vi "UHR-Fleezers Control (host) - 9.3.vi"() -> ()   [LabVIEW 2009]
uses:
  <vilib>/Utility/miscctls.llb/LVPoint32TypeDef.ctl
  <vilib>/Utility/miscctls.llb/LVMinMaxIncTypeDef.ctl
  <vilib>/userDefined/High Color/nirio_resource_hc.ctl
  <vilib>/Instr/_visa.llb/VISA Configure Serial Port (Instr).vi
  <vilib>/Platform/TimedLoop/XDataNode/XDataNode.xnode
  <vilib>/Platform/TimedLoop/XDataNode/loadlvalarms.vi
  <vilib>/Platform/TimedLoop/XDataNode/timing_clust.ctl
  <vilib>/Platform/TimedLoop/XDataNode/nitl_modes.ctl
  <vilib>/Platform/TimedLoop/XDataNode/wakeup.ctl
  <vilib>/rvi/interface/nirviOpenFPGA/nirviOpenFPGA.xnode
  FPGA Bitfiles/UHR-Fleezers Instr~3C_FPGA Target_UHR-Fleezers Contr~C3.lvbitx
  UHR-Fleezers Control (fpga) - 9.2.vi
  <vilib>/FPGAPlugInAG/PCIe-7852R/nirviIntfOpen_PCIe-7852R.vi
  <vilib>/rvi/interface/nirviMethod/nirviMethod.xnode
  <vilib>/Utility/error.llb/Merge Errors.vi
  <vilib>/LabVIEW Targets/FPGA/Rio/nirio_HostInterface/nirio_Reset.vi
  <vilib>/LabVIEW Targets/FPGA/Rio/nirio_HostInterface/nirio_DMAStopAll.vi
  <vilib>/rvi/interface/common/niFpgaNodeNameForErrorReporting.ctl
  <vilib>/rvi/errors/niLvFpgaWhatHappensToTopLevelVI.ctl
  <vilib>/LabVIEW Targets/FPGA/Rio/nirio_HostInterface/nirio_DisableInterrupts.vi
  <vilib>/Utility/error.llb/Error Cluster From Error Code.vi
  <vilib>/rvi/errors/niLvFpgaAdjustHostInterfaceError.vi
  <vilib>/rvi/interface/nirviReadWriteControl/nirviReadWriteControl.xnode
  <vilib>/LabVIEW Targets/FPGA/Rio/nirio_HostInterface/nirio_WriteBig.vi
  <vilib>/LabVIEW Targets/FPGA/Rio/nirio_HostInterface/nirio_DMAConfigure.vi
  <vilib>/LabVIEW Targets/FPGA/Rio/nirio_HostInterface/nirio_DMAStop.vi
  <vilib>/RVI Host/nirviSupport.llb/nirviErrorClusterFromErrorCode.vi
  <vilib>/LabVIEW Targets/FPGA/Rio/nirio_HostInterface/nirio_EnableInterrupts.vi
  <vilib>/rvi/errors/niLvFpgaReportInternalErrorWithAdditionalInfo.vi
  <vilib>/express/express analysis/Spectral/XNode/ExpressSpectralMeasurementsBlockNode.xnode
  <vilib>/express/express analysis/Spectral/Block/exnSpectralBlock spectral measurements PSD poly.vi
  <vilib>/express/express analysis/Spectral/Block/exnSpectralBlock spectral measurements PSD WFM.vi
  <vilib>/Waveform/WDTOps.llb/WDT Append Waveforms DBL.vi
  <vilib>/LabVIEW Targets/FPGA/Rio/nirio_HostInterface/nirio_ReadBig.vi
  <vilib>/vision/Avi1.llb/AviRefnum.ctl
  <vilib>/rvi/interface/nirviCloseFPGA/nirviCloseFPGA.xnode
  <vilib>/FPGAPlugInAG/PCIe-7852R/nirviIntfClose_PCIe-7852R.vi
  <vilib>/Analysis/NI_AALBase.lvlib
  <vilib>/Platform/TimedLoop/XDataNode/XDNodeRunTimeDep.lvlib
  openfpgaref.8.6.ctl
  NiRioSrv.dll
  <vilib>/vision/NI_Vision_Development_Module.lvlib
panel:
  in  "Force Reset":bool
  in  "Force Yank":bool
  in  "Random Choice":bool=TRUE
  in  "N Array El":u8=3 min=1 step=1
  in  "Yank to Delta Array (MHz)":dbl[](array[numeric])=[16.3, 15.85, 14.85]
  in  "Yank Delay (s)":dbl=3.5
  in  "N pts to average":u16=6
  out "Fl. High":bool
  out "Waiting":bool
  in  "Fl. Delta Thresh. (kHz)":dbl=0.6
  in  "Fl. Triggered...":bool
  in  "Action":string(combo)="Yank"
  out "Duration (s)":dbl
  out "Waveform Graph":dbl[](graph) caption="APD Line Scan"
  in  "Total Volume\nFlushed (uL)":dbl
  in  "Flush Center Channel":bool
  in  "Inject Pump 3 (D)":bool
  in  "Inject Pump 1 (DNA)":bool
  out "Messages":string
  in  "APD Ave N":dbl=10.0
  out "Int. Time (s)":dbl
  in  "Stop All":bool
  out "sigma/mean":dbl
  out "Rate sigma (Hz)":dbl format="%0.2f"
  out "Current Stage  Position":cluster{dbl, dbl, dbl}
  in  "Index":dbl=1.0 caption="Save File Index" min=1.0 step=1.0
  in  "Tab Control 6":T1(tab)=enum."Dual Display (Trap + APD)"
  out "All Signals":waveform(dbl)[](graph)
  in  "Signals to Plot":i32(listbox)
  out "Trap Disp. Freq. (Hz)":dbl caption="Freq. (Hz)" format="%#_6p"
  out "Display Period (s)":dbl caption="Period (s)" format="%#_6p"
  in  "Trap Disp. Downsample":dbl=20000.0 caption="Downsample"
  in  "APD Disp. Scale":dbl=0.1 caption="Scale (Divide,\nfor above plot only)"
  in  "APD Disp. Downsample":dbl=30.0 caption="Integrate" min=1.0 step=1.0
  out "APD Display Freq. (Hz)":dbl caption="Freq. (Hz)"
  out "APD Display Period (s)":dbl caption="Period (s)"
  out "RMS (Ang)":dbl format="%_2g"
  in  "Bead Sep. Int. Time (s)":dbl=5.0 caption="Int. Time (s)"
  in  "Below (kHz)":dbl=0.5
  in  "Above (kHz)":dbl=2.0
  in  "Adjust Scale\nto Mean":bool
  in  "Rescale on Mean":bool
  in  "Offset (nm)":dbl
  out "Mean":dbl caption="Mean (pN)" format="%#_3g"
  out "Force":waveform(dbl)[](graph)
  out "APD 1 Chart":waveform(dbl)(graph)
  in  "Calibration":u16(ring)=2 items=["None", "Position", "Force"]
  out "T1 X":dbl caption="T1 X (pN)" format="%0.2f"
  out "T2 X":dbl caption="T2 X (pN)" format="%0.2f"
  out "Bead Separation":waveform(dbl)(graph)
  in  "Amplitude (nm)":dbl=1.0
  out "Bead Mean (nm)":dbl caption="Mean (nm)" format="%0.2f"
  out "Difference":dbl caption="Difference (pN)" format="%.2g"
  out "APD 1 Graph":dbl[](graph) caption="Most Recent Time Trace"
  out "Trap Delta Graph":dbl[](graph) caption="Most Recent Time Trace"
  out "size(s) APD array":i32
  out "size(s) of 1 acq array":i32
  out "Delta Fl. (Hz)":dbl
  out "APD 1 Graph 2":dbl[](graph) caption="Most Recent Time Trace"
  in  "Flip Green Filter":bool
  in  "Set X Only":bool
  in  "Set Y Only":bool
  out "Detection Laser X":T2(plugin-control)
  out "APD 1":T2(plugin-control)
  out "Detection Laser Y":T2(plugin-control)
  out "Pointer Y (V)":dbl format="%_3g"
  out "Pointer X (V)":dbl format="%_3g"
  in  "Set Confocal Spot (X-Y)":bool
  out "FFT 1":cluster{"f0":dbl, "df":dbl, "magnitude":dbl[]}[](graph)
  out "FFT 2":cluster{"f0":dbl, "df":dbl, "magnitude":dbl[]}[](graph)
  in  "FFT 1 Choice 1":u16(ring) items=["T1 Y", "T1 X", "T1 Sum", "T2 Y", "T2 X", "T2 Sum", "T1 FB X", "T1 FB Sum", "T2 FB X", "T2 FB Sum", "PSD Y", "PSD X", "PSD Y Sum", "none"]
  in  "FFT 2 Choice 1":u16(ring)=13 items=["T1 Y", "T1 X", "T1 Sum", "T2 Y", "T2 X", "T2 Sum", "T1 FB X", "T1 FB Sum", "T2 FB X", "T2 FB Sum", "PSD Y", "PSD X", "PSD Y Sum", "none"]
  in  "FFT 1 Choice 2":u16(ring)=1 items=["T1 Y", "T1 X", "T1 Sum", "T2 Y", "T2 X", "T2 Sum", "T1 FB X", "T1 FB Sum", "T2 FB X", "T2 FB Sum", "PSD Y", "PSD X", "PSD Y Sum", "none"]
  in  "FFT 2 Choice 2":u16(ring)=13 items=["T1 Y", "T1 X", "T1 Sum", "T2 Y", "T2 X", "T2 Sum", "T1 FB X", "T1 FB Sum", "T2 FB X", "T2 FB Sum", "PSD Y", "PSD X", "PSD Y Sum", "none"]
  in  "Compute FFT":bool
  in  "Reset FFT":bool
  in  "# Spectra to Ave.":dbl=100.0
  out "Ave. Time (s)":dbl
  out "1 Channel":waveform(dbl)(graph)
  out "Slow mean":dbl format="%0.2f"
  in  "Slow mean N ave.":dbl=1.0 min=1.0 step=1.0
  out "Mean Intensity":dbl
  out "Sigma":dbl
  out "Sigma/Mean":dbl
  in  "Subtract mean":bool
  in  "High Res. Display":u16(ring) items=["T1 Y", "T1 X", "T1 Sum", "T2 Y", "T2 X", "T2 Sum", "T1 FB X", "T1 FB Sum", "T2 FB X", "T2 FB Sum", "PSD Y", "PSD X", "PSD Y Sum"]
  out "APD 1 Rate (Hz)":dbl format="%#_3p"
  out "Image":u32[][](graph)
  in  "Tab Control":T3(tab)=enum."Trap Control (RF)"
  in  "Lower Ch. Cap.":bool
  in  "With\nOffset":bool
  in  "Read Cal":bool
  out "Tether":bool
  in  "Tether Alarm?":bool=TRUE
  in  "Move to Delta (MHz)":dbl=14.85
  in  "Then...":string(combo)="4"
  in  "Data Acq. Spot":bool
  in  "Confocal Linescan":bool
  in  "Speed (nm/s)":dbl=100.0
  in  "Stop F (pN)":dbl=3.0
  in  "Furthest Withdraw (MHz)":dbl=15.0
  in  "Closest Delta (MHz)":dbl=10.25 step=0.25
  in  "Fish for Tether":bool
  in  "Confocal Image":bool
  in  "Round T1 X":bool caption="Round"
  in  "T1 offset_x (mV)":dbl=-26.302542012392074 format="%#_2g"
  in  "T1 kappa_x (pN/nm)":dbl=0.22546432407642192 min=0.0 step=0.001 format="%#_2g"
  out "Time (s)":dbl
  out "Total Time (s)":dbl
  in  "Start Saving":bool
  in  "Limits Enable":bool=TRUE caption="Enable"
  in  "Limit Max (MHz)":dbl=16.0 caption="Max (MHz)"
  in  "Limit Min (MHz)":dbl=10.0 caption="Min (MHz)"
  in  "Cal sets to save":u32=50 min=1 step=1
  in  "Comment (data description)":string="testing confocal setup"
  out "Calibrating Trap...":bool
  in  "Trap 2 (ON/OFF)":bool
  in  "Trap 1 (ON/OFF)":bool
  in  "Save Calibration":bool
  in  "N sets to save":u32=200 caption="N Sets"
  in  "Save N Sets":bool
  out "Save file name":path
  in  "Save ave N":dbl=500.0 caption="Averaging Factor"
  out "Saving...":bool
  in  "Stop Saving":bool
  out "Progress":u16(slide) scale=0.0..100.0
  out "Manipulating Trap":bool
  out "Buffer Status":dbl(slide) scale=0.0..1.0
  out "Overflow (data lost)":bool
  in  "Reset":bool
  out "Data Rate (Hz)":dbl caption="Trap Data Rate (Hz)" format="%#_3p"
  out "Data Period (s)":dbl caption="Trap Data Period (s)" format="%#_6p"
  out "Save Data Rate (Hz)":dbl caption="Rate (Hz)" format="%#_6p"
  out "Save Data Period (s)":dbl caption="Period (s)" format="%#_6p"
  in  "T1 alpha_x (nm/V)":dbl=630.439304367558 step=10.0 format="%#_3g"
  in  "T2 alpha_x (nm/V)":dbl=704.7738222964198 step=10.0 format="%#_3g"
  in  "T2 kappa_x (pN/nm)":dbl=0.2030110880477556 min=0.0 step=0.001 format="%#_2g"
  in  "T2 offset_x (mV)":dbl=-26.67973517613748 format="%#_2g"
  in  "BD 1 Frequency 1 (MHz)":dbl=70.15 caption="T1 X (MHz)" min=60.0 max=90.0 step=1.0 format="%#_6p"
  in  "BD 1 Frequency 2 (MHz)":dbl=85.0 caption="T2 X (MHz)" min=60.0 max=90.0 step=1.0 format="%#_6p"
  in  "Green Laser ON/Interlacing":bool
  in  "Round T2 X":bool caption="Round"
  in  "AO1":dbl(slide)=5.61 caption="Confocal Y (V)" min=0.0 max=10.0 step=0.01 scale=0.0..10.0 scale format="%_1f"
  in  "AO2":dbl(slide)=3.9 caption="Confocal X (V)" min=0.0 max=10.0 step=0.01 scale=0.0..10.0 scale format="%_1f"
  in  "Upper Cap.":bool
  in  "Lower Cap.":bool
  in  "Trap Raster Scan":bool
  out "Raster Scanning...":bool
  in  "Trap Delta (MHz)":dbl=14.85
  in  "Dump Beads":bool
  out "Stage Moving":bool
  in  "Wait Before Save (s)":u32=1
  out "Attempts":dbl
  in  "Attempt Limit":dbl=30.0 caption="Limit"
  in  "Array":dbl[][](array[numeric])
  in  "Move to Position 5":bool
  in  "Position 5 Label":string="Lower channel capillary"
  in  "z nudge increment (um)":dbl=0.5
  in  "+z":bool
  in  "Saved Stage Positions":T4={"Position 1"={1.04712, -0.65049, 0.0}, "Position 2"={0.0, 0.0, 0.0}, "Position 3"={2.99364, -0.33706, 0.0}, "Position 4"={2.1058, 0.57485, 0.0}, "Position 5"={3.01039, 3.32514, 0.03555}} {"Position 5"."?" min=-0.1 max=0.1 step=0.1; "Position 1"."?" min=-0.1 max=0.1 step=0.1; "Position 2"."?" min=-0.1 max=0.1 step=0.1; "Position 3"."?" min=-0.1 max=0.1 step=0.1; "Position 4"."?" min=-0.1 max=0.1 step=0.1}
  in  "Position 1 Label":string="Upper capillary"
  in  "Set Position 1":bool
  in  "Set Position 2":bool
  in  "Set Position 3":bool
  in  "Set Position 4":bool
  in  "Move to Position 3":bool
  in  "Move to Position 4":bool
  in  "Move to Position 2":bool
  in  "Move to Position 1":bool
  in  "Position 2 Label":string="Lower capillary"
  in  "Position 3 Label":string="Measurement spot"
  in  "Position 4 Label":string="Dump beads"
  in  "-z":bool
  in  "Set Position 5":bool
  in  "Top Ch Inject Rate (ul/h)":dbl=10.0
  in  "Pump write delay (ms)":dbl=300.0
  in  "All Pump Parameters":T5={"Pump 1"={"Diameter (mm)"=4.61, "Units"=3.0, "Volume"=0.0, "Rate"=0.0}, "Pump 2"={"Diameter (mm)"=4.61, "Units"=3.0, "Volume"=0.0, "Rate"=0.0}, "Pump 3"={"Diameter (mm)"=4.61, "Units"=3.0, "Volume"=0.0, "Rate"=0.0}}
  in  "Top Ch Inject Volume (uL)":dbl=100.0
  in  "Pump pause delay (ms)":u32
  in  "Bottom Ch Inject Volume (uL)":dbl=100.0
  in  "Bottom Ch Inject Rate (ul/h)":dbl=10.0
  in  "Flush Center Ch Volume (uL)":dbl=15.0
  in  "Flush Center Ch Rate (ul/m)":dbl=100.0
  in  "Tab Control 2":T6(tab)=enum."AOD Raster Scan"
  out "Total Counts (ticks)":u32
  in  "Trap ON/OFF X or Y Amp?":bool=TRUE
  in  "Oscillate Set 1":bool
  in  "Trap 1 ON":bool
  in  "Number Interlace Sets":u8=3 min=1 max=3
  in  "DIO count 3 (ticks)":u32=200
  in  "DIO count 2 (ticks)":u32=200
  in  "DIO count 1 (ticks)":u32=200
  in  "BD 2 Amplitude 3 (%)":dbl min=0.0 max=50.0 step=1.0
  in  "BD 2 Amplitude 2 (%)":dbl min=0.0 max=50.0 step=1.0
  in  "BD 2 Amplitude 1 (%)":dbl min=0.0 max=50.0 step=1.0
  in  "BD 1 Amplitude 3 (%)":dbl min=0.0 max=50.0 step=1.0
  in  "BD 1 Amplitude 2 (%)":dbl=35.0 min=0.0 max=50.0 step=1.0
  in  "BD 1 Amplitude 1 (%)":dbl=10.0 min=0.0 max=50.0 step=1.0
  in  "BD 2 Frequency 3 (MHz)":dbl=26.0 min=0.0 max=40.0 step=1.0 format="%#_6p"
  in  "BD 1 Frequency 3 (MHz)":dbl=70.0 min=60.0 max=90.0 step=1.0 format="%#_6p"
  in  "BD 2 Frequency 2 (MHz)":dbl=26.0 min=0.0 max=40.0 step=1.0 format="%#_6p"
  in  "BD 2 Frequency 1 (MHz)":dbl=26.0 min=0.0 max=40.0 step=1.0 format="%#_6p"
  in  "Not-Interlacing Set":enum32{"Set 1", "Set 2", "Set 3"}(radio)
  in  "Interlace":bool=TRUE
  in  "Trap 2 ON":bool
  in  "Trap 3 ON":bool
  in  "Scan axis 2":bool=TRUE
  in  "Osc. freq. (Hz)":dbl=0.25
  in  "Osc. amp. (MHz)":dbl=2.0
  out "Coords":T7
  in  "Manipulation Scaling":cluster{"Horizontal":dbl, "Vertical":dbl}={"Horizontal"=0.075, "Vertical"=0.01}
  in  "Freq or Amp switch first":bool=TRUE
  in  "Swap F1 and F2":bool
  in  "Freq switch delay":u16
  in  "Amp switch delay":u16=5
  in  "MCL Step Increment (V_int)":dbl=3.0
  out "Time to Finish All (min)":dbl format="%#_2p"
  in  "Scan Speed (nm/s)":dbl=100.0
  in  "Scan Range (nm)":dbl=200.0
  in  "Step Size (nm)":dbl=1.0
  in  "MCL/AOM Scale Tweak":dbl=1.0
  in  "MCL Step Position Ratio":dbl=0.5
  in  "Move MCL Also?":bool=TRUE
  out "Final sep (nm)":dbl
  out "Initial sep (nm)":dbl
  out "Save index":dbl
  out "Final delta (MHz)":dbl
  out "Initial delta (MHz)":dbl
  out "Final freq. (MHz)":dbl
  out "Initial freq. (MHz)":dbl
  in  "Saved AOD Raster Scan Parameter Sets":T8(array[cluster])=[{"Scan Range AOD (nm) 2"=500.0, "Step Size AOD (nm) 2"=1.0, "Scan Speed AOD (nm/s) 2"=200.0, "Number of scans (AOD) 2"=1, "Label"=""}, {"Scan Range AOD (nm) 2"=1000.0, "Step Size AOD (nm) 2"=1.0, "Scan Speed AOD (nm/s) 2"=200.0, "Number of scans (AOD) 2"=5, "Label"="wide offset scan"}, {"Scan Range AOD (nm) 2"=20.0, "Step Size AOD (nm) 2"=0.68, "Scan Speed AOD (nm/s) 2"=0.68, "Number of scans (AOD) 2"=1, "Label"="2 bp steps"}]
  in  "Load parameters":bool
  out "Scan Range (MHz)":dbl=10.0
  in  "Restart DMA? (AOD)":bool=TRUE caption="Restart DMA?"
  out "Incr. int (AOD)":i64
  out "Time/Scan (s) (AOD)":dbl format="%#_2p"
  out "Data points/scans":dbl
  out "Data points/scan (f/b)":dbl
  in  "Save scans":bool=TRUE
  out "AOD Scan I":u64 caption="Scan I"
  in  "Continuous AOD Scanning":bool caption="Continuous Scanning"
  in  "Abort AOD Scan":bool caption="Abort Scan"
  in  "Scan BD":bool=TRUE
  out "Cycles/step (AOD)":u64=400 format="%.0p"
  in  "Number of F/B Scans (AOD)":u16=3 min=1
  out "Scan steps (AOD)":u64=1000
  out "Scan Increment (MHz)":dbl=0.2
  out "AOD Scanning":bool caption="Scanning"
  in  "Start AOD Scan":bool caption="Start Scan"
  out "N sets should be saved":dbl
  out "Progress 2":u16(slide) caption="Progress" scale=0.0..100.0
  in  "Abort save 2":bool caption="Abort save"
  in  "Trap 1 Bead Size (nm)":dbl=860.0
  in  "Trap 2 Bead Size (nm)":dbl=790.0
  out "MCL Count":dbl
  in  "All FB On/Off":bool=TRUE
  in  "AI2 to Setpoint":cluster{"Set 1":bool, "Set 2":bool}
  out "AI2 (V)":cluster{"Set 1":dbl, "Set 2":dbl}
  in  "Reset Feedback":cluster{"Set 1":bool, "Set 2":bool}
  in  "PID Gains":T9={"Set 1"={"proportional gain (Kc)"=0, "integral gain (Kc*Ts/Ti)"=5, "derivative gain (Kc*Td/Ts)"=0}, "Set 2"={"proportional gain (Kc)"=0, "integral gain (Kc*Ts/Ti)"=5, "derivative gain (Kc*Td/Ts)"=0}}
  in  "Setpoints (V)":cluster{"Set 1":dbl, "Set 2":dbl}={"Set 1"=9.0, "Set 2"=9.0}
  in  "Feedback On/Off":cluster{"Set 1":bool, "Set 2":bool}={"Set 1"=TRUE, "Set 2"=TRUE}
  in  "Tab Control 3":enum32{"Timing", "MCL Scan", "Analog Out"}(tab)=enum."MCL Scan"
  out "APD Gate Late Counter":u32
  in  "- phase (APD Gate)":bool
  in  "+ phase (APD Gate)":bool
  out "APD Gate Relative Phase":i16
  in  "Phase Adj. (APD Gate)":i16=20
  in  "Initial Phase Adjustment (APD Gate)":i16=50
  in  "Save APD Data\nwith Trap Data":bool=TRUE
  out "APD FIFO Elements Remaining":u32
  in  "- phase (APD Acq)":bool
  in  "+ phase (APD Acq)":bool
  out "APD Acq Late Counter":u32
  out "APD Acq Relative Phase":i16
  in  "Phase Adj. (APD Acq)":i16=20
  in  "Initial Phase Adjustment (APD Acq)":i16
  in  "Invert APD Gate":bool caption="Invert Gate"
  in  "APD Gate OFF Count":u32=450 caption="Gate OFF Count"
  in  "APD Gate ON Count":u32=150 caption="Gate ON Count"
  in  "APD Gate":enum32{"ON", "OFF", "Interlace"}(radio)=enum."Interlace"
  in  "APD Integration Time (s)":dbl=0.01 caption="Integration Time (s)"
  out "APD Acq Rate (Hz)":dbl=20000000.0 caption="Rate (Hz)"
  out "APD Samples/FIFO Acq.":dbl
  out "APD Elements/DMA read":u32
  out "APD Int. Count":u32 format="%.0p"
  in  "Tab Control 5":enum32{"PSD X", "PSD Y", "Other Data Channel"}(tab)
  out "Data map":dbl[][](graph)
  in  "Channel":i32=4
  in  "Abort MCL Scan":bool
  out "MCL Scan I":u64
  out "MCL Scanning":bool
  in  "Start MCL Scan":bool
  out "wait to reset values":bool
  in  "Tab Control 4":enum32{"Scan Settings", "MCL FPGA Loop Timing"}(tab)
  out "Total Time (s)":dbl
  in  "Scan lines (y)":u64=20
  in  "Fast Scan Dir":bool=TRUE
  in  "2D or 1D Scan":bool=TRUE
  out "Initial X":dbl
  out "Initial Y":dbl
  out "Time/f+b scan (s) (MCL)":dbl caption="Time/scan (s)"
  in  "Number of scans (MCL)":u64=1 caption="Scans"
  in  "Scan steps (MCL)":u64=40 caption="Scan steps (x)"
  in  "N APD Samp/step":dbl=3.0
  in  "Scan Range (V)\n(of steps)":dbl=3.5
  in  "Restart DMA? (MCL)":bool=TRUE caption="Restart DMA?"
  in  "Continuous MCL Scanning":bool caption="Cont. Scanning"
  in  "Center Scan":bool=TRUE
  in  "Save Data (MCL)":bool=TRUE caption="Save Data"
  out "Actual Incr. int (MCL)":i16 caption="Incr. int"
  out "Desired incr (int)":dbl
  out "Desired Scan Incr (V)":dbl
  out "N sets should be saved (MCL)":dbl caption="N sets should be saved"
  out "Data points/scans (MCL)":dbl caption="Data points/scans"
  out "Data points/scan (f+b)":dbl caption="points/scan (f+b)"
  out "Cycles/step (MCL)":u64 caption="Cycles/step" format="%.0p"
  out "Actual MCL Inc (V)":dbl
  in  "Phase adjust (MCL)":i16 caption="Phase adjust"
  out "Relative Phase (MCL)":i16 caption="Relative Phase"
  in  "Initial Phase Adj. (MCL)":i16 caption="Initial Phase Adj."
  in  "Update Count (MCL)":u32=600
  in  "+ phase (MCL)":bool
  in  "- phase (MCL)":bool
  out "MCL Late Counter":u32
  in  "APD 1 AO Mult.":i16=1 min=1
  in  "APD 2 AO Mult.":i16=1 min=1
  in  "APD 1 AO offset":i16
  in  "APD 2 AO offset":i16
  in  "Tab Control 7":enum32{"Green FB Signals", "Slow MCL Scan"}(tab)
  out "Green FB Plot":dbl(graph)
  out "MCL Scan 2":cluster{"Begin (V)":dbl, dbl, dbl[]}(graph)
  out "MCL Scan":cluster{"Begin (V)":dbl, dbl, dbl[]}(graph)
  in  "Green laser mode":enum32{"Laser ON", "Laser OFF", "Interlace"}(radio)=enum."Interlace"
  in  "GI Frequency, ON count":u32=150 min=1 step=1
  in  "Invert GI":bool
  out "GI Late Counter":u32
  in  "Phase adj. (GI)":i16=5
  out "GI relative phase":i16
  in  "+ phase (GI)":bool
  in  "Initial Phase Adjustment (GI)":i16=15
  in  "GI Frequency, OFF count":u32=450 min=1 step=1
  in  "- phase (GI)":bool
  out "Green FB Signals (V)":cluster{"Y":dbl, "X":dbl, "Sum":dbl}
  out "Relative phase (Green FB)":i16
  in  "+ phase (Green FB)":bool
  in  "- phase (Green FB)":bool
  in  "Green FB Count":u32=600
  in  "Phase adj. (Green FB)":i16=10
  in  "Initial Phase Adjustment (Green FB)":i16=50
  in  "Green FB On/Off":bool=TRUE
  in  "Current When FB OFF (%)":dbl=87.0 min=0.0 max=100.0 step=1.0
  in  "Green int current ON count adj":u32=150
  in  "Green FB Gains":T10={"proportional gain (Kc)"=10, "integral gain (Kc*Ts/Ti)"=5, "derivative gain (Kc*Td/Ts)"=0}
  in  "Green FB Setpoint (mV)":dbl=100.0
  in  "- phase (GI) 2":bool
  in  "Initial Phase Adjustment (GI) 2":i16=-100
  in  "+ phase (GI) 2":bool
  out "GI relative phase 2":i16
  in  "Phase adj. (GI) 2":i16=20
  out "GI Late Counter 2":u32
  in  "# Samples/trap":dbl=20000.0 format="%#_6p"
  out "Elements/DMA read":u32 format="%.0p"
  out "Ave. Rate (Hz)":dbl format="%#_6p"
  out "FIFO El. Rem.":u32 format="%.0p"
  in  "Phase adj. (AI1)":i16=15
  out "Relative phase (AI1)":i16
  in  "+ phase (AI1)":bool
  in  "- phase (AI1)":bool
  out "Late Counter (AI1)":u32
  in  "Initial Phase Adjustment (AI1)":i16=220
  out "AI rate (Hz)":dbl=50000.0 format="%#_6p"
  in  "AI Count (ticks)":u32=200
  out "# Samples/channel":u32=20000 format="%.0p"
  in  "FIFO Depth":u32=600000 format="%.0p"
  in  "Detector Type":string(combo)="IR-QPD + PSD + FB-QPD X position"
  in  "N Acq Sets (Traps + Fl.)":i16=3
  in  "Sets to FIFO (Traps)":T11={"Set 1"=TRUE, "Set 2"=TRUE, "Set 3"=FALSE}
  in  "FPGA Ave.":dbl=1.0 min=1.0 step=1.0
  out "Ave. Period (s)":dbl format="%#_6p"
  out "DMA Update Period (s)":dbl
  out "FPGA Averaging":bool
  out "Trap Sets":i16
  out "Counts/DMA":dbl format="%#_6p"
  in  "Video Capture Rate (Hz)":dbl=30.0
  in  "Video Index":dbl=1.0 min=1.0 step=1.0
  in  "New Video File":bool
  in  "Capture Video":bool
  in  "Reset Averaging":bool
  in  "Averaging":bool
  in  "Capture and Save Image":bool
  in  "Image Index":dbl=1.0 min=1.0
  out "Path Out":path
  in  "Center Point":cluster{"X":i32, "Y":i32}={"X"=335, "Y"=271}
  in  "Zoom Factor":sgl=7.0
  out "Window Size":cluster{"Width":i32, "Height":i32}
  out "Window Position":cluster{"X Position":i32, "Y Position":i32}={"X Position"=40, "Y Position"=40}
  in  "Initial Window Size":cluster{"Width":i32, "Height":i32}={"Width"=884, "Height"=619}
  in  "Initial Window Position":cluster{"X Position":i32, "Y Position":i32}={"X Position"=796, "Y Position"=4}
  in  "Intensity Upper":u8=88
  in  "Intensity Lower":u8=66
  out "error out":errorcluster
  out "error out 2":errorcluster
  in  "Lost Tether Alarm Threshold (pN)":dbl=0.5
  in  "AOM X Cal (nm/MHz)":dbl=123.0
  in  "MCL X Cal (nm/V)":dbl=1070.0
  out "X RF Amplitude Limits (%)":T12={"Minimum"=0.0, "Maximum"=50.0, "Increment"=1.0}
  out "X RF Frequency Limits (MHz)":T12={"Minimum"=60.0, "Maximum"=90.0, "Increment"=1.0}
  out "Y RF Frequency Limits (MHz)":T12={"Minimum"=60.0, "Maximum"=90.0, "Increment"=1.0}
  out "Y RF Amplitude Limits (%)":T12={"Minimum"=0.0, "Maximum"=50.0, "Increment"=1.0}
  in  "Manip. X?":bool=TRUE
  in  "Manip. Y?":bool
  in  "Force Manip Abort":bool
  out "Read cal error":errorcluster
  in  "DAQ Delay (ms)":u32=1000
  in  "Start Scan":bool
  in  "Scan axis":bool=TRUE
  in  "Osc. amp. (V)":dbl=5.0
  in  "Osc. center (V)":dbl=5.0
  in  "Osc. freq. (Hz) 2":dbl=1.0
  in  "MCL Mode":u16(ring) items=["Manual Positioning", "Sinusoidal Wave", "Linear Scan"]
  in  "Begin (V)":dbl
  in  "End (V)":dbl=10.0
  in  "N Points":dbl=20.0
  in  "Delay to Interlace (s)":dbl
  in  "Delayed Interlace Start":bool
  in  "Read Lateness and Rel Phase":bool
  out "Vec Mean of T1 T2":dbl[](array[numeric])
  in  "Cal read wait (s)":u32=5
  out "Time tether formed":timestamp
  in  "Sample Chamber Stage Serial Port":refnum<visa-resource-name>="ChamberStageCOM4"
  in  "Syringe Pump Serial Port":refnum<visa-resource-name>="ChemyxPumpCOM3"
  # "Trap Display:"
  # "APD Display:"
  # "DAQ"
  # "Move Stage and Take Action"
  # "Trap Manipulation"
  # "Data Saving"
  # "Bead Calibration"
  # "Trap Position Difference Limits"
  # "DNA Beads"
  # "ADig Beads"
  # "Center channel"
  # "Units: \n1 = ml/m\n2 = ml/h\n3 = ul/m\n4 = ul/h"
  # "Rate param is ul/h\nVolume param is ul"
  # "X"
  # "Y"
  # "Oscillate Set 1 freq. (debugging)"
  # "BD 1"
  # "BD 2"
  # "AOD Raster Scan"
  # "Approx. trap separations"
  # "X"
  # "Y"
  # "Gate"
  # "X"
  # "2D"
  # "Y"
  # "1D"
  # "Green Laser Interlacing"
  # "Green FB Measurement"
  # "Digital Gate"
  # "Current Analog Control"
  # "Total AI Rates (NOT rates/trap)"
  # "(Samples/trap x Trap Sets)"
  # "(Samples/channel x\n8 if averaging (8 channels)\n4 if no averaging)"
  # "Trap 1"
  # "Trap 2"
  # "Flour./Trap 3"
  # "External Video Window"
  # "MCL Position Debugging"
  # "Temporary Control Storage\n(these used to be somewhere else, still want to keep them)"
  # "Y"
  # "X"
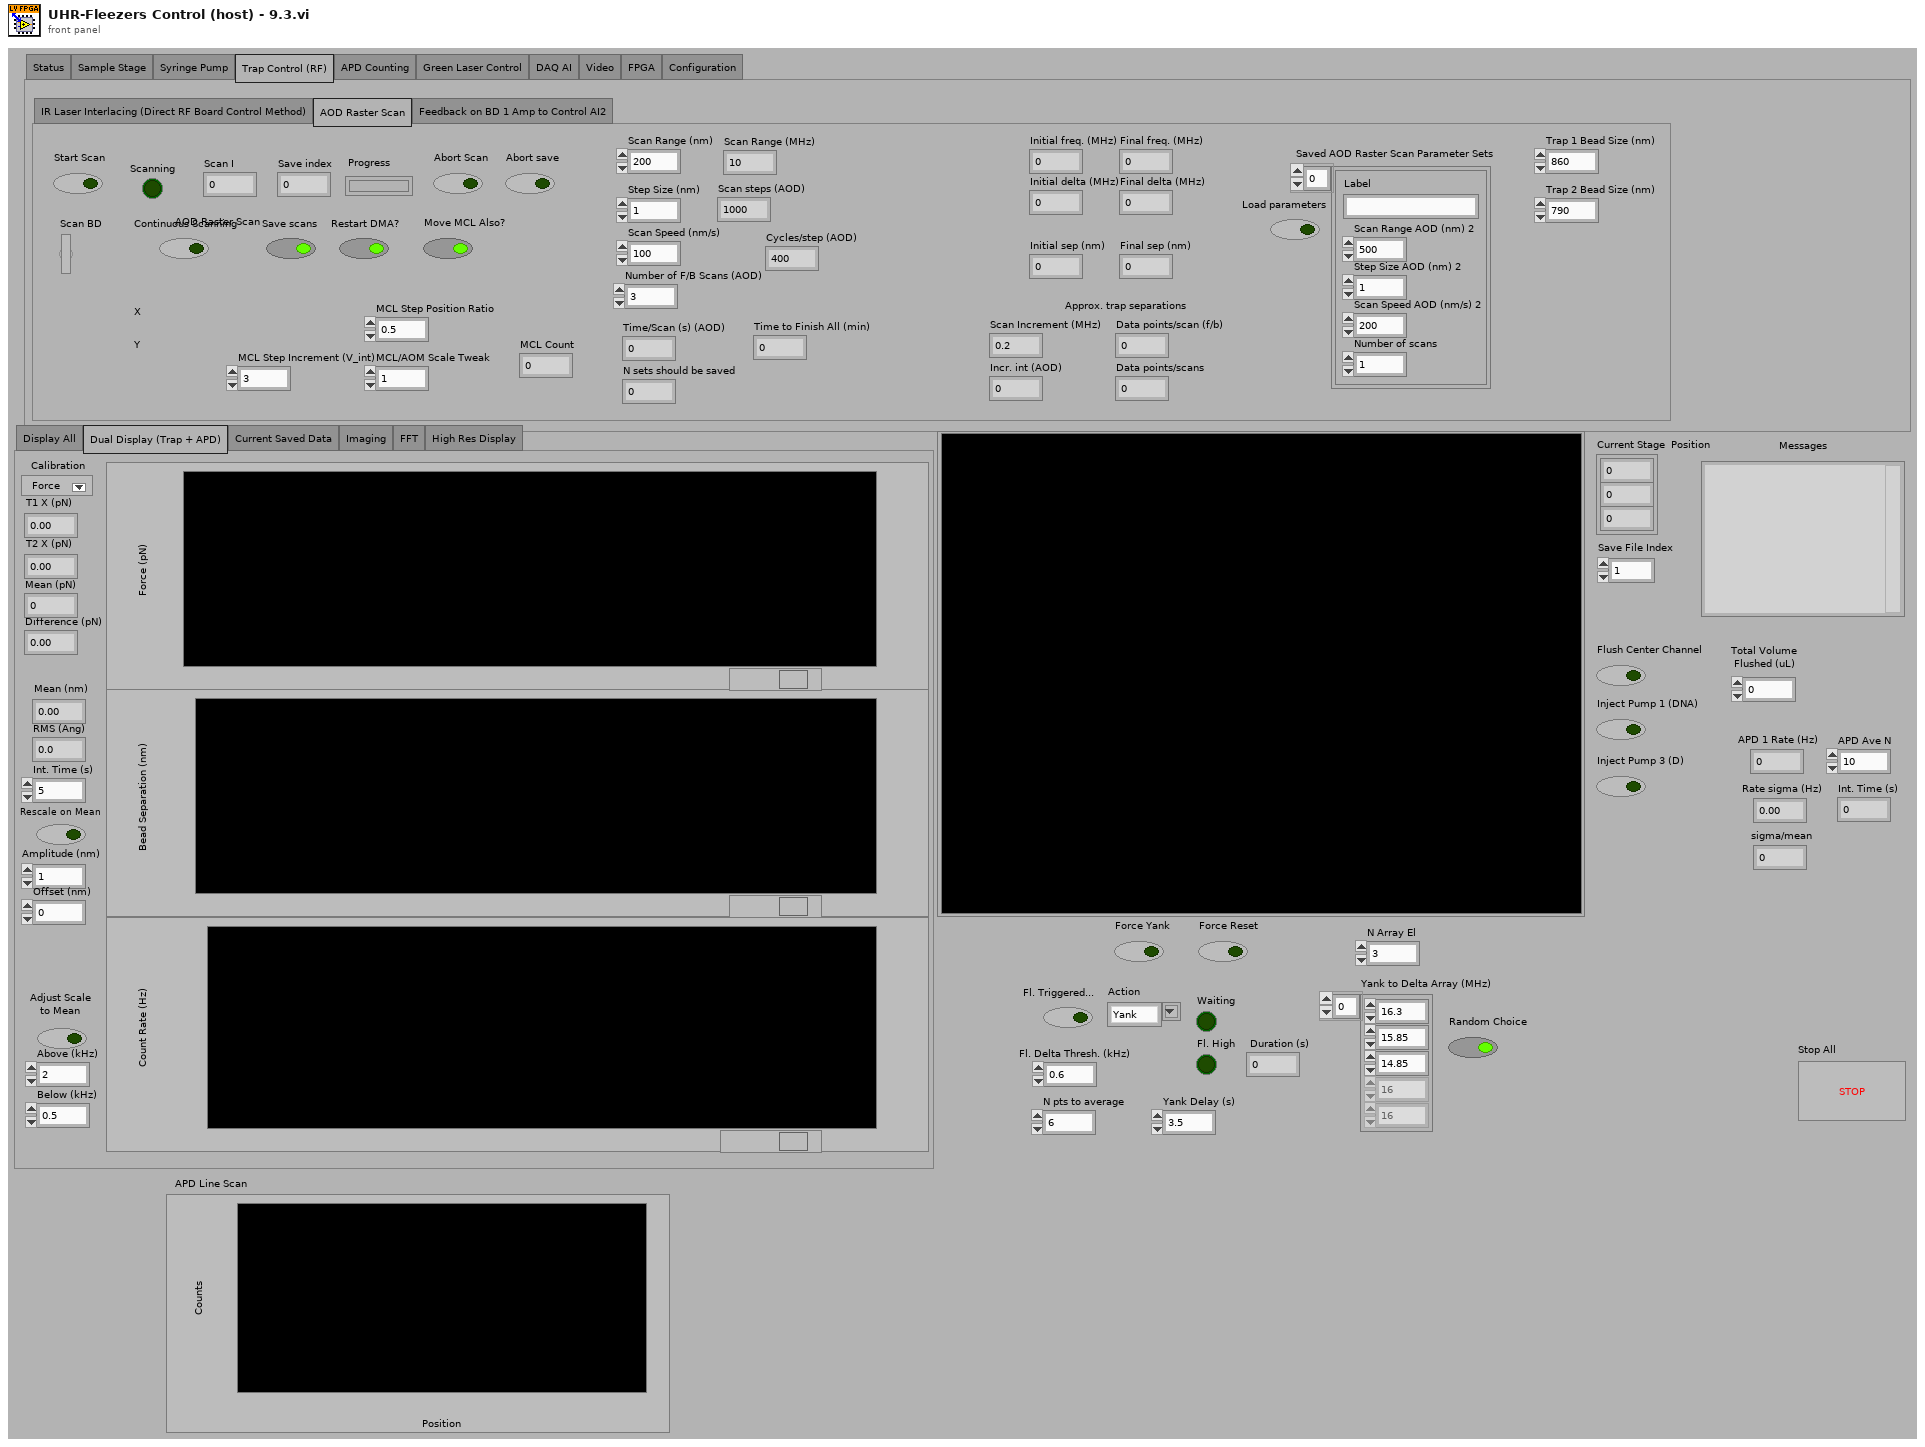
[diagram p1: front panel]
types:
  T1 = enum32{"Display All", "Dual Display (Trap + APD)", "Current Saved Data", "Imaging", "FFT", "High Res Display"}
  T2 = typedef "IMAQ Image.ctl" = refnum<image>
  T3 = enum32{"Status", "Sample Stage", "Syringe Pump", "Trap Control (RF)", "APD Counting", "Green Laser Control", "DAQ AI", "Video", "FPGA", "Configuration"}
  T4 = cluster{"Position 1":cluster{dbl, dbl, dbl}, "Position 2":cluster{dbl, dbl, dbl}, "Position 3":cluster{dbl, dbl, dbl}, "Position 4":cluster{dbl, dbl, dbl}, "Position 5":cluster{dbl, dbl, dbl}}
  T5 = cluster{"Pump 1":cluster{"Diameter (mm)":dbl, "Units":dbl, "Volume":dbl, "Rate":dbl}, "Pump 2":cluster{"Diameter (mm)":dbl, "Units":dbl, "Volume":dbl, "Rate":dbl}, "Pump 3":cluster{"Diameter (mm)":dbl, "Units":dbl, "Volume":dbl, "Rate":dbl}}
  T6 = enum32{"IR Laser Interlacing (Direct RF Board Control Method)", "AOD Raster Scan", "Feedback on BD 1 Amp to Control AI2"}
  T7 = typedef "LVPoint32TypeDef.ctl" = cluster{"Horizontal":i32, "Vertical":i32}
  T8 = cluster{"Scan Range AOD (nm) 2":dbl, "Step Size AOD (nm) 2":dbl, "Scan Speed AOD (nm/s) 2":dbl, "Number of scans (AOD) 2":u16, "Label":string}[]
  T9 = cluster{"Set 1":cluster{"proportional gain (Kc)":i16, "integral gain (Kc*Ts/Ti)":i16, "derivative gain (Kc*Td/Ts)":i16}, "Set 2":cluster{"proportional gain (Kc)":i16, "integral gain (Kc*Ts/Ti)":i16, "derivative gain (Kc*Td/Ts)":i16}}
  T10 = cluster{"proportional gain (Kc)":i16, "integral gain (Kc*Ts/Ti)":i16, "derivative gain (Kc*Td/Ts)":i16}
  T11 = cluster{"Set 1":bool, "Set 2":bool, "Set 3":bool}
  T12 = typedef "LVMinMaxIncTypeDef.ctl" = cluster{"Minimum":dbl, "Maximum":dbl, "Increment":dbl}
  T13 = typedef "Image Type" = u32
  T14 = typedef "nirio_resource_hc.ctl" = tag
  T15 = typedef "openfpgaref.8.6.ctl" = refnum<k20>
  T16 = typedef "niFpgaNodeNameForErrorReporting.ctl" = enum16{"Open FPGA VI Reference", "Read/Write Control", "Invoke Method: Abort", "Invoke Method: Acknowledge IRQ", "Invoke Method: Download", "Invoke Method: FIFO.Configure", "Invoke Method: FIFO.Read", "Invoke Method: FIFO.Start", "Invoke Method: FIFO.Stop", "Invoke Method: FIFO.Write", "Invoke Method: Reset", "Invoke Method: Run", "Invoke Method: Wait on IRQ", "Close FPGA VI Reference"}
  T17 = typedef "niLvFpgaWhatHappensToTopLevelVI.ctl" = enum16{"top level VI scripted behind XNode", "top level VI inlined behind XNode"}
  T18 = typedef "XDNodeRunTimeDep.lvlib/timing_clust.ctl" = cluster{"Expected End [f-1]":u64, "Actual End [f-1]":u64, "Finished Late? [f-1]":bool, "Expected End [i-1]":u64, "Actual End [i-1]":u64, "Finished Late? [i-1]":bool, "Expected Start [i]":u64, "Actual Start [i]":u64, "Expected Start [f]":u64, "Actual Start [f]":u64, "Source Name":string, "Structure Name":string, "Period":i64, "Deadline":i64, "Offset":i64, "Start":i64, "Priority":i32, "Timeout":i32, "Mode":T19, "Wakeup Reason":T20, "Error":errorcluster, "Source Type":string, "Secondary Source Type":string, "Global End Time":u64, "Global Start Time":u64, "Frame Duration":u64, "Iteration Duration":u64, "Assigned CPU":i32, "I/O Scan Engine Mode":u32}
  T19 = typedef "XDNodeRunTimeDep.lvlib/nitl_modes.ctl" = enum32{"No Change", "Process missed periods, maintain original phase", "Discard missed periods, maintain original phase", "Process missed periods, ignore original phase", "Discard missed periods, ignore original phase"}
  T20 = typedef "XDNodeRunTimeDep.lvlib/wakeup.ctl" = enum32{"Normal", "Aborted", "Asynchronous wakeup", "Timing source error", "Timed loop error", "Timeout"}
  T21 = enum16{"big-endian, network order", "native, host order", "little-endian"}
  T22 = enum16{"open", "replace", "create", "open or create", "replace or create", "replace or create with confirmation"}
  T23 = cluster{"Scan Range AOD (nm) 2":dbl, "Step Size AOD (nm) 2":dbl, "Scan Speed AOD (nm/s) 2":dbl, "Number of scans (AOD) 2":u16, "Label":string}
  T24 = cluster{"[0]":dbl, "[1]":dbl, "[2]":dbl, "[3]":dbl, "[4]":dbl, "[5]":dbl}
  T25 = cluster{"Diameter (mm)":dbl, "Units":dbl, "Volume":dbl, "Rate":dbl}
  T26 = cluster{"Left":i32, "Top":i32, "Width":u32, "Height":u32}
  T27 = cluster{cluster{"Left":i32, "Top":i32, "Width":u32, "Height":u32}}[]
  T28 = enum32{"setting", "request", "request control", "info", "statistics", "system settings", "I/O sub system", "HRT control", "camera descriptions", "device specific data", "event sub system settings", "event sub system results", "image memory manager"}
  T29 = typedef "AviRefnum.ctl" = refnum<k1>
  T30 = typedef "imagedata.ctl" = cluster{"image type":i32, "image depth":i32, "image":u8[], "mask":u8[], "colors":u32[], "Rectangle":cluster{"left":i16, "top":i16, "right":i16, "bottom":i16}}
  T31 = enum32{"Normal Display", "Dual Display (APD)", "FFT", "High Res Display"}
  T32 = cluster{"Origin Pixel":cluster{"X":sgl, "Y":sgl}, "Angle Relative to Horizontal (deg)":sgl, "Axis Reference":u32}
  T33 = typedef "Simple Grid Descriptor" = cluster{"X Step":sgl, "Y Step":sgl, "Unit":T34}
  T34 = typedef "Image Unit" = enum32{"Undefined", "Angström", "Micrometer", "Millimeter", "Centimeter", "Meter", "Kilometer", "Microinch", "Inch", "Feet", "Nautical miles", "Standard miles", "Steps"}
  T35 = cluster{"averaging mode":u16, "weighting mode":u16, "number of averages":u32}
  T36 = cluster{"dB On (F)":bool, "unwrap phase (F)":bool, "convert to degree (F)":bool}
  T37 = cluster{"Green FB Ch 0":i16, "Green FB Ch 1":i16, "Green FB Ch 2":i16}
  T38 = cluster{string, string, string, string, string, string, string, string}
  T39 = cluster{string, string, string, string, string, string, string, string, string, string, string, string}
  T40 = cluster{string, string, string, string, string, string, string, string, string, string, string, string, string}
  T41 = cluster{string, string, string, string, string, string, string, string, string, string, string, string, string, string}
  T42 = cluster{"f0":dbl, "df":dbl, "magnitude":dbl[]}[][]
  T43 = cluster{"Green FB Ch 0":dbl, "Green FB Ch 1":dbl, "Green FB Ch 2":dbl}
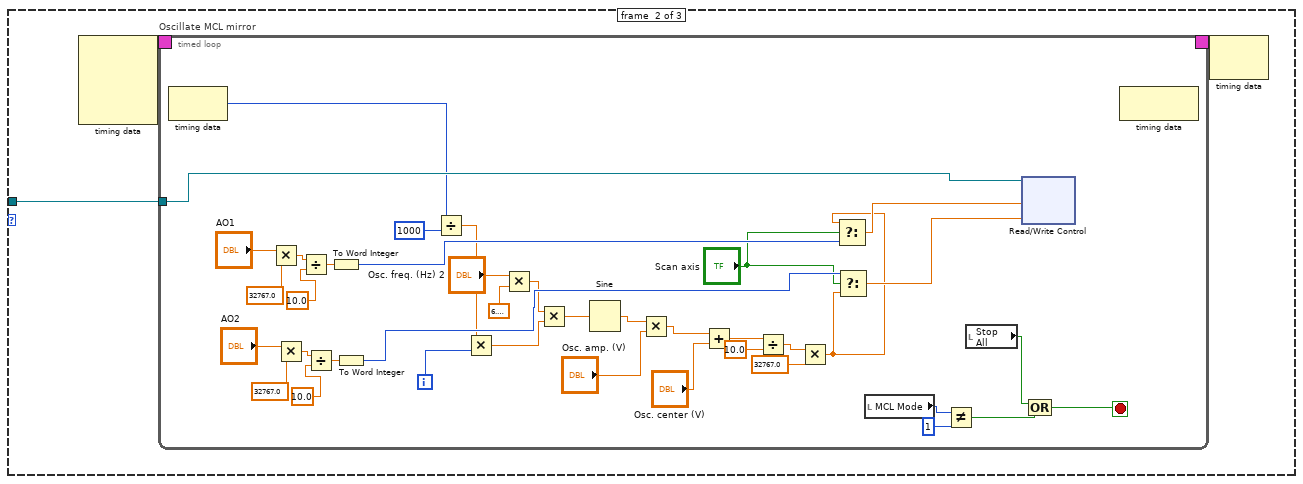
[diagram p2: hidden frame]
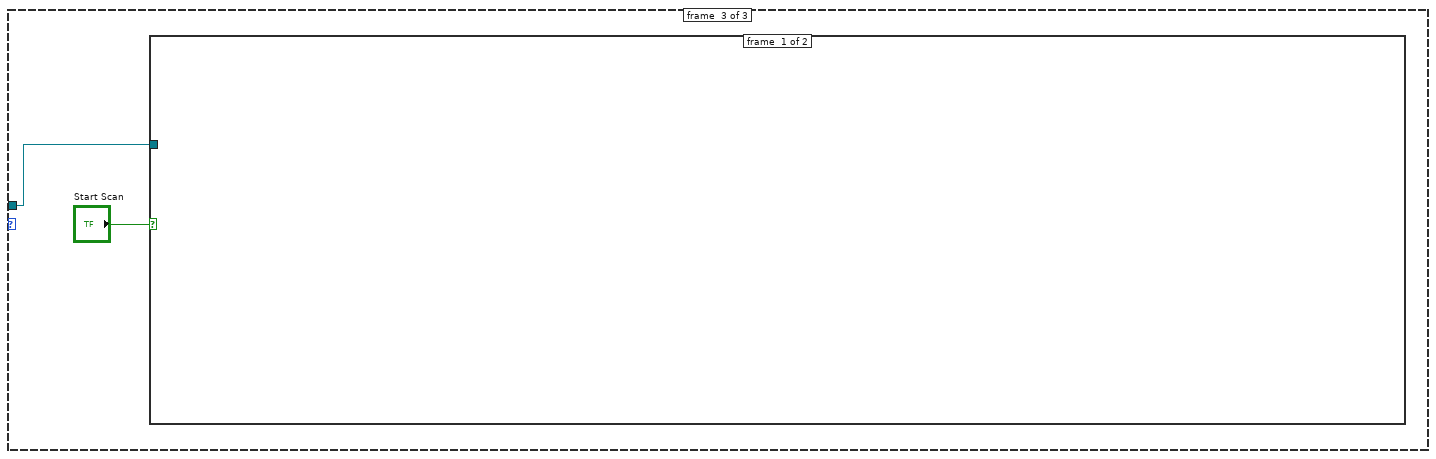
[diagram p3: hidden frame]
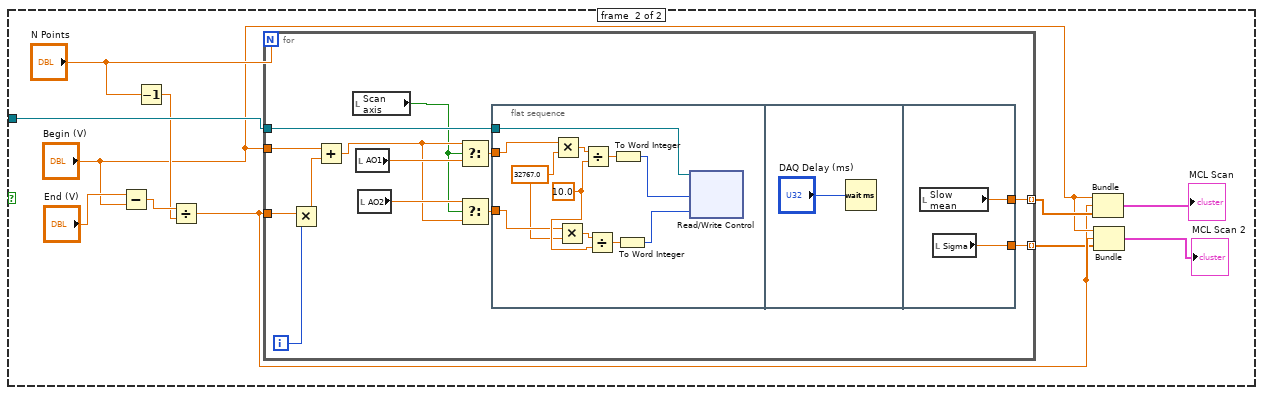
[diagram p4: hidden frame]
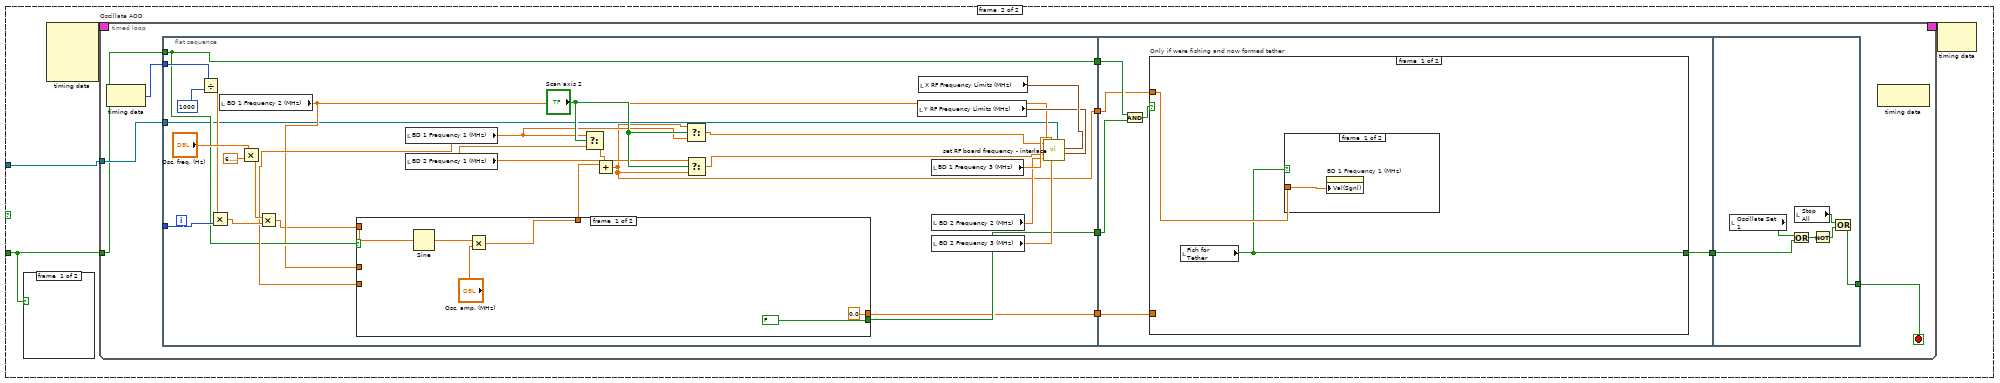
[diagram p6: hidden frame]
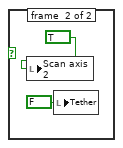
[diagram p7: hidden frame]
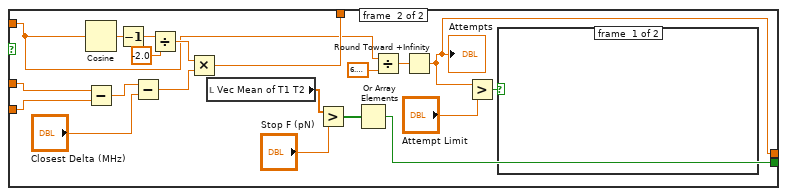
[diagram p8: hidden frame]
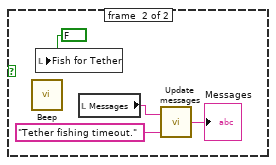
[diagram p9: hidden frame]
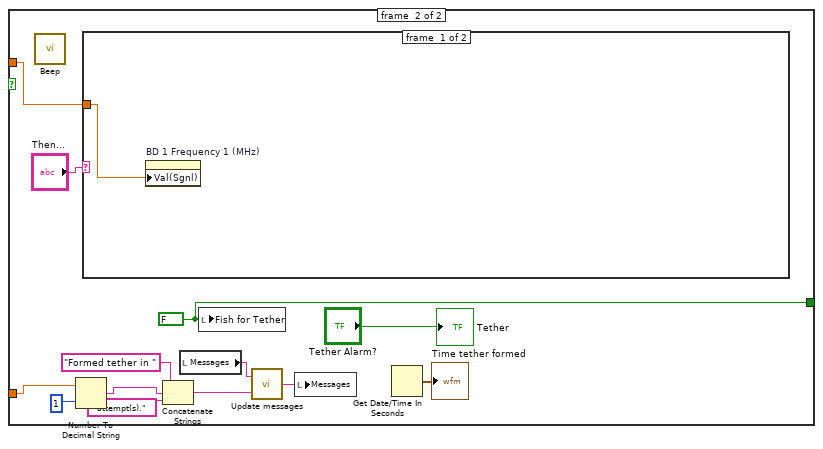
[diagram p11: hidden frame]
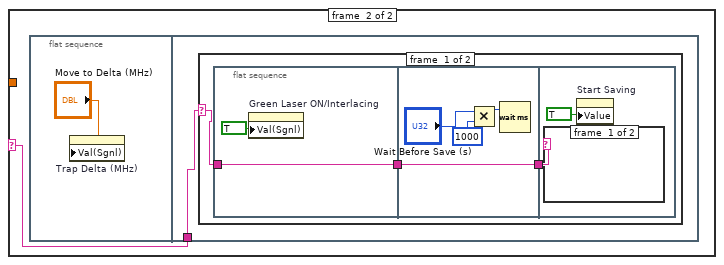
[diagram p12: hidden frame]
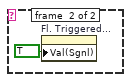
[diagram p13: hidden frame]
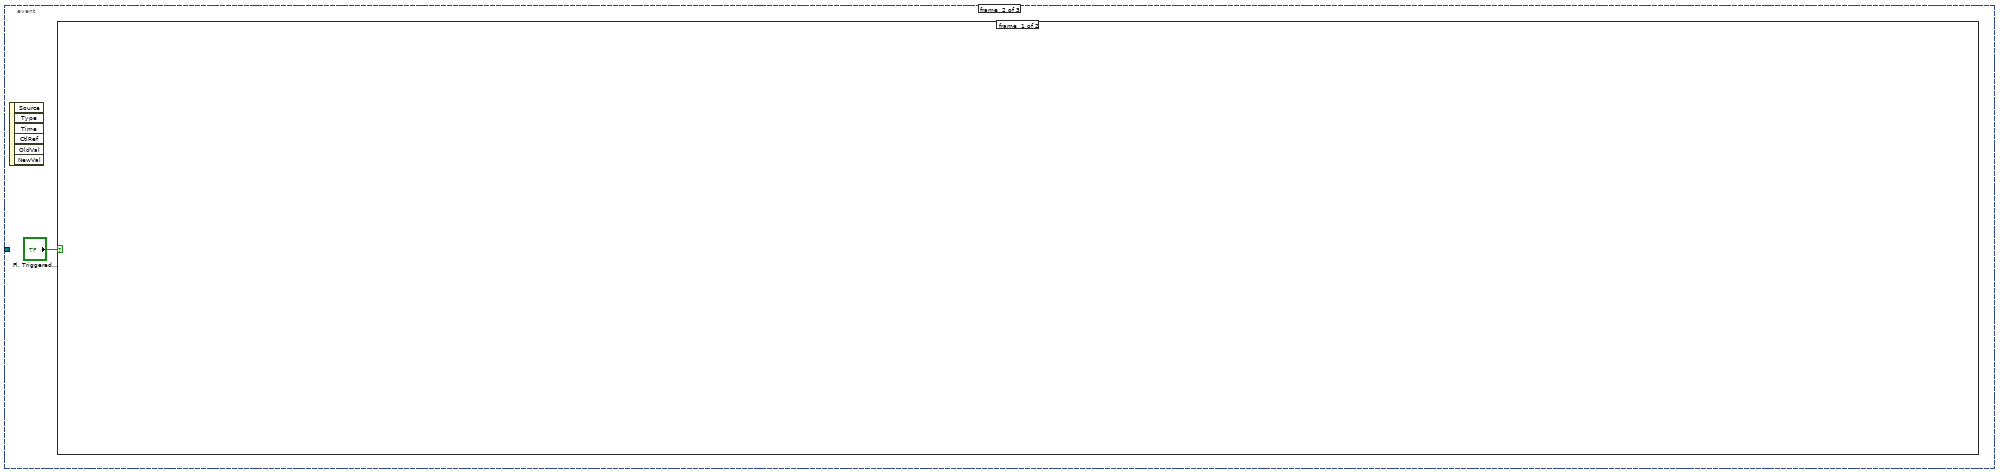
[diagram p15: hidden frame]
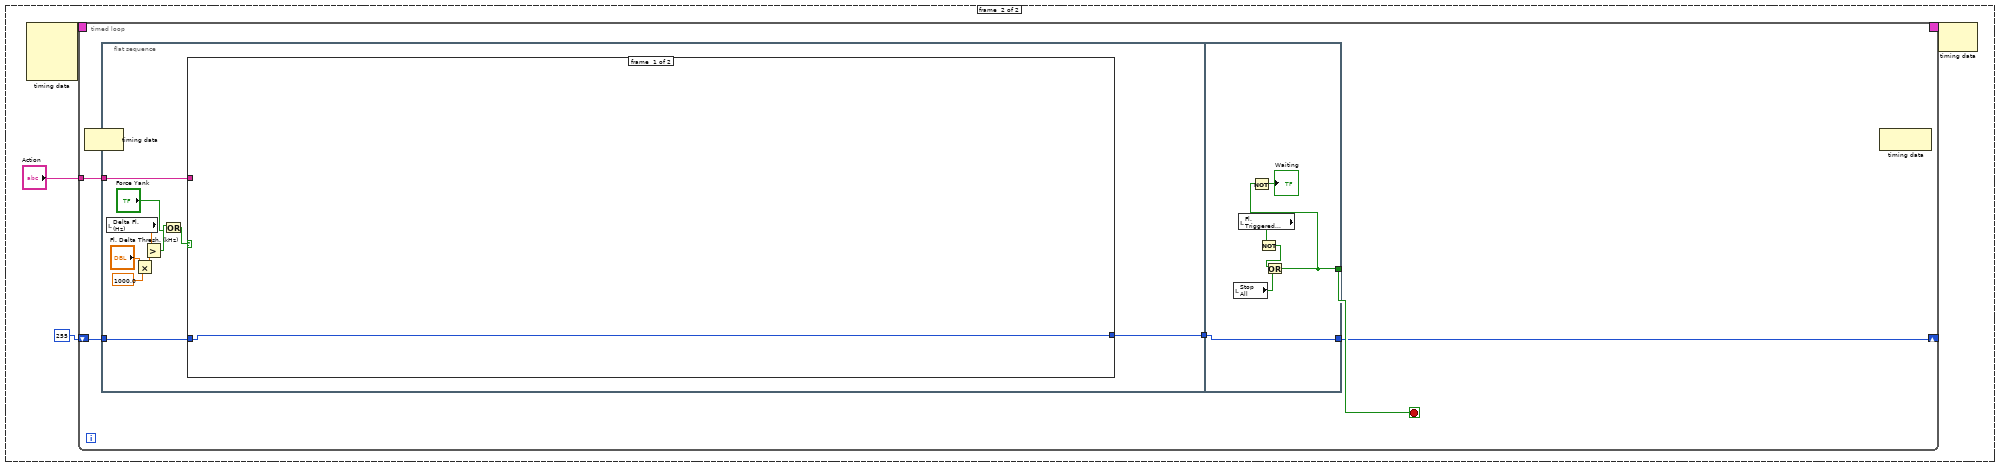
[diagram p16: hidden frame]
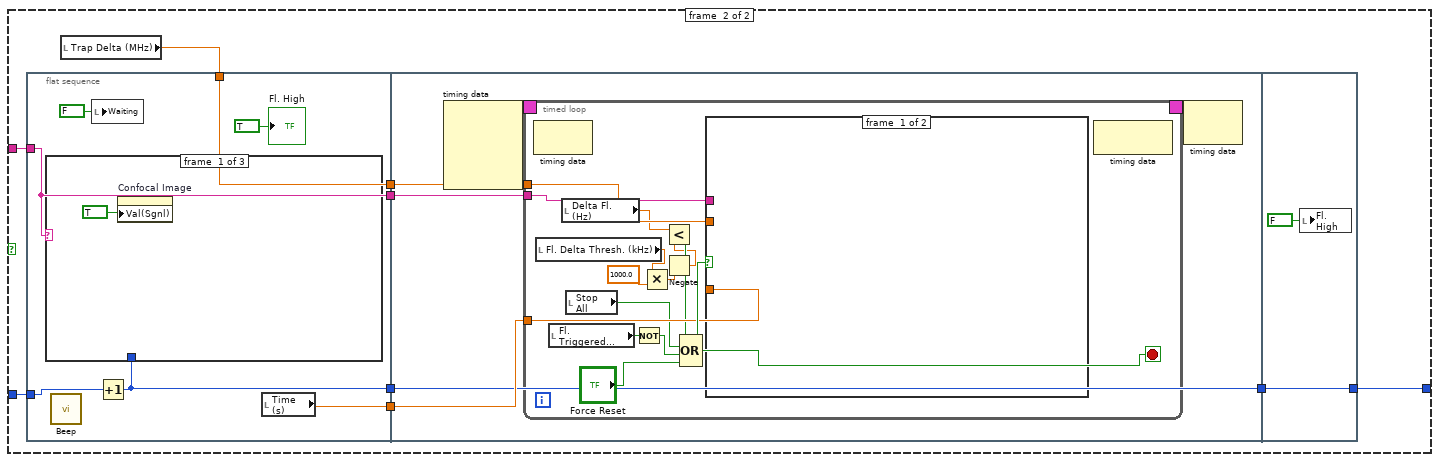
[diagram p17: hidden frame]
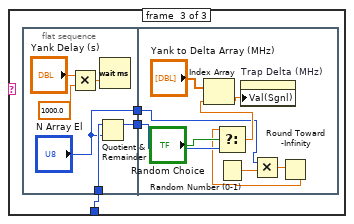
[diagram p19: hidden frame]
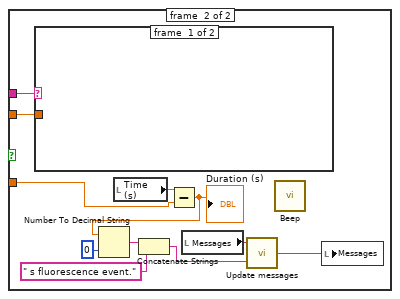
[diagram p20: hidden frame]
diagram:
  w3 = T13 2 items=["Grayscale (U8)", "Grayscale (I16)", "Grayscale (SGL)", "Complex (CSG)", "RGB (U32)", "HSL (U32)", "RGB (U64)", "Grayscale (U16)"] ("Image Type")
  w57 = T12 {"Minimum"=-0.1, "Maximum"=0.1, "Increment"=0.1}  # Z Limits
  w70 = cluster{"output high":i16, "output low":i16} {"output high"=3000, "output low"=0} ("FB output range 1")
  w76 = TRUE ("AI to FIFO")
  w161 = 10.0 ("y")
  w160 = 32767.0 ("y")
  w176 = 6.0  # clock mult.
  w177 = 49152000.0  # TCXO frequ.
  n1 = Build Array("DIO count 1 (ticks)", "DIO count 2 (ticks)", "DIO count 3 (ticks)") -> (w52:u32[])
  n2 = Multiply(x="APD Integration Time (s)", y=40000000.0) -> (x*y=w84:dbl)
  n3 = Reciprocal(x="APD Integration Time (s)") -> (1/x=w81:dbl)
  n4 = local write "APD Acq Rate (Hz)"(w81) -> ()
  n5 = local read "AO1"() -> (w155:dbl)
  n6 = local read "AO2"() -> (w154:dbl)
  n7 = To Unsigned Long Integer(number=w84) -> (unsigned 32bit integer=w83:u32)
  "APD Int. Count" <- w83
  n8 = local read "Scan Increment (MHz)"() -> (w172:dbl)
  n9 = local read "Continuous MCL Scanning"() -> (w142:bool)
  n10 = local read "Fast Scan Dir"() -> (w141:bool)
  n11 = Multiply(x=w155, y=w160) -> (x*y=w157:dbl)
  n12 = local read "Number of scans (MCL)"() -> (w143:u64)
  n13 = Multiply(x=w154, y=w160) -> (x*y=w159:dbl)
  n14 = Divide(x=w157, y=w161) -> (x/y=w156:dbl)
  n15 = Divide(x=w159, y=w161) -> (x/y=w158:dbl)
  n16 = To Word Integer(number=w156) -> (16bit integer=w153:i16)
  n17 = To Word Integer(number=w158) -> (16bit integer=w152:i16)
  n18 = Not(x=w141) -> (.not. x?=w136:bool)
  n19 = local read "Cycles/step (MCL)"() -> (w144:u64)
  n20 = Multiply(x=w172, y=1000.0) -> (x*y=w179:dbl)
  n21 = local read "Scan steps (MCL)"() -> (w145:u64)
  n22 = local read "Desired Scan Incr (V)"() -> (w147:dbl)
  n23 = Scale By Power Of 2(n=48, x=w179) -> (x*2^n=w180:dbl)
  n24 = Multiply(x=w177, y=w176) -> (x*y=w175:dbl)
  n25 = Divide(x=w180, y=w175) -> (x/y=w174:dbl)
  n26 = local read "Setpoints (V)"() -> (w200:cluster{"Set 1":dbl, "Set 2":dbl})
  n27 = property on="AI Count (ticks)" class="DigNum (strict)"("Val(Sgnl)"="AI Count (ticks)") -> ()  [unwired: 2 in, 2 out]
  n28 = local read "Number Interlace Sets"() -> (w45:u8)
  n29 = Split 1D Array(array=w52, index=w45) -> (first subarray=w54:u32[])  [unwired: 1 out]
  n30 = Add Array Elements(numeric array=w54) -> (sum=w53:u32)
  n31 = local read "# Samples/channel"() -> (w164:u32)
  n32 = To Quad Integer(1:w174) -> (0:w171:i64)
  n33 = local read "Sets to FIFO (Traps)"() -> (w207:T11)
  n34 = local read "Number of F/B Scans (AOD)"() -> (w165:u16)
  n35 = local read "Not-Interlacing Set"() -> (w44:enum32{"Set 1", "Set 2", "Set 3"})
  n36 = To Unsigned Byte Integer(number=w44) -> (unsigned 8bit integer=w50:u8)
  n37 = Index Array(array=w52, index=w50) -> (element=w51:u32)
  n38 = Divide(x=40000000.0, y="AI Count (ticks)") -> (x/y=w132:dbl)
  n39 = Multiply(x=w147, y=32767.0) -> (x*y=w149:dbl)
  n40 = local read "Feedback On/Off"() -> (w203:cluster{"Set 1":bool, "Set 2":bool})
  n41 = local read "PID Gains"() -> (w195:T9)
  n42 = local read "Scan steps (AOD)"() -> (w170:u64)
  n43 = local read "All FB On/Off"() -> (w204:bool)
  n44 = local read "Cycles/step (AOD)"() -> (w169:u64)
  n45 = local write "AI rate (Hz)"(w132) -> ()
  n46 = Divide(x=w149, y=10.0) -> (x/y=w148:dbl)
  n47 = Multiply(x=w170, y=w169) -> (x*y=w168:u64)
  n48 = Multiply(x=3276.7, y=w200) -> (x*y=w199:cluster{"Set 1":dbl, "Set 2":dbl})
  n49 = To Word Integer(number=w148) -> (16bit integer=w146:i16)
  n50 = Multiply(x=w168, y=u64 2) -> (x*y=w166:u64)
  n51 = Divide(x=w132, y="FPGA Ave.") -> (x/y=w133:dbl)
  n52 = To Word Integer(number=w199) -> (16bit integer=w198:cluster{"Set 1":i16, "Set 2":i16})
  n53 = xnode "Open FPGA VI Reference"("resource name"=T14 "750kHzDAQ") -> ("FPGA VI Reference Out"=w187:T15, "error out"=w186:errorcluster)  [unwired: 1 in]
  n54 = Unbundle By Name(w195) -> ("Set 1"=w194:T10, "Set 2"=w193:T10)
  n55 = Multiply(x=w166, y=w165) -> (x*y=w163:u64)
  n56 = Divide(x=w163, y=w164) -> (x/y=w162:dbl)
  n57 = local write "Ave. Rate (Hz)"(w133) -> ()
  n58 = Unbundle By Name(w198) -> ("Set 1"=w197:i16, "Set 2"=w196:i16)
  n59 = local read "2D or 1D Scan"() -> (w73:bool)
  n60 = local write "Data points/scans"(w163) -> ()
  n61 = And(x=w203, y=w204) -> (x .and. y?=w202:cluster{"Set 1":bool, "Set 2":bool})
  n62 = local read "Scan BD"() -> (w181:bool)
  n63 = Reciprocal(x=w133) -> (1/x=w134:dbl)
  n64 = local write "Data points/scan (f/b)"(w166) -> ()
  n65 = local read "N Acq Sets (Traps + Fl.)"() -> (w125:i16)
  n66 = local write "N sets should be saved"(w162) -> ()
  n67 = Unbundle By Name(w202) -> ("Set 1"=w206:bool, "Set 2"=w205:bool)
  n68 = xnode "Invoke Method"("FPGA VI Reference In"=w187, "error in"=w186) -> ("FPGA VI Reference Out"=w69:T15, "error out"=w99:errorcluster)
  n69 = local read "Interlace"() -> (w46:bool)
  n70 = Select(t=w53, s=w46, f=w51) -> (s? t:f=w43:u32)
  n71 = local write "Update Count (MCL)"(w43) -> ()
  n72 = local write "Total Counts (ticks)"(w43) -> ()
  n73 = local write "Ave. Period (s)"(w134) -> ()
  n74 = property on="2D or 1D Scan" class="Bool (strict)"("Val(Sgnl)"=w73) -> ()  [unwired: 2 in, 2 out]
  n75 = xnode "Read/Write Control"("FPGA VI Reference In"=w68, "error in"=w99, "ai count"="AI Count (ticks)", "AI Averages"="FPGA Ave.", "DMA buffer timeout"=0, "AI to FIFO"=FALSE, "Interlace ON/OFF"=w46, "Number Interlace Cycles"=w45, "AI1 Sets to FIFO"=w207, "FB On/Off Set 1"=w206, "FB On/Off Set 2"=w205, "Interlace Off Parameters"=w44, "FB Setpoint Set 1"=w197, "FB Setpoint Set 2"=w196, "FB Gains Set 1"=w194, "FB Gains Set 2"=w193, "FB output range 1"=w70, "FB output range 2"=w70, "Cycles per step"=w169, "Scan BD"=w181, "Number of scans"=w165, "Scan steps"=w170, "Scan freq.  increment"=w171, "AO1"=w153, "AO2"=w152, "Scan freq.  increment (MCL)"=w146, "Scan steps (MCL)"=w145, "Cycles per step (MCL)"=w144, "Number of scans (MCL)"=w143, "MCL count"=w43, "Cont. Scan (MCL)"=w142, "MCL Scan Axis"=w136, "1D or 2D Scan?"=w73, "N of AI1 Int Acq Sets"=w125, "Freq or Amp switch first"="Freq or Amp switch first", "Freq switch delay"="Freq switch delay", "Amp switch delay"="Amp switch delay", "Swap F1 and F2"="Swap F1 and F2", "APD Acq Rate Count"=w83, "APD to FIFO"=FALSE, "APD Gate Operating Mode"="APD Gate", "APD Gate ON Count"="APD Gate ON Count", "APD Gate OFF Count"="APD Gate OFF Count", "Invert APD Gate"="Invert APD Gate", "DIO count 1 (ticks)"="DIO count 1 (ticks)", "DIO count 2 (ticks)"="DIO count 2 (ticks)", "DIO count 3 (ticks)"="DIO count 3 (ticks)", "APD 1 AO scale factor"="APD 1 AO Mult.", "APD 2 AO scale factor"="APD 2 AO Mult.", "APD 1 AO offset"="APD 1 AO offset", "APD 2 AO offset"="APD 2 AO offset") -> ("FPGA VI Reference Out"=w38:T15, "error out"=w40:errorcluster)
  n76 = local read "Green Laser ON/Interlacing"() -> (w41:bool)
  n77 = local read "GI Frequency, OFF count"() -> (w34:u32)
  n78 = local read "GI Frequency, ON count"() -> (w33:u32)
  n79 = Multiply(x="Current When FB OFF (%)", y=655.35) -> (x*y=w24:dbl)
  n80 = local read "Green laser mode"() -> (w42:enum32{"Laser ON", "Laser OFF", "Interlace"})
  n81 = local read "Green FB Count"() -> (w32:u32)
  n82 = To Unsigned Word Integer(number=w24) -> (unsigned 16bit integer=w22:u16)
  n83 = local read "Invert GI"() -> (w36:bool)
  n84 = Multiply(x="Green FB Setpoint (mV)", y=3.2767) -> (x*y=w21:dbl)
  n85 = case shown="False" w41 {
    tunnel: w42 -> [_ w234]
    tunnel: [enum32{"Laser ON", "Laser OFF", "Interlace"}."Laser OFF" ("Green laser mode") w234] -> w35
    frame #0 {
    }
    frame #1 {
    }
  }
  n86 = To Word Integer(number=w21) -> (16bit integer=w19:i16)
  n87 = xnode "Read/Write Control"("FPGA VI Reference In"=w38, "error in"=w40, "Green interlace ON count 2"=w33, "Green interlace OFF count 2"=w34, "Invert GI 2"=w36, "Operating Mode 2"=w35, "Green FB Gains"="Green FB Gains", "Green FB Setpoint"=w19, "Green FB On/Off"="Green FB On/Off", "Current Out"=w22, "Green int current ON count adj"="Green int current ON count adj", "Green FB Count"=w32, "Operating Mode"=w35, "Green interlace OFF count"=w34, "Green interlace ON count"=w33, "Invert GI"=w36) -> ("FPGA VI Reference Out"=w37:T15, "error out"=w39:errorcluster)
  n88 = flat-sequence {
    tunnel: w69 -> [w239]
    tunnel: [w239] -> w68
    tunnel: [w238] -> w67
    tunnel: [w237] -> w66
    tunnel: [w235] -> w64
    tunnel: [w236] -> w65
    frame #0 {
      w236 = T12 {"Minimum"=0.0, "Maximum"=40.0, "Increment"=1.0} ("Min Max Inc")
      w235 = T12 {"Minimum"=0.0, "Maximum"=50.0, "Increment"=1.0} ("Data Entry Limits")
      w238 = T12 {"Minimum"=60.0, "Maximum"=90.0, "Increment"=1.0} ("Min Max Inc")
      w237 = T12 {"Minimum"=0.0, "Maximum"=50.0, "Increment"=1.0} ("Data Entry Limits")
      n89 = property on="BD 2 Frequency 1 (MHz)" class="DigNum (strict)"("Data Range"=w236) -> ()  [unwired: 2 in, 2 out]
      n90 = property on="BD 2 Frequency 3 (MHz)" class="DigNum (strict)"("Data Range"=w236) -> ()  [unwired: 2 in, 2 out]
      n91 = property on="BD 2 Frequency 2 (MHz)" class="DigNum (strict)"("Data Range"=w236) -> ()  [unwired: 2 in, 2 out]
      n92 = property on="BD 1 Frequency 1 (MHz)" class="DigNum (strict)"("Data Range"=w238) -> ()  [unwired: 2 in, 2 out]
      n93 = property on="BD 1 Frequency 2 (MHz)" class="DigNum (strict)"("Data Range"=w238) -> ()  [unwired: 2 in, 2 out]
      n94 = property on="BD 1 Frequency 3 (MHz)" class="DigNum (strict)"("Data Range"=w238) -> ()  [unwired: 2 in, 2 out]
      n95 = property on="BD 2 Amplitude 1 (%)" class="DigNum (strict)"("Data Range"=w235) -> ()  [unwired: 2 in, 2 out]
      n96 = property on="BD 2 Amplitude 2 (%)" class="DigNum (strict)"("Data Range"=w235) -> ()  [unwired: 2 in, 2 out]
      n97 = property on="BD 2 Amplitude 3 (%)" class="DigNum (strict)"("Data Range"=w235) -> ()  [unwired: 2 in, 2 out]
      n98 = property on="BD 1 Amplitude 3 (%)" class="DigNum (strict)"("Data Range"=w237) -> ()  [unwired: 2 in, 2 out]
      n99 = property on="BD 1 Amplitude 2 (%)" class="DigNum (strict)"("Data Range"=w237) -> ()  [unwired: 2 in, 2 out]
      n100 = property on="BD 1 Amplitude 1 (%)" class="DigNum (strict)"("Data Range"=w237) -> ()  [unwired: 2 in, 2 out]
      "X RF Frequency Limits (MHz)" <- w238
      "X RF Amplitude Limits (%)" <- w237
      "Y RF Amplitude Limits (%)" <- w235
      "Y RF Frequency Limits (MHz)" <- w236
    }
  }
  n101 = xnode "Invoke Method"("FPGA VI Reference In"=w37, "error in"=w39, "Depth"="FIFO Depth") -> ("FPGA VI Reference Out"=w192:T15, "error out"=w191:errorcluster)
  n102 = xnode "Invoke Method"("FPGA VI Reference In"=w192, "error in"=w191) -> ("FPGA VI Reference Out"=w98:T15, "error out"=w97:errorcluster)
  n103 = xnode "Invoke Method"("FPGA VI Reference In"=w98, "error in"=w97) -> ("FPGA VI Reference Out"=w96:T15, "error out"=w95:errorcluster)  [unwired: 1 out]
  n104 = flat-sequence "Initial FPGA Loop Relative Phase Adjustment" {
    tunnel: "Initial Phase Adjustment (AI1)" -> [w249]
    tunnel: "Initial Phase Adjustment (GI)" -> [w248]
    tunnel: w96 -> [w247]
    tunnel: w95 -> [w246]
    tunnel: "Initial Phase Adj. (MCL)" -> [w245]
    tunnel: [w250] -> w107
    tunnel: [w244] -> w103
    tunnel: "Initial Phase Adjustment (APD Acq)" -> [w243]
    tunnel: "Initial Phase Adjustment (APD Gate)" -> [w242]
    tunnel: "Initial Phase Adjustment (Green FB)" -> [w241]
    tunnel: "Initial Phase Adjustment (GI) 2" -> [w240]
    tunnel: w107 -> [w402]
    tunnel: [w403] -> w104
    tunnel: w103 -> [w403]
    tunnel: [w402] -> w102
    tunnel: w104 -> [w406]
    tunnel: w102 -> [w405]
    tunnel: [w408] -> w101
    tunnel: [w407] -> w100
    tunnel: [w567] -> w105
    tunnel: [w568] -> w106
    tunnel: w101 -> [w568]
    tunnel: w100 -> [w567]
    frame #0 {
      n105 = xnode "Read/Write Control"("FPGA VI Reference In"=w247, "error in"=w246, "Phase count adjustment"=w249, "Phase count adjustment (GI)"=w248, "Phase count adjustment (MCL)"=w245, "Phase Count Adjustment (APD Acq)"=w243, "Phase count adjustment (APD Gate)"=w242, "Phase count adjustment (Green FB)"=w241, "Phase count adjustment (GI) 2"=w240) -> ("FPGA VI Reference Out"=w244:T15, "error out"=w250:errorcluster)
    }
    frame #1 {
      n106 = Wait (ms)(milliseconds to wait=u32 1000) -> ()  [unwired: 1 out]
    }
    frame #2 {
      w404 = TRUE
      n107 = xnode "Read/Write Control"("FPGA VI Reference In"=w406, "error in"=w405, "+ phase"=w404, "+ phase (GI)"=w404, "+ phase (MCL)"=w404, "+ phase (APD Acq)"=w404, "+ phase (APD Gate)"=w404, "+ phase (Green FB)"=w404, "+ phase (GI) 2"=w404) -> ("FPGA VI Reference Out"=w407:T15, "error out"=w408:errorcluster)
    }
    frame #3 {
      n108 = Wait (ms)(milliseconds to wait=u32 1000) -> ()  [unwired: 1 out]
    }
  }
  n109 = local read "Phase adj. (Green FB)"() -> (w55:i16)
  n110 = local read "Phase adj. (GI) 2"() -> (w25:i16)
  n111 = local read "Phase adjust (MCL)"() -> (w137:i16)
  n112 = local read "Phase adj. (AI1)"() -> (w139:i16)
  n113 = local read "Phase adj. (GI)"() -> (w138:i16)
  n114 = xnode "Read/Write Control"("FPGA VI Reference In"=w105, "error in"=w106, "Phase count adjustment"=w139, "Phase count adjustment (GI)"=w138, "Phase count adjustment (MCL)"=w137, "Phase Count Adjustment (APD Acq)"="Phase Adj. (APD Acq)", "Phase count adjustment (APD Gate)"="Phase Adj. (APD Gate)", "Phase count adjustment (Green FB)"=w55, "Phase count adjustment (GI) 2"=w25) -> ("FPGA VI Reference Out"=w8:T15, "error out"=w114:errorcluster)
  n115 = call "Initialize RF boards - interlace 3.vi"("error in"=w114, "FPGA VI Reference In"=w8) -> ("error out"=w112:errorcluster, "FPGA VI Reference Out"=w113:T15)
  n116 = call "set RF board frequency - interlace.vi"("Board 2 Frequency Limits"=w65, "Board 1 Frequency Limits"=w67, "error in"=w112, "FPGA VI Reference In"=w113, "Board 2 Frequency 3 (MHz)"="BD 2 Frequency 3 (MHz)", "Board 1 Frequency 3 (MHz)"="BD 1 Frequency 3 (MHz)", "Board 2 Frequency 2 (MHz)"="BD 2 Frequency 2 (MHz)", "Board 2 Frequency 1 (MHz)"="BD 2 Frequency 1 (MHz)", "Board 1 Frequency 2 (MHz)"="BD 1 Frequency 2 (MHz)", "Board 1 Frequency 1  (MHz)"="BD 1 Frequency 1 (MHz)") -> ("error out"=w223:errorcluster, "FPGA VI Reference Out"=w224:T15)
  n117 = call "set RF board amplitude - interlace.vi"("Board 2 Amplitude Limits"=w64, "Board 1 Amplitude Limits"=w66, "error in"=w223, "FPGA VI Reference In"=w224, "Board 2 Amplitude 3 (%)"="BD 2 Amplitude 3 (%)", "Board 1 Amplitude 3 (%)"="BD 1 Amplitude 3 (%)", "Board 2 Amplitude 2 (%)"="BD 2 Amplitude 2 (%)", "Board 2 Amplitude 1 (%)"="BD 2 Amplitude 1 (%)", "Board 1 Amplitude 2 (%)"="BD 1 Amplitude 2 (%)", "Board 1 Amplitude 1 (%)"="BD 1 Amplitude 1 (%)") -> ("error out"=w211:errorcluster, "FPGA VI Reference Out"=w212:T15)
  n118 = flat-sequence {
    tunnel: w212 -> [w577]
    tunnel: w211 -> [w576]
    tunnel: [w575] -> w216
    tunnel: [w574] -> w215
    tunnel: [w618] -> w214
    tunnel: w216 -> [w618]
    tunnel: [w617] -> w213
    tunnel: w215 -> [w617]
    tunnel: w214 -> [w626]
    tunnel: w213 -> [w625]
    tunnel: [w624] -> w78
    tunnel: [w623] -> w77
    frame #0 {
      n119 = local read "Trap 1 (ON/OFF)"() -> (w569:bool)
      n120 = xnode "Read/Write Control"("FPGA VI Reference In"=w577, "error in"=w576, "Direct RF Box  Communication"=FALSE) -> ("FPGA VI Reference Out"=w575:T15, "error out"=w574:errorcluster)
      n121 = local write "Saving..."(FALSE ("Saving Data")) -> ()
      n122 = local write "Stop All"(FALSE ("Stop All")) -> ()
      n123 = local write "Index"(1.0 ("Index")) -> ()
      n124 = property on="Trap 1 ON" class="Bool (strict)"("Value"=w569) -> ()  [unwired: 2 in, 2 out]
      "Manipulating Trap" <- FALSE ("Manipulating Trap")
    }
    frame #1 {
      n125 = local read "Trap 2 (ON/OFF)"() -> (w616:bool)
      n126 = Wait (ms)(milliseconds to wait=u32 10) -> ()  [unwired: 1 out]
      n127 = property on="Trap 2 ON" class="Bool (strict)"("Val(Sgnl)"=w616) -> ()  [unwired: 2 in, 2 out]
    }
    frame #2 {
      n128 = xnode "Read/Write Control"("FPGA VI Reference In"=w626, "error in"=w625, "FPGA Controls  RF Box"=TRUE ("Direct RF Box  Communication")) -> ("FPGA VI Reference Out"=w624:T15, "error out"=w623:errorcluster)
      n129 = call "Update messages.vi"("Message to add"="UHR-Fleezers ready.", "Old message string"="") -> ("New message string"=w622:string)
      n130 = local write "Messages"(w622) -> ()
    }
  }
  n131 = Subtract(x="BD 1 Frequency 1 (MHz)", y="BD 1 Frequency 2 (MHz)") -> (x-y=w124:dbl)
  n132 = Subtract(x="BD 2 Frequency 1 (MHz)", y="BD 2 Frequency 2 (MHz)") -> (x-y=w123:dbl)
  n133 = Square(x=w123) -> (x^2=w121:dbl)
  n134 = Square(x=w124) -> (x^2=w122:dbl)
  n135 = Add(x=w122, y=w121) -> (x+y=w120:dbl)
  n136 = Square Root(x=w120) -> (sqrt(x)=w119:dbl)
  n137 = local write "Trap Delta (MHz)"(w119) -> ()
  n138 = xnode "Read/Write Control"("FPGA VI Reference In"=w78, "error in"=w77, "AI to FIFO"=w76, "APD to FIFO"=w76) -> ("FPGA VI Reference Out"=w75:T15, "error out"=w74:errorcluster)
  n139 = property on="pos 1 z" class="DigNum (strict)"("Data Range"=w57) -> ()  [unwired: 2 in, 2 out]
  n140 = property on="pos 2 z" class="DigNum (strict)"("Data Range"=w57) -> ()  [unwired: 2 in, 2 out]
  n141 = property on="pos 3 z" class="DigNum (strict)"("Data Range"=w57) -> ()  [unwired: 2 in, 2 out]
  n142 = property class="DigNum (strict)"("Data Range"=w57) -> ()  [unwired: 2 in, 2 out]
  n143 = call "IMAQ Create"("Image Name"="Det. Y Image", "Image Type"=w3) -> ("New Image"=w1:T2)  [unwired: 3 in, 1 out]
  n144 = call-poly "VISA Configure Serial Port"("VISA resource name"="Sample Chamber Stage Serial Port") -> ("VISA resource name out"=w61:refnum<visa-resource-name>, "error out"=w60:errorcluster)  [unwired: 5 in, 8 out]
  n145 = call "IMAQ Create"("Image Name"="Det. X Image", "Image Type"=w3) -> ("New Image"=w2:T2)  [unwired: 3 in, 1 out]
  n146 = call "IMAQ Create"("Image Name"="APD1 Image", "Image Type"=w3) -> ("New Image"=w6:T2)  [unwired: 3 in, 1 out]
  n147 = disable-structure shown="Disabled" {
    disable-tunnel: [w666 _] -> w184
    disable-tunnel: w78 -> [w665 _]
    frame #0 {
      n148 = node-c288() -> (w668:T18)  [unwired: 4 out]
      n149 = timed-loop "Rough control of MCL mirror stage (debugging)" {
        tunnel: w665 -> [w671]
        tunnel: [w670] -> w666
        timing: w668 -> [_]
        timing-out: [_] -> w667
        stop <- w670 stop-if-true
        n150 = node-c288() -> ()  [unwired: 2 out]
        n151 = case shown="1" "MCL Mode" {
          tunnel: w671 -> [_ w674 w776]
          frame #0 {
          }
          frame #1 {
            n152 = node-c288() -> (w676:T18)  [unwired: 4 out]
            n153 = timed-loop "Oscillate MCL mirror" {
              timing: w676 -> [_]
              timing-out: [_] -> w675
              tunnel: w674 -> [w715]
              i -> [w714]
              stop <- w677 stop-if-true
              n154 = node-c288() -> (w713:i64)  [unwired: 1 out]
              n155 = Multiply(x="AO1", y=32767.0) -> (x*y=w709:dbl)
              n156 = Multiply(x="AO2", y=32767.0) -> (x*y=w704:dbl)
              n157 = Divide(x=w709, y=10.0) -> (x/y=w710:dbl)
              n158 = Divide(x=w704, y=10.0) -> (x/y=w705:dbl)
              n159 = To Word Integer(number=w710) -> (16bit integer=w702:i16)
              n160 = To Word Integer(number=w705) -> (16bit integer=w701:i16)
              n161 = Divide(x=w713, y=i64 1000) -> (x/y=w684:dbl)
              n162 = Multiply(x=w684, y=w714) -> (x*y=w695:dbl)
              n163 = Multiply(x="Osc. freq. (Hz) 2", y=6.283185307179586) -> (x*y=w696:dbl)
              n164 = Multiply(x=w696, y=w695) -> (x*y=w694:dbl)
              n165 = Sine(x=w694) -> (sin(x)=w693:dbl)
              n166 = Multiply(x=w693, y="Osc. amp. (V)") -> (x*y=w691:dbl)
              n167 = Add(x=w691, y="Osc. center (V)") -> (x+y=w689:dbl)
              n168 = Divide(x=w689, y=10.0) -> (x/y=w687:dbl)
              n169 = Multiply(x=w687, y=32767.0) -> (x*y=w682:dbl)
              n170 = Select(t=w682, s="Scan axis", f=w702) -> (s? t:f=w700:dbl)
              n171 = Select(t=w701, s="Scan axis", f=w682) -> (s? t:f=w699:dbl)
              n172 = local read "MCL Mode"() -> (w681:u16)
              n173 = Not Equal?(x=w681, y=u16 1) -> (x != y?=w678:bool)
              n174 = local read "Stop All"() -> (w679:bool)
              n175 = xnode "Read/Write Control"("FPGA VI Reference In"=w715, "AO1"=w700, "AO2"=w699) -> ()  [unwired: 1 in, 2 out]
              n176 = Compound Arithmetic op=OR(w679, w678) -> (w677:bool)
              n177 = node-c288() -> ()  [unwired: 2 out]
            }
            n178 = node-c288(w675) -> ()  [unwired: 1 out]
          }
          frame #2 {
            n179 = case shown="True" "Start Scan" {
              tunnel: w776 -> [_ w788]
              frame #0 {
              }
              frame #1 {
                n180 = Subtract(x="End (V)", y="Begin (V)") -> (x-y=w784:dbl)
                n181 = Decrement(x="N Points") -> (x-1=w783:dbl)
                n182 = Divide(x=w784, y=w783) -> (x/y=w781:dbl)
                n183 = for {
                  N: "N Points" -> [_]
                  tunnel: "Begin (V)" -> [w801]
                  tunnel: w788 -> [w793]
                  tunnel: [w792] -> w787 mode=indexing
                  tunnel: w781 -> [w791]
                  tunnel: [w789] -> w780 mode=indexing
                  i -> [w800]
                  n184 = Multiply(x=w791, y=w800) -> (x*y=w799:dbl)
                  n185 = Add(x=w801, y=w799) -> (x+y=w796:dbl)
                  n186 = local read "Scan axis"() -> (w790:bool)
                  n187 = local read "AO1"() -> (w798:dbl)
                  n188 = local read "AO2"() -> (w797:dbl)
                  n189 = Select(t=w796, s=w790, f=w798) -> (s? t:f=w795:dbl)
                  n190 = Select(t=w797, s=w790, f=w796) -> (s? t:f=w794:dbl)
                  n191 = flat-sequence {
                    tunnel: w795 -> [w805]
                    tunnel: w794 -> [w804]
                    tunnel: w793 -> [w802]
                    tunnel: [w870] -> w792
                    tunnel: [w869] -> w789
                    frame #0 {
                      w808 = 10.0 ("y")
                      w803 = 32767.0 ("y")
                      n192 = Multiply(x=w805, y=w803) -> (x*y=w811:dbl)
                      n193 = Multiply(x=w804, y=w803) -> (x*y=w809:dbl)
                      n194 = Divide(x=w811, y=w808) -> (x/y=w812:dbl)
                      n195 = Divide(x=w809, y=w808) -> (x/y=w810:dbl)
                      n196 = To Word Integer(number=w812) -> (16bit integer=w806:i16)
                      n197 = To Word Integer(number=w810) -> (16bit integer=w807:i16)
                      n198 = xnode "Read/Write Control"("FPGA VI Reference In"=w802, "AO1"=w806, "AO2"=w807) -> ()  [unwired: 1 in, 2 out]
                    }
                    frame #1 {
                      n199 = Wait (ms)(milliseconds to wait="DAQ Delay (ms)") -> ()  [unwired: 1 out]
                    }
                    frame #2 {
                      n200 = local read "Slow mean"() -> (w870:dbl)
                      n201 = local read "Sigma"() -> (w869:dbl)
                    }
                  }
                }
                n202 = Bundle("Begin (V)"="Begin (V)", w781, w787) -> (→"MCL Scan":cluster{"Begin (V)":dbl, dbl, dbl[]})  [unwired: 1 out]
                n203 = Bundle("Begin (V)"="Begin (V)", w781, w780) -> (→"MCL Scan 2":cluster{"Begin (V)":dbl, dbl, dbl[]})  [unwired: 1 out]
              }
            }
          }
        }
        n204 = local read "Stop All"() -> (w670:bool)
        n205 = node-c288() -> ()  [unwired: 2 out]
      }
      n206 = node-c288(w667) -> ()  [unwired: 1 out]
    }
    frame #1 {
    }
  }
  n207 = node-c288() -> (w13:T18)  [unwired: 4 out]
  n208 = node-c288() -> (w17:T18)  [unwired: 4 out]
  n209 = node-c288() -> (w11:T18)  [unwired: 4 out]
  n210 = node-c288() -> (w15:T18)  [unwired: 4 out]
  n211 = timed-loop "Control parameters (event loop)" {
    tunnel: w78 -> [w876]
    shift-right: [w875] -> _
    shift-left: errorcluster {"status"=FALSE, "code"=0, "source"=""} ("error out") -> [w874]
    tunnel: [w873] -> w182
    timing: w13 -> [_]
    timing-out: [_] -> w12
    stop <- w873 stop-if-true
    n212 = node-c288() -> ()  [unwired: 2 out]
    n213 = event shown="[44] \"Inject Pump 3 (D)\": Value Change" {
      selector: _ -> [_ _ _ _ _ _ _ _ _ _ _ _ _ _ _ _ _ _ _ _ _ _ _ _ _ _ _ _ _ _ _ _ _ _ _ _ _ _ _ _ _ _ _ _ _ _ _]
      dyn-events: _ -> [_ _ _ _ _ _ _ _ _ _ _ _ _ _ _ _ _ _ _ _ _ _ _ _ _ _ _ _ _ _ _ _ _ _ _ _ _ _ _ _ _ _ _ _ _ _ _]
      timeout: _ -> [_ _ _ _ _ _ _ _ _ _ _ _ _ _ _ _ _ _ _ _ _ _ _ _ _ _ _ _ _ _ _ _ _ _ _ _ _ _ _ _ _ _ _ _ _ _ _]
      tunnel: w876 -> [w917 _ _ w1044 _ w1139 _ _ _ _ w1205 _ _ _ _ _ _ _ w1325 w1463 w1525 w1568 w1718 w1793 w1904 w1997 w2081 w2165 w2249 w2333 w2426 w2621 w2821 w2914 w3047 _ w3217 w3258 w3305 w3382 w3423 _ w3468 _ _ _ w3616]
      tunnel: [w916 _ _ w1034 _ w1138 _ _ w1170 _ w1184 _ _ _ _ _ _ _ w1324 w1459 w1522 w1565 w1717 w1791 w1903 w1991 w2075 w2159 w2243 w2327 w2424 w2620 w2819 w2912 w3045 _ w3215 w3256 w3295 w3380 w3421 _ w3466 _ _ _ w3614] -> w875
      tunnel: w874 -> [w915 _ _ w1043 _ w1137 _ _ w1170 _ w1204 _ _ _ _ _ _ _ w1323 w1458 w1521 w1564 w1716 w1792 w1902 w1996 w2080 w2164 w2248 w2332 w2425 w2619 w2820 w2913 w3046 _ w3216 w3257 w3304 w3381 w3422 _ w3467 _ _ _ w3615]
      tunnel: [_ _ _ _ _ _ _ _ w1169 _ _ _ _ _ _ _ _ _ _ _ _ _ _ _ _ _ _ _ _ _ _ _ _ _ _ _ _ _ _ _ _ _ _ _ _ _ _] -> w873
      tunnel: [_ _ _ _ _ _ "Round T1 X" _ _ _ _ _ _ _ _ _ "Load parameters" _ _ _ _ _ _ _ _ _ _ _ _ _ _ _ _ _ _ _ _ _ _ _ _ _ _ _ _ _ _] -> _
      tunnel: [_ _ "Adjust Scale\nto Mean" _ _ _ _ _ _ _ _ "Set Position 1" "Set Position 2" "Set Position 3" "Set Position 4" "Set Position 5" _ _ _ _ _ _ _ _ _ _ _ _ _ _ _ _ _ _ _ _ _ _ _ _ _ _ _ _ _ _ _] -> _
      tunnel: [_ _ _ _ _ _ _ "Round T2 X" _ "Delayed Interlace Start" _ _ _ _ _ _ _ _ _ _ _ _ _ _ _ _ _ _ _ _ _ _ _ _ _ _ _ _ _ _ _ _ _ _ _ _ _] -> _
      tunnel: [_ "Rescale on Mean" _ _ _ _ _ _ _ _ _ _ _ _ _ _ _ _ _ _ _ _ _ _ _ _ _ _ _ _ _ _ _ _ _ _ _ _ _ _ _ _ _ _ _ _ _] -> _
      tunnel: [_ _ _ _ _ _ _ _ _ _ _ _ _ _ _ _ _ _ _ _ _ _ _ _ _ _ _ _ _ _ _ _ _ _ _ _ _ _ _ _ _ _ _ _ _ _ "Flip Green Filter"] -> _
      event #0 {
        # "So that if 'Save ave N' is updated, the AOD scanning code updates too."
        n214 = event-data() -> ()  [unwired: 6 out]
        n215 = local read "AI Count (ticks)"() -> (w887:u32)
        n216 = local read "FPGA Ave."() -> (w891:dbl)
        n217 = Boolean To (0,1)(Boolean="Sets to FIFO (Traps)") -> (0, 1=w905:cluster{"Set 1":i16, "Set 2":i16, "Set 3":i16})
        n218 = xnode "Read/Write Control"("FPGA VI Reference In"=w917, "error in"=w915, "ai count"=w887, "AI1 Sets to FIFO"="Sets to FIFO (Traps)", "AI Averages"=w891, "N of AI1 Int Acq Sets"="N Acq Sets (Traps + Fl.)") -> ("error out"=w916:errorcluster)  [unwired: 1 out]
        n219 = Cluster To Array(cluster=w905) -> (array=w904:i16[])
        n220 = local read "Scan steps (AOD)"() -> (w906:u64)
        n221 = Multiply(x=w887, y="N Acq Sets (Traps + Fl.)") -> (x*y=w885:u32)
        n222 = Divide(x=40000000.0, y=w887) -> (x/y=w913:dbl)
        "AI rate (Hz)" <- w913
        n223 = Add Array Elements(numeric array=w904) -> (sum=w889:i16)
        "Trap Sets" <- w889
        n224 = Divide(x=w913, y=w891) -> (x/y=w914:dbl)
        "Ave. Rate (Hz)" <- w914
        n225 = Reciprocal(x=w914) -> (1/x=→"Ave. Period (s)":dbl)
        n226 = property on="Scan steps (AOD)" class="DigNum (strict)"("Val(Sgnl)"=w906) -> ()  [unwired: 2 in, 2 out]
        n227 = Divide(x=w914, y="N Acq Sets (Traps + Fl.)") -> (x/y=w910:dbl)
        "Data Rate (Hz)" <- w910
        n228 = Reciprocal(x=w910) -> (1/x=→"Data Period (s)":dbl)
        n229 = local read "Save ave N"() -> (w909:dbl)
        n230 = Divide(x=w910, y=w909) -> (x/y=w908:dbl)
        "Save Data Rate (Hz)" <- w908
        n231 = Reciprocal(x=w908) -> (1/x=→"Save Data Period (s)":dbl)
        n232 = Multiply(x=w885, y="# Samples/trap") -> (x*y=w881:dbl)
        "Counts/DMA" <- w881
        n233 = Multiply(x=w889, y="# Samples/trap") -> (x*y=w888:dbl)
        "# Samples/channel" <- w888
        n234 = Greater?(x=w891, y=1.0) -> (0:w894:bool)
        "FPGA Averaging" <- w894
        n235 = local read "APD Int. Count"() -> (w883:u32)
        n236 = Divide(x=w888, y=u32 2) -> (x/y=w897:dbl)
        n237 = Select(t=w888, s=w894, f=w897) -> (s? t:f=w902:dbl)
        n238 = Divide(x=w881, y=w883) -> (x/y=w882:dbl)
        "APD Samples/FIFO Acq." <- w882
        n239 = Divide(x=w881, y=40000000.0) -> (x/y=w879:dbl)
        "DMA Update Period (s)" <- w879
        n240 = Multiply(x=w902, y=u32 8) -> (x*y=→"Elements/DMA read":dbl)
        n241 = Multiply(x=2.0, y=w882) -> (x*y=→"APD Elements/DMA read":dbl)
        n242 = local read "N sets to save"() -> (w899:u32)
        n243 = Multiply(x=w879, y=w899) -> (x*y=→"Total Time (s)":dbl)
      }
      event #1 {
        n244 = event-data() -> ()  [unwired: 7 out]
        n245 = local read "Bead Mean (nm)"() -> (w1022:dbl)
        n246 = Add(x="Amplitude (nm)", y=w1022) -> (x+y=w1020:dbl)
        n247 = Subtract(x=w1022, y="Amplitude (nm)") -> (x-y=w1019:dbl)
        n248 = property on="Bead Separation" class="WFChart (strict)"("YScale.Minimum"=w1019) -> ()  [unwired: 2 in, 2 out]
        n249 = property on="Bead Separation" class="WFChart (strict)"("YScale.Maximum"=w1020) -> ()  [unwired: 2 in, 2 out]
      }
      event #2 {
        n250 = event-data() -> ()  [unwired: 7 out]
        n251 = local read "APD 1 Rate (Hz)"() -> (w1031:dbl)
        n252 = Multiply(x=1000.0, y="Above (kHz)") -> (x*y=w1029:dbl)
        n253 = Multiply(x=1000.0, y="Below (kHz)") -> (x*y=w1027:dbl)
        n254 = Add(x=w1029, y=w1031) -> (x+y=w1024:dbl)
        n255 = Subtract(x=w1031, y=w1027) -> (x-y=w1025:dbl)
        n256 = property on="APD 1 Chart" class="WFChart (strict)"("YScale.Minimum"=w1025) -> ()  [unwired: 2 in, 2 out]
        n257 = property on="APD 1 Chart" class="WFChart (strict)"("YScale.Maximum"=w1024) -> ()  [unwired: 2 in, 2 out]
      }
      event #3 {
        n258 = event-data() -> ()  [unwired: 7 out]
        n259 = Negate(x="Phase adj. (AI1)") -> (-x=w1041:i16)
        n260 = Select(t=w1041, s="- phase (AI1)", f="Phase adj. (AI1)") -> (s? t:f=w1040:i16)
        n261 = xnode "Read/Write Control"("FPGA VI Reference In"=w1044, "error in"=w1043, "Phase count adjustment"=w1040) -> ("FPGA VI Reference Out"=w1039:T15, "error out"=w1038:errorcluster)
        n262 = Or(x="- phase (AI1)", y="+ phase (AI1)") -> (x .or. y?=w1035:bool)
        n263 = xnode "Read/Write Control"("FPGA VI Reference In"=w1039, "error in"=w1038, "+ phase"=w1035) -> ("error out"=w1034:errorcluster)  [unwired: 1 out]
      }
      event #4 {
        w1120 = u32 9868950 ("Color Box")
        n264 = event-data() -> ("Row"=w1122:i32)  [unwired: 9 out]
        n265 = property on="All Signals" class="WFChart (strict)"("Active Plot"=w1122) -> (error out=w1133:errorcluster)  [unwired: 2 in, 1 out]
        n266 = property on="All Signals" class="WFChart (strict)" props=["Plot", "Visible?", "Plot", "Plot Color"](error in=w1133) -> (error out=w1132:errorcluster, "Plot.Visible?"=w1131:bool)  [unwired: 1 in, 2 out]
        n267 = Select(t=FALSE ("Plot.Visible"), s=w1131, f=TRUE ("Plot.Visible")) -> (s? t:f=w1126:bool)
        n268 = property on="All Signals" class="WFChart (strict)"(error in=w1132, "Plot.Visible?"=w1126) -> (error out=w1128:errorcluster)  [unwired: 1 in, 1 out]
        n269 = property on="All Signals" class="WFChart (strict)"(error in=w1128) -> (error out=w1123:errorcluster, "Plot.Plot Color"=w1127:u32)  [unwired: 1 in, 1 out]
        n270 = property on="Signals to Plot" class="LstBox (strict)"(error in=w1123, "Active Row"=w1122) -> (error out=w1121:errorcluster)  [unwired: 1 in, 1 out]
        n271 = Select(t=w1127, s=w1126, f=u32 0) -> (s? t:f=w1124:u32)
        n272 = property on="Signals to Plot" class="LstBox (strict)"(error in=w1121, "CellFontColor"=w1124, "SelColor"=w1120, "CellBG"=w1120, "CellFontSize"=u32 20 ("Active Row:Cell Font:Size"), "CellFontBold"=TRUE ("Active Row:Cell Font:Bold")) -> ()  [unwired: 1 in, 2 out]
      }
      event #5 {
        n273 = event-data() -> ("CtlRef"=w1136:refnum<vi>)  [unwired: 6 out]
        n274 = control-ref of="Trap Delta (MHz)"() -> (w1135:refnum<vi>)
        n275 = Equal?(x=w1135, y=w1136) -> (x = y?=w1134:bool)
        n276 = case shown="False" "Oscillate Set 1" {
          tunnel: w1139 -> [w1159 _]
          tunnel: [w1158 w1162] -> w1138
          tunnel: w1137 -> [w1157 w1162]
          tunnel: w1134 -> [w1142 _]
          frame #0 {
            n277 = local read "BD 1 Frequency 2 (MHz)"() -> (w1146:dbl)
            n278 = local read "BD 1 Frequency 1 (MHz)"() -> (w1144:dbl)
            n279 = Subtract(x=w1146, y="Trap Delta (MHz)") -> (x-y=w1143:dbl)
            n280 = Select(t=w1143, s=w1142, f=w1144) -> (s? t:f=w1141:dbl)
            n281 = local read "Y RF Frequency Limits (MHz)"() -> (w1147:T12)
            n282 = local read "X RF Frequency Limits (MHz)"() -> (w1148:T12)
            n283 = local read "BD 1 Frequency 3 (MHz)"() -> (w1160:dbl)
            n284 = local write "BD 1 Frequency 1 (MHz)"(w1141) -> ()
            n285 = local read "BD 2 Frequency 1 (MHz)"() -> (w1151:dbl)
            n286 = local read "BD 2 Frequency 2 (MHz)"() -> (w1150:dbl)
            n287 = local read "BD 2 Frequency 3 (MHz)"() -> (w1161:dbl)
            n288 = call "set RF board frequency - interlace.vi"("Board 2 Frequency Limits"=w1147, "Board 1 Frequency Limits"=w1148, "error in"=w1157, "FPGA VI Reference In"=w1159, "Board 2 Frequency 3 (MHz)"=w1161, "Board 1 Frequency 3 (MHz)"=w1160, "Board 2 Frequency 2 (MHz)"=w1150, "Board 2 Frequency 1 (MHz)"=w1151, "Board 1 Frequency 2 (MHz)"=w1146, "Board 1 Frequency 1  (MHz)"=w1141) -> ("error out"=w1158:errorcluster)  [unwired: 1 out]
            n289 = Subtract(x=w1151, y=w1150) -> (x-y=w1155:dbl)
            n290 = Subtract(x=w1141, y=w1146) -> (x-y=w1156:dbl)
            n291 = Square(x=w1155) -> (x^2=w1153:dbl)
            n292 = Square(x=w1156) -> (x^2=w1154:dbl)
            n293 = Add(x=w1154, y=w1153) -> (x+y=w1152:dbl)
            n294 = Square Root(x=w1152) -> (sqrt(x)=w1149:dbl)
            n295 = local write "Trap Delta (MHz)"(w1149) -> ()
            n296 = property on="Initial delta (MHz)" class="DigNum (strict)"("Val(Sgnl)"=w1149) -> ()  [unwired: 2 in, 2 out]
          }
          frame #1 {
          }
        }
      }
      event #6 {
        n297 = event-data() -> ()  [unwired: 7 out]
        n298 = local read "BD 1 Frequency 1 (MHz)"() -> (w1165:dbl)
        n299 = Round To Nearest(number=w1165) -> (nearest integer value=w1164:dbl)
        n300 = property on="BD 1 Frequency 1 (MHz)" class="DigNum (strict)"("Val(Sgnl)"=w1164) -> ()  [unwired: 2 in, 2 out]
      }
      event #7 {
        n301 = event-data() -> ()  [unwired: 7 out]
        n302 = local read "BD 1 Frequency 2 (MHz)"() -> (w1167:dbl)
        n303 = Round To Nearest(number=w1167) -> (nearest integer value=w1166:dbl)
        n304 = property on="BD 1 Frequency 2 (MHz)" class="DigNum (strict)"("Val(Sgnl)"=w1166) -> ()  [unwired: 2 in, 2 out]
      }
      event #8 {
        n305 = event-data() -> ()  [unwired: 7 out]
        n306 = local read "Stop All"() -> (w1169:bool)
      }
      event #9 {
        n307 = event-data() -> ()  [unwired: 7 out]
        n308 = flat-sequence {
          frame #0 {
            n309 = Multiply(x="Delay to Interlace (s)", y=1000.0) -> (x*y=w1172:dbl)
            n310 = Wait (ms)(milliseconds to wait=w1172) -> ()  [unwired: 1 out]
          }
          frame #1 {
            n311 = property on="Green laser mode" class="RadioBtnsControl (strict)"("Val(Sgnl)"=enum32{"Laser ON", "Laser OFF", "Interlace"}."Interlace" ("Value (Signaling)")) -> ()  [unwired: 2 in, 2 out]
          }
        }
      }
      event #10 {
        w1196 = i16 1 ("f")
        n312 = event-data() -> ()  [unwired: 7 out]
        n313 = local write "Trap 1 (ON/OFF)"("Trap 1 ON") -> ()
        n314 = local write "Trap 2 (ON/OFF)"("Trap 2 ON") -> ()
        n315 = Boolean To (0,1)(Boolean="Trap 3 ON") -> (0, 1=w1197:i16)
        n316 = Boolean To (0,1)(Boolean="Trap 1 ON") -> (0, 1=w1198:i16)
        n317 = Boolean To (0,1)(Boolean="Trap 2 ON") -> (0, 1=w1199:i16)
        n318 = Select(t=w1199, s="Trap ON/OFF X or Y Amp?", f=w1196) -> (s? t:f=w1194:i16)
        n319 = Select(t=w1198, s="Trap ON/OFF X or Y Amp?", f=w1196) -> (s? t:f=w1195:i16)
        n320 = Select(t=w1197, s="Trap ON/OFF X or Y Amp?", f=w1196) -> (s? t:f=w1193:i16)
        n321 = Select(t=w1196, s="Trap ON/OFF X or Y Amp?", f=w1199) -> (s? t:f=w1191:i16)
        n322 = Select(t=w1196, s="Trap ON/OFF X or Y Amp?", f=w1198) -> (s? t:f=w1192:i16)
        n323 = Select(t=w1196, s="Trap ON/OFF X or Y Amp?", f=w1197) -> (s? t:f=w1190:i16)
        n324 = And(x="All FB On/Off", y="Feedback On/Off") -> (x .and. y?=w1188:cluster{"Set 1":bool, "Set 2":bool})
        n325 = local read "BD 1 Amplitude 1 (%)"() -> (w1208:dbl)
        n326 = local read "BD 1 Amplitude 2 (%)"() -> (w1207:dbl)
        n327 = local read "BD 1 Amplitude 3 (%)"() -> (w1206:dbl)
        n328 = Unbundle By Name(w1188) -> ("Set 1"=w1183:bool, "Set 2"=w1180:bool)
        n329 = local read "Y RF Amplitude Limits (%)"() -> (w1176:T12)
        n330 = local read "X RF Amplitude Limits (%)"() -> (w1177:T12)
        n331 = local read "BD 2 Amplitude 1 (%)"() -> (w1209:dbl)
        n332 = local read "BD 2 Amplitude 2 (%)"() -> (w1210:dbl)
        n333 = local read "BD 2 Amplitude 3 (%)"() -> (w1211:dbl)
        n334 = And(x="Trap 2 ON", y=w1180) -> (x .and. y?=w1178:bool)
        n335 = And(x="Trap 1 ON", y=w1183) -> (x .and. y?=w1181:bool)
        n336 = Multiply(x=w1195, y=w1208) -> (x*y=w1203:dbl)
        n337 = Multiply(x=w1207, y=w1194) -> (x*y=w1201:dbl)
        n338 = Multiply(x=w1206, y=w1193) -> (x*y=w1202:dbl)
        n339 = Multiply(x=w1209, y=w1192) -> (x*y=w1212:dbl)
        n340 = Multiply(x=w1210, y=w1191) -> (x*y=w1213:dbl)
        n341 = Multiply(x=w1211, y=w1190) -> (x*y=w1214:dbl)
        n342 = call "set RF board amplitude - interlace.vi"("Board 2 Amplitude Limits"=w1176, "Board 1 Amplitude Limits"=w1177, "error in"=w1204, "FPGA VI Reference In"=w1205, "Board 2 Amplitude 3 (%)"=w1214, "Board 1 Amplitude 3 (%)"=w1202, "Board 2 Amplitude 2 (%)"=w1213, "Board 2 Amplitude 1 (%)"=w1212, "Board 1 Amplitude 2 (%)"=w1201, "Board 1 Amplitude 1 (%)"=w1203) -> ("error out"=w1185:errorcluster, "FPGA VI Reference Out"=w1186:T15)
        n343 = xnode "Read/Write Control"("FPGA VI Reference In"=w1186, "error in"=w1185, "FB On/Off Set 1"=w1181, "FB On/Off Set 2"=w1178) -> ("error out"=w1184:errorcluster)  [unwired: 1 out]
      }
      event #11 {
        n344 = event-data() -> ()  [unwired: 7 out]
        n345 = local read "Current Stage  Position"() -> (w1275:cluster{dbl, dbl, dbl})
        n346 = local read "Saved Stage Positions"() -> (w1274:T4)
        n347 = Bundle By Name(cluster=w1274, "Position 1"=w1275) -> (w1273:T4)
        n348 = local write "Saved Stage Positions"(w1273) -> ()
      }
      event #12 {
        n349 = event-data() -> ()  [unwired: 7 out]
        n350 = local read "Current Stage  Position"() -> (w1279:cluster{dbl, dbl, dbl})
        n351 = local read "Saved Stage Positions"() -> (w1278:T4)
        n352 = Bundle By Name(cluster=w1278, "Position 2"=w1279) -> (w1277:T4)
        n353 = local write "Saved Stage Positions"(w1277) -> ()
      }
      event #13 {
        n354 = event-data() -> ()  [unwired: 7 out]
        n355 = local read "Saved Stage Positions"() -> (w1283:T4)
        n356 = local read "Current Stage  Position"() -> (w1282:cluster{dbl, dbl, dbl})
        n357 = Bundle By Name(cluster=w1283, "Position 3"=w1282) -> (w1281:T4)
        n358 = local write "Saved Stage Positions"(w1281) -> ()
      }
      event #14 {
        n359 = event-data() -> ()  [unwired: 7 out]
        n360 = local read "Current Stage  Position"() -> (w1286:cluster{dbl, dbl, dbl})
        n361 = local read "Saved Stage Positions"() -> (w1287:T4)
        n362 = Bundle By Name(cluster=w1287, "Position 4"=w1286) -> (w1285:T4)
        n363 = local write "Saved Stage Positions"(w1285) -> ()
      }
      event #15 {
        n364 = event-data() -> ()  [unwired: 7 out]
        n365 = local read "Current Stage  Position"() -> (w1290:cluster{dbl, dbl, dbl})
        n366 = local read "Saved Stage Positions"() -> (w1291:T4)
        n367 = Bundle By Name(cluster=w1291, "Position 5"=w1290) -> (w1289:T4)
        n368 = local write "Saved Stage Positions"(w1289) -> ()
      }
      event #16 {
        n369 = event-data() -> ()  [unwired: 7 out]
        n370 = property on="Saved AOD Raster Scan Parameter Sets" class="Arr (strict)"() -> ("Index Values"=w1301:u32[])  [unwired: 2 in, 2 out]
        n371 = Index Array(array=w1301, index=0) -> (element=w1298:u32)
        n372 = Index Array(array="Saved AOD Raster Scan Parameter Sets", index=w1298) -> (element=w1297:T23)
        n373 = Unbundle By Name(w1297) -> ("Scan Range AOD (nm) 2"=w1296:dbl, "Step Size AOD (nm) 2"=w1295:dbl, "Scan Speed AOD (nm/s) 2"=w1294:dbl, "Number of scans (AOD) 2"=w1293:u16)
        n374 = flat-sequence {
          tunnel: w1296 -> [w1305]
          tunnel: w1295 -> [w1304]
          tunnel: w1294 -> [w1303]
          tunnel: w1293 -> [w1306]
          frame #0 {
            n375 = local write "Scan Speed (nm/s)"(w1303) -> ()
            n376 = local write "Scan Range (nm)"(w1305) -> ()
            n377 = local write "Step Size (nm)"(w1304) -> ()
          }
          frame #1 {
            n378 = property on="Number of F/B Scans (AOD)" class="DigNum (strict)"("Val(Sgnl)"=w1306) -> ()  [unwired: 2 in, 2 out]
          }
        }
      }
      event #17 {
        n379 = event-data() -> ()  [unwired: 7 out]
        n380 = property on="Trap 2 ON" class="Bool (strict)"("Val(Sgnl)"="Trap 2 (ON/OFF)") -> ()  [unwired: 2 in, 2 out]
        n381 = property on="Trap 1 ON" class="Bool (strict)"("Val(Sgnl)"="Trap 1 (ON/OFF)") -> ()  [unwired: 2 in, 2 out]
      }
      event #18 {
        n382 = event-data() -> ()  [unwired: 7 out]
        n383 = local read "DIO count 3 (ticks)"() -> (w1319:u32)
        n384 = local read "DIO count 1 (ticks)"() -> (w1321:u32)
        n385 = local read "DIO count 2 (ticks)"() -> (w1320:u32)
        n386 = To Unsigned Byte Integer(number="Not-Interlacing Set") -> (unsigned 8bit integer=w1310:u8)
        n387 = Add(x=w1310, y=u8 1) -> (x+y=w1314:u8)
        n388 = xnode "Read/Write Control"("FPGA VI Reference In"=w1325, "error in"=w1323, "DIO count 1 (ticks)"=w1321, "DIO count 2 (ticks)"=w1320, "DIO count 3 (ticks)"=w1319, "Interlace ON/OFF"="Interlace", "Number Interlace Cycles"="Number Interlace Sets", "Interlace Off Parameters"=w1314) -> ("error out"=w1324:errorcluster)  [unwired: 1 out]
        n389 = Build Array(w1321, w1320, w1319) -> (w1312:u32[])
        n390 = Split 1D Array(array=w1312, index="Number Interlace Sets") -> (first subarray=w1322:u32[])  [unwired: 1 out]
        n391 = Index Array(array=w1312, index=w1310) -> (element=w1311:u32)
        n392 = Add Array Elements(numeric array=w1322) -> (sum=w1316:u32)
        n393 = Select(t=w1316, s="Interlace", f=w1311) -> (s? t:f=→"Total Counts (ticks)":u32)
      }
      event #19 {
        n394 = event-data() -> ()  [unwired: 7 out]
        n395 = Unbundle By Name("Reset Feedback") -> ("Set 1"=w1461:bool, "Set 2"=w1460:bool)
        n396 = xnode "Read/Write Control"("FPGA VI Reference In"=w1463, "error in"=w1458, "FB Reset Set 1"=w1461, "FB Reset Set 2"=w1460) -> ("error out"=w1459:errorcluster)  [unwired: 1 out]
      }
      event #20 {
        n397 = event-data() -> ()  [unwired: 7 out]
        n398 = Unbundle By Name("PID Gains") -> ("Set 1"=w1524:T10, "Set 2"=w1523:T10)
        n399 = xnode "Read/Write Control"("FPGA VI Reference In"=w1525, "error in"=w1521, "FB Gains Set 1"=w1524, "FB Gains Set 2"=w1523) -> ("error out"=w1522:errorcluster)  [unwired: 1 out]
      }
      event #21 {
        n400 = event-data() -> ()  [unwired: 7 out]
        n401 = xnode "Read/Write Control"("FPGA VI Reference In"=w1568, "error in"=w1564) -> ("FPGA VI Reference Out"=w1567:T15, "error out"=w1566:errorcluster, "AI2 Y Sum Set 1"=w1575:i16, "AI2 Y Sum Set 2"=w1574:i16)
        n402 = Cluster To Array(cluster="AI2 to Setpoint") -> (array=w1578:bool[])
        n403 = local read "AI2 (V)"() -> (w1576:cluster{"Set 1":dbl, "Set 2":dbl})
        n404 = Or Array Elements(Boolean array=w1578) -> (logical OR=w1579:bool)
        n405 = Bundle By Name(cluster=w1576, "Set 1"=w1575, "Set 2"=w1574) -> (w1573:cluster{"Set 1":dbl, "Set 2":dbl})
        n406 = Divide(x=w1573, y=3276.7) -> (x/y=w1572:cluster{"Set 1":dbl, "Set 2":dbl})
        "AI2 (V)" <- w1572
        n407 = case shown="True" w1579 {
          tunnel: [w1641 w1658] -> w1571
          tunnel: "AI2 to Setpoint" -> [_ w1654]
          tunnel: "Setpoints (V)" -> [w1642 w1657]
          tunnel: w1572 -> [_ w1651]
          frame #0 {
            n408 = Multiply(x=3276.7, y=w1642) -> (x*y=w1643:cluster{"Set 1":dbl, "Set 2":dbl})
            n409 = To Word Integer(number=w1643) -> (16bit integer=w1641:cluster{"Set 1":i16, "Set 2":i16})
          }
          frame #1 {
            n410 = Unbundle By Name(w1651) -> ("Set 1"=w1650:dbl, "Set 2"=w1649:dbl)
            n411 = Unbundle By Name(w1657) -> ("Set 1"=w1656:dbl, "Set 2"=w1655:dbl)
            n412 = Unbundle By Name(w1654) -> ("Set 1"=w1653:bool, "Set 2"=w1652:bool)
            n413 = Select(t=w1650, s=w1653, f=w1656) -> (s? t:f=w1648:dbl)
            n414 = Select(t=w1649, s=w1652, f=w1655) -> (s? t:f=w1647:dbl)
            n415 = Bundle By Name(cluster=w1657, "Set 1"=w1648, "Set 2"=w1647) -> (w1645:cluster{"Set 1":dbl, "Set 2":dbl})
            n416 = Multiply(x=3276.7, y=w1645) -> (x*y=w1646:cluster{"Set 1":dbl, "Set 2":dbl})
            n417 = local write "Setpoints (V)"(w1645) -> ()
            n418 = To Word Integer(number=w1646) -> (16bit integer=w1658:cluster{"Set 1":i16, "Set 2":i16})
          }
        }
        n419 = Unbundle By Name(w1571) -> ("Set 1"=w1570:i16, "Set 2"=w1569:i16)
        n420 = xnode "Read/Write Control"("FPGA VI Reference In"=w1567, "error in"=w1566, "FB Setpoint Set 1"=w1570, "FB Setpoint Set 2"=w1569) -> ("error out"=w1565:errorcluster)  [unwired: 1 out]
      }
      event #22 {
        n421 = event-data() -> ()  [unwired: 7 out]
        n422 = xnode "Read/Write Control"("FPGA VI Reference In"=w1718, "error in"=w1716, "Invert GI"="Invert GI", "Invert GI 2"="Invert GI") -> ("error out"=w1717:errorcluster)  [unwired: 1 out]
      }
      event #23 {
        n423 = event-data() -> ()  [unwired: 7 out]
        n424 = local read "Green FB Setpoint (mV)"() -> (w1782:dbl)
        n425 = local read "Current When FB OFF (%)"() -> (w1785:dbl)
        n426 = Multiply(x=w1782, y=3.2767) -> (x*y=w1781:dbl)
        n427 = Multiply(x=w1785, y=655.35) -> (x*y=w1786:dbl)
        n428 = To Unsigned Word Integer(number=w1786) -> (unsigned 16bit integer=w1784:u16)
        n429 = local read "Green int current ON count adj"() -> (w1789:u32)
        n430 = local read "Green FB Gains"() -> (w1788:T10)
        n431 = local read "Green Laser ON/Interlacing"() -> (w1779:bool)
        n432 = local read "Green laser mode"() -> (w1778:enum32{"Laser ON", "Laser OFF", "Interlace"})
        n433 = local read "Green FB On/Off"() -> (w1790:bool)
        n434 = Equal?(x=w1778, y=enum32{"Laser ON", "Laser OFF", "Interlace"}."Interlace") -> (x = y?=w1776:bool)
        n435 = Compound Arithmetic op=AND(w1776, w1790, w1779) -> (w1780:bool)
        n436 = xnode "Read/Write Control"("FPGA VI Reference In"=w1793, "error in"=w1792, "Green FB Setpoint"=w1781, "Green FB On/Off"=w1780, "Current Out"=w1784, "Green int current ON count adj"=w1789, "Green FB Gains"=w1788) -> ("error out"=w1791:errorcluster)  [unwired: 1 out]
      }
      event #24 {
        n437 = event-data() -> ()  [unwired: 7 out]
        n438 = case shown="True" "Green Laser ON/Interlacing" {
          tunnel: "Green laser mode" -> [_ w1911]
          tunnel: [enum32{"Laser ON", "Laser OFF", "Interlace"}."Laser OFF" ("Green laser mode") w1911] -> w1899
          tunnel: [FALSE w1907] -> w1898
          frame #0 {
          }
          frame #1 {
            n439 = local read "Green FB On/Off"() -> (w1908:bool)
            n440 = Equal?(x=w1911, y=enum32{"Laser ON", "Laser OFF", "Interlace"}."Interlace") -> (x = y?=w1909:bool)
            n441 = And(x=w1909, y=w1908) -> (x .and. y?=w1907:bool)
          }
        }
        n442 = xnode "Read/Write Control"("FPGA VI Reference In"=w1904, "error in"=w1902, "Operating Mode"=w1899, "Operating Mode 2"=w1899, "Green FB On/Off"=w1898) -> ("error out"=w1903:errorcluster)  [unwired: 1 out]
      }
      event #25 {
        n443 = event-data() -> ()  [unwired: 7 out]
        n444 = local read "Phase Adj. (APD Gate)"() -> (w1987:i16)
        n445 = Negate(x=w1987) -> (-x=w1995:i16)
        n446 = Select(t=w1995, s="- phase (APD Gate)", f=w1987) -> (s? t:f=w1994:i16)
        n447 = Or(x="- phase (APD Gate)", y="+ phase (APD Gate)") -> (x .or. y?=w1990:bool)
        n448 = xnode "Read/Write Control"("FPGA VI Reference In"=w1997, "error in"=w1996, "Phase count adjustment (APD Gate)"=w1994) -> ("FPGA VI Reference Out"=w1992:T15, "error out"=w1993:errorcluster)
        n449 = xnode "Read/Write Control"("FPGA VI Reference In"=w1992, "error in"=w1993, "+ phase (APD Gate)"=w1990) -> ("error out"=w1991:errorcluster)  [unwired: 1 out]
      }
      event #26 {
        n450 = event-data() -> ()  [unwired: 7 out]
        n451 = local read "Phase Adj. (APD Acq)"() -> (w2073:i16)
        n452 = Negate(x=w2073) -> (-x=w2079:i16)
        n453 = Select(t=w2079, s="+ phase (APD Acq)", f=w2073) -> (s? t:f=w2078:i16)
        n454 = Or(x="+ phase (APD Acq)", y="- phase (APD Acq)") -> (x .or. y?=w2074:bool)
        n455 = xnode "Read/Write Control"("FPGA VI Reference In"=w2081, "error in"=w2080, "Phase Count Adjustment (APD Acq)"=w2078) -> ("FPGA VI Reference Out"=w2076:T15, "error out"=w2077:errorcluster)
        n456 = xnode "Read/Write Control"("FPGA VI Reference In"=w2076, "error in"=w2077, "+ phase (APD Acq)"=w2074) -> ("error out"=w2075:errorcluster)  [unwired: 1 out]
      }
      event #27 {
        n457 = event-data() -> ()  [unwired: 7 out]
        n458 = Negate(x="Phase adj. (GI)") -> (-x=w2163:i16)
        n459 = Select(t=w2163, s="+ phase (GI)", f="Phase adj. (GI)") -> (s? t:f=w2162:i16)
        n460 = Or(x="+ phase (GI)", y="- phase (GI)") -> (x .or. y?=w2158:bool)
        n461 = xnode "Read/Write Control"("FPGA VI Reference In"=w2165, "error in"=w2164, "Phase count adjustment (GI)"=w2162) -> ("FPGA VI Reference Out"=w2160:T15, "error out"=w2161:errorcluster)
        n462 = xnode "Read/Write Control"("FPGA VI Reference In"=w2160, "error in"=w2161, "+ phase (GI)"=w2158) -> ("error out"=w2159:errorcluster)  [unwired: 1 out]
      }
      event #28 {
        n463 = event-data() -> ()  [unwired: 7 out]
        n464 = Negate(x="Phase adj. (GI) 2") -> (-x=w2247:i16)
        n465 = Select(t=w2247, s="+ phase (GI) 2", f="Phase adj. (GI) 2") -> (s? t:f=w2246:i16)
        n466 = Or(x="+ phase (GI) 2", y="- phase (GI) 2") -> (x .or. y?=w2242:bool)
        n467 = xnode "Read/Write Control"("FPGA VI Reference In"=w2249, "error in"=w2248, "Phase count adjustment (GI) 2"=w2246) -> ("FPGA VI Reference Out"=w2244:T15, "error out"=w2245:errorcluster)
        n468 = xnode "Read/Write Control"("FPGA VI Reference In"=w2244, "error in"=w2245, "+ phase (GI) 2"=w2242) -> ("error out"=w2243:errorcluster)  [unwired: 1 out]
      }
      event #29 {
        n469 = event-data() -> ()  [unwired: 7 out]
        n470 = Negate(x="Phase adj. (Green FB)") -> (-x=w2331:i16)
        n471 = Select(t=w2331, s="+ phase (Green FB)", f="Phase adj. (Green FB)") -> (s? t:f=w2330:i16)
        n472 = Or(x="+ phase (Green FB)", y="- phase (Green FB)") -> (x .or. y?=w2326:bool)
        n473 = xnode "Read/Write Control"("FPGA VI Reference In"=w2333, "error in"=w2332, "Phase count adjustment (Green FB)"=w2330) -> ("FPGA VI Reference Out"=w2328:T15, "error out"=w2329:errorcluster)
        n474 = xnode "Read/Write Control"("FPGA VI Reference In"=w2328, "error in"=w2329, "+ phase (Green FB)"=w2326) -> ("error out"=w2327:errorcluster)  [unwired: 1 out]
      }
      event #30 {
        n475 = event-data() -> ()  [unwired: 7 out]
        n476 = local read "APD Integration Time (s)"() -> (w2407:dbl)
        n477 = local read "APD Gate ON Count"() -> (w2422:u32)
        n478 = local read "APD Gate OFF Count"() -> (w2421:u32)
        n479 = local read "Invert APD Gate"() -> (w2423:bool)
        n480 = local read "APD Gate"() -> (w2420:enum32{"ON", "OFF", "Interlace"})
        n481 = Multiply(x=w2407, y=40000000.0) -> (x*y=w2418:dbl)
        n482 = Reciprocal(x=w2407) -> (1/x=→"APD Acq Rate (Hz)":dbl)
        n483 = To Unsigned Long Integer(number=w2418) -> (unsigned 32bit integer=w2417:u32)
        n484 = local read "DMA Update Period (s)"() -> (w2408:dbl)
        n485 = Divide(x=w2408, y=w2407) -> (x/y=w2411:dbl)
        n486 = local read "APD 1 AO offset"() -> (w2413:i16)
        n487 = local read "APD 1 AO Mult."() -> (w2415:i16)
        n488 = local read "APD 2 AO Mult."() -> (w2414:i16)
        n489 = local read "APD 2 AO offset"() -> (w2412:i16)
        n490 = Multiply(x=2.0, y=w2411) -> (x*y=w2410:dbl)
        n491 = local write "APD Samples/FIFO Acq."(w2411) -> ()
        n492 = local write "APD Elements/DMA read"(w2410) -> ()
        n493 = xnode "Read/Write Control"("FPGA VI Reference In"=w2426, "error in"=w2425, "Invert APD Gate"=w2423, "APD Gate ON Count"=w2422, "APD Gate OFF Count"=w2421, "APD Acq Rate Count"=w2417, "APD Gate Operating Mode"=w2420, "APD 1 AO scale factor"=w2415, "APD 2 AO scale factor"=w2414, "APD 1 AO offset"=w2413, "APD 2 AO offset"=w2412) -> ("error out"=w2424:errorcluster)  [unwired: 1 out]
      }
      event #31 {
        n494 = event-data() -> ()  [unwired: 7 out]
        n495 = xnode "Read/Write Control"("FPGA VI Reference In"=w2621, "error in"=w2619, "Green interlace ON count"="GI Frequency, ON count", "Green interlace OFF count"="GI Frequency, OFF count", "Green interlace ON count 2"="GI Frequency, ON count", "Green interlace OFF count 2"="GI Frequency, OFF count", "Green FB Count"="Green FB Count") -> ("error out"=w2620:errorcluster)  [unwired: 1 out]
      }
      event #32 {
        w2789 = 123.0  # AOM cal (nm/MHz)
        n496 = event-data() -> ()  [unwired: 7 out]
        n497 = local read "BD 1 Frequency 1 (MHz)"() -> (w2772:dbl)
        n498 = local read "AOM X Cal (nm/MHz)"() -> (w2764:dbl)
        n499 = local read "X RF Frequency Limits (MHz)"() -> (w2776:T12)
        n500 = local read "Y RF Frequency Limits (MHz)"() -> (w2773:T12)
        n501 = local read "BD 2 Frequency 1 (MHz)"() -> (w2778:dbl)
        n502 = Negate(x="Scan Range (nm)") -> (-x=w2741:dbl)
        n503 = Divide(x=w2741, y=w2764) -> (x/y=w2745:dbl)
        n504 = Select(t=w2776, s="Scan BD", f=w2773) -> (s? t:f=w2775:T12)
        n505 = Select(t=w2772, s="Scan BD", f=w2778) -> (s? t:f=w2777:dbl)
        n506 = Unbundle By Name(w2775) -> ("Maximum"=w2784:dbl, "Minimum"=w2783:dbl)
        n507 = Add(x=w2745, y=w2777) -> (x+y=w2781:dbl)
        n508 = Divide(x=w2741, y="Step Size (nm)") -> (x/y=w2761:dbl)
        n509 = Divide(x="Step Size (nm)", y=w2764) -> (x/y=w2770:dbl)
        n510 = Absolute Value(x=w2761) -> (abs(x)=w2744:dbl)
        n511 = Sign(1:w2741) -> (0:w2742:dbl)
        n512 = In Range and Coerce(upper limit=w2784, x=w2781, lower limit=w2783) -> (coerced(x)=w2780:dbl, In Range?=w2782:bool)
        n513 = To Unsigned Quad Integer(1:w2744) -> (0:w2760:u64)
        "Scan steps (AOD)" <- w2760
        n514 = call "IR AOM freq to word.vi"("Frequency In (MHz)"=w2770) -> ("Frequency Word Out (double)"=w2767:dbl)
        n515 = Multiply(x=w2742, y=w2767) -> (x*y=w2743:dbl)
        n516 = Subtract(x=w2781, y=w2780) -> (x-y=w2779:dbl)
        n517 = To Quad Integer(1:w2743) -> (0:w2766:i64)
        "Incr. int (AOD)" <- w2766
        n518 = Subtract(x=w2745, y=w2779) -> (x-y=w2765:dbl)
        "Scan Range (MHz)" <- w2765
        n519 = Select(t=w2745, s=w2782, f=w2765) -> (s? t:f=w2785:dbl)
        n520 = Multiply(x=w2765, y=w2764) -> (x*y=w2763:dbl)
        n521 = Decrement(x=w2760) -> (x-1=w2813:u64)
        n522 = Negate(x=w2763) -> (-x=w2759:dbl)
        n523 = local write "Scan Range (nm)"(w2759) -> ()
        n524 = Divide(x=w2785, y=w2813) -> (x/y=w2769:dbl)
        "Scan Increment (MHz)" <- w2769
        n525 = call "IR AOM freq to word.vi"("Frequency In (MHz)"=w2769) -> ("Frequency Word Out (double)"=w2768:dbl)
        n526 = Divide(x="Step Size (nm)", y="Scan Speed (nm/s)") -> (x/y=w2756:dbl)
        n527 = To Quad Integer(1:w2768) -> ()  [unwired: 1 out]
        n528 = local read "Number Interlace Sets"() -> (w2739:u8)
        n529 = local read "AI Count (ticks)"() -> (w2740:u32)
        n530 = local read "Total Counts (ticks)"() -> (w2738:u32)
        n531 = local read "# Samples/trap"() -> (w2771:dbl)
        n532 = Multiply(x=w2740, y=w2739) -> (x*y=w2737:u32)
        n533 = Divide(x=w2738, y=w2737) -> (x/y=w2736:dbl)
        n534 = Select(t=w2772, s="Scan BD", f=w2778) -> (s? t:f=w2810:dbl)
        "Initial freq. (MHz)" <- w2810
        n535 = Add(x=w2785, y=w2810) -> (x+y=→"Final freq. (MHz)":dbl)
        n536 = Divide(x=w2738, y=40000000.0) -> (x/y=w2755:dbl)
        n537 = Divide(x=w2756, y=w2755) -> (x/y=w2754:dbl)
        n538 = To Unsigned Quad Integer(1:w2754) -> (0:w2753:u64)
        "Cycles/step (AOD)" <- w2753
        n539 = xnode "Read/Write Control"("FPGA VI Reference In"=w2821, "error in"=w2820, "Scan steps"=w2760, "Number of scans"="Number of F/B Scans (AOD)", "Cycles per step"=w2753, "Scan freq.  increment"=w2766, "Scan BD"="Scan BD") -> ("error out"=w2819:errorcluster)  [unwired: 1 out]
        n540 = Multiply(x=w2760, y=w2753) -> (x*y=w2814:u64)
        n541 = Multiply(x=w2814, y=u64 2) -> (x*y=w2735:u64)
        n542 = Multiply(x=w2736, y=w2735) -> (x*y=w2734:dbl)
        "Data points/scan (f/b)" <- w2734
        n543 = Multiply(x=w2734, y="Number of F/B Scans (AOD)") -> (x*y=w2817:dbl)
        "Data points/scans" <- w2817
        n544 = Divide(x=w2817, y=w2771) -> (x/y=→"N sets should be saved":dbl)
        n545 = Multiply(x=w2814, y=w2755) -> (x*y=w2752:dbl)
        "Time/Scan (s) (AOD)" <- w2752
        n546 = Select(t=w2785, s="Scan BD", f=0.0) -> (s? t:f=w2811:dbl)
        n547 = Select(t=0.0, s="Scan BD", f=w2785) -> (s? t:f=w2807:dbl)
        n548 = local read "BD 2 Frequency 2 (MHz)"() -> (w2803:dbl)
        n549 = local read "BD 1 Frequency 2 (MHz)"() -> (w2806:dbl)
        n550 = Add(x=w2807, y=w2778) -> (x+y=w2804:dbl)
        n551 = Add(x=w2772, y=w2811) -> (x+y=w2805:dbl)
        n552 = Multiply(x=w2752, y=2.0) -> (x*y=w2751:dbl)
        n553 = Multiply(x=w2751, y="Number of F/B Scans (AOD)") -> (x*y=w2748:dbl)
        n554 = Divide(x=w2748, y=60.0) -> (x/y=→"Time to Finish All (min)":dbl)
        n555 = Add(x="Trap 2 Bead Size (nm)", y="Trap 1 Bead Size (nm)") -> (x+y=w2793:dbl)
        n556 = Divide(x=w2793, y=2.0) -> (x/y=w2787:dbl)
        n557 = Subtract(x=w2804, y=w2803) -> (x-y=w2801:dbl)
        n558 = Subtract(x=w2805, y=w2806) -> (x-y=w2802:dbl)
        n559 = local read "Initial delta (MHz)"() -> (w2790:dbl)
        n560 = Square(x=w2801) -> (x^2=w2800:dbl)
        n561 = Square(x=w2802) -> (x^2=w2799:dbl)
        n562 = Add(x=w2799, y=w2800) -> (x+y=w2798:dbl)
        n563 = Square Root(x=w2798) -> (sqrt(x)=w2797:dbl)
        "Final delta (MHz)" <- w2797
        n564 = Multiply(x=w2789, y=w2797) -> (x*y=w2796:dbl)
        n565 = Multiply(x=w2790, y=w2789) -> (x*y=w2788:dbl)
        n566 = Subtract(x=w2788, y=w2787) -> (x-y=→"Initial sep (nm)":dbl)
        n567 = Subtract(x=w2796, y=w2787) -> (x-y=→"Final sep (nm)":dbl)
      }
      event #33 {
        n568 = event-data() -> ()  [unwired: 7 out]
        n569 = local read "Freq or Amp switch first"() -> (w2908:bool)
        n570 = local read "Amp switch delay"() -> (w2909:u16)
        n571 = local read "Freq switch delay"() -> (w2911:u16)
        n572 = local read "Swap F1 and F2"() -> (w2910:bool)
        n573 = xnode "Read/Write Control"("FPGA VI Reference In"=w2914, "error in"=w2913, "Freq switch delay"=w2911, "Swap F1 and F2"=w2910, "Amp switch delay"=w2909, "Freq or Amp switch first"=w2908) -> ("error out"=w2912:errorcluster)  [unwired: 1 out]
      }
      event #34 {
        w3011 = 32767.0 ("y")
        n574 = event-data() -> ()  [unwired: 7 out]
        n575 = Select(t="Scan lines (y)", s="2D or 1D Scan", f="Number of scans (MCL)") -> (s? t:f=w3016:u64)
        n576 = Decrement(x="Scan steps (MCL)") -> (x-1=w3032:u64)
        n577 = Divide(x="Scan Range (V)\n(of steps)", y=w3032) -> (x/y=w3031:dbl)
        "Desired Scan Incr (V)" <- w3031
        n578 = local read "APD Integration Time (s)"() -> (w3024:dbl)
        n579 = Multiply(x=w3031, y=w3011) -> (x*y=w3040:dbl)
        n580 = Divide(x=w3040, y=10.0) -> (x/y=w3030:dbl)
        "Desired incr (int)" <- w3030
        n581 = local read "Update Count (MCL)"() -> (w3036:u32)
        n582 = Round Toward -Infinity(1:w3030) -> (0:w3039:dbl)
        n583 = To Word Integer(number=w3039) -> (16bit integer=w3014:i16)
        "Actual Incr. int (MCL)" <- w3014
        n584 = Multiply(x=w3024, y=40000000.0) -> (x*y=w3037:dbl)
        n585 = Divide(x=w3037, y=w3036) -> (x/y=w3035:dbl)
        n586 = Multiply(x=i16 10, y=w3014) -> (x*y=w3012:i16)
        n587 = Multiply(x="N APD Samp/step", y=w3035) -> (x*y=w3034:dbl)
        "Cycles/step (MCL)" <- w3034
        n588 = Divide(x=w3012, y=w3011) -> (x/y=→"Actual MCL Inc (V)":dbl)
        n589 = Multiply(x="N APD Samp/step", y="Scan steps (MCL)") -> (x*y=w3026:dbl)
        n590 = local read "APD Samples/FIFO Acq."() -> (w3023:dbl)
        n591 = Multiply(x=w3026, y=u64 2) -> (x*y=w3025:dbl)
        "Data points/scan (f+b)" <- w3025
        n592 = Multiply(x=w3025, y=w3016) -> (x*y=w3043:dbl)
        "Data points/scans (MCL)" <- w3043
        n593 = Multiply(x=w3024, y=w3025) -> (x*y=w3017:dbl)
        "Time/f+b scan (s) (MCL)" <- w3017
        n594 = Divide(x=w3043, y=w3023) -> (x/y=→"N sets should be saved (MCL)":dbl)
        n595 = Multiply(x=w3017, y=w3016) -> (x*y=→"Total Time (s)":dbl)
        n596 = Not(x="Fast Scan Dir") -> (.not. x?=w3021:bool)
        n597 = xnode "Read/Write Control"("FPGA VI Reference In"=w3047, "error in"=w3046, "Scan steps (MCL)"="Scan steps (MCL)", "Number of scans (MCL)"=w3016, "Cycles per step (MCL)"=w3034, "Scan freq.  increment (MCL)"=w3014, "1D or 2D Scan?"="2D or 1D Scan", "MCL Scan Axis"=w3021, "Cont. Scan (MCL)"="Continuous MCL Scanning") -> ("error out"=w3045:errorcluster)  [unwired: 1 out]
      }
      event #35 {
        w3184 = 1000.0 ("y")
        n598 = event-data() -> ()  [unwired: 7 out]
        n599 = local read "Save file name"() -> (w3209:path)
        n600 = local write "Read Cal"(FALSE ("Read Cal")) -> ()
        n601 = Strip Path(path=w3209) -> (stripped path=w3208:path)  [unwired: 1 out]
        n602 = Path To String(path=w3208) -> (string=w3207:string)
        n603 = Concatenate Strings(w3207, "\\current.cal" ("string")) -> (w3205:string)
        n604 = String To Path(string=w3205) -> (path=w3204:path)
        n605 = Open/Create/Replace File(file path (use dialog)=w3204, operation (0:open)=T22."open", access (0:read/write)=enum16{"read/write", "read-only", "write-only"}."read-only") -> (refnum out=w3212:refnum<file>, error out=w3198:errorcluster)  [unwired: 1 in, 3 out]
        n606 = Deny Access(4:w3198, 7:w3212) -> (0:w3197:errorcluster, 3:w3203:refnum<file>)  [unwired: 1 out]
        n607 = Read from Binary File(5:0.0, 8:w3197, 9:T21."big-endian, network order" ("byte order (0:big-endian, network order)"), 10:-1 ("count (1)"), 11:w3203) -> (0:w3196:errorcluster, 2:w3194:dbl[], 3:w3199:refnum<file>)  [unwired: 2 out]
        n608 = Array To Cluster(array=w3194) -> (cluster=w3193:T24)
        n609 = Unbundle(w3193) -> ("[0]"=w3192:dbl, "[1]"=w3191:dbl, "[2]"=w3190:dbl, "[3]"=w3189:dbl, "[4]"=w3188:dbl, "[5]"=w3187:dbl)
        n610 = Close File(refnum=w3199, error in=w3196) -> (error out=→"Read cal error":errorcluster)  [unwired: 1 out]
        n611 = Multiply(x=w3187, y=w3184) -> (x*y=w3185:dbl)
        n612 = local write "T2 kappa_x (pN/nm)"(w3189) -> ()
        n613 = local write "T1 kappa_x (pN/nm)"(w3190) -> ()
        n614 = local write "T1 alpha_x (nm/V)"(w3192) -> ()
        n615 = local write "T2 alpha_x (nm/V)"(w3191) -> ()
        n616 = Multiply(x=w3188, y=w3184) -> (x*y=w3186:dbl)
        n617 = local write "T1 offset_x (mV)"(w3186) -> ()
        n618 = local write "T2 offset_x (mV)"(w3185) -> ()
      }
      event #36 {
        n619 = event-data() -> ()  [unwired: 7 out]
        n620 = local write "MCL Scanning"(FALSE ("MCL Scanning")) -> ()
        n621 = xnode "Read/Write Control"("FPGA VI Reference In"=w3217, "error in"=w3216, "Abort scan (MCL)"="Abort MCL Scan") -> ("error out"=w3215:errorcluster)  [unwired: 1 out]
      }
      event #37 {
        n622 = event-data() -> ()  [unwired: 7 out]
        n623 = xnode "Read/Write Control"("FPGA VI Reference In"=w3258, "error in"=w3257, "MCL count"="Update Count (MCL)") -> ("error out"=w3256:errorcluster)  [unwired: 1 out]
      }
      event #38 {
        n624 = event-data() -> ()  [unwired: 7 out]
        n625 = Negate(x="Phase adjust (MCL)") -> (-x=w3303:i16)
        n626 = Select(t=w3303, s="- phase (MCL)", f="Phase adjust (MCL)") -> (s? t:f=w3301:i16)
        n627 = Or(x="- phase (MCL)", y="+ phase (MCL)") -> (x .or. y?=w3296:bool)
        n628 = xnode "Read/Write Control"("FPGA VI Reference In"=w3305, "error in"=w3304, "Phase count adjustment (MCL)"=w3301) -> ("FPGA VI Reference Out"=w3297:T15, "error out"=w3298:errorcluster)
        n629 = xnode "Read/Write Control"("FPGA VI Reference In"=w3297, "error in"=w3298, "+ phase (MCL)"=w3296) -> ("error out"=w3295:errorcluster)  [unwired: 1 out]
      }
      event #39 {
        n630 = event-data() -> ()  [unwired: 7 out]
        n631 = xnode "Read/Write Control"("FPGA VI Reference In"=w3382, "error in"=w3381, "Abort scan"="Abort AOD Scan") -> ("error out"=w3380:errorcluster)  [unwired: 1 out]
      }
      event #40 {
        n632 = event-data() -> ()  [unwired: 7 out]
        n633 = xnode "Read/Write Control"("FPGA VI Reference In"=w3423, "error in"=w3422, "Cont. Scan"="Continuous AOD Scanning") -> ("error out"=w3421:errorcluster)  [unwired: 1 out]
      }
      event #41 {
        n634 = event-data() -> ()  [unwired: 7 out]
        n635 = call "Create new save file.vi"("Insert"="", "Ext"=".dat" ("string"), "Index In"="Index") -> ("Path Out"=→"Save file name":path, "Index Out"=w3461:dbl)
        "Save index" <- w3461
        n636 = local write "Index"(w3461) -> ()
      }
      event #42 {
        w3476 = 10.0 ("y")
        w3475 = 32767.0 ("y")
        n637 = event-data() -> ()  [unwired: 7 out]
        n638 = local read "AO2"() -> (w3474:dbl)
        n639 = local read "AO1"() -> (w3471:dbl)
        n640 = Multiply(x=w3471, y=w3475) -> (x*y=w3470:dbl)
        n641 = Multiply(x=w3474, y=w3475) -> (x*y=w3473:dbl)
        n642 = Divide(x=w3470, y=w3476) -> (x/y=w3469:dbl)
        n643 = Divide(x=w3473, y=w3476) -> (x/y=w3472:dbl)
        n644 = To Word Integer(number=w3469) -> (16bit integer=w3477:i16)
        n645 = To Word Integer(number=w3472) -> (16bit integer=w3478:i16)
        n646 = xnode "Read/Write Control"("FPGA VI Reference In"=w3468, "error in"=w3467, "AO1"=w3477, "AO2"=w3478) -> ("error out"=w3466:errorcluster)  [unwired: 1 out]
      }
      event #43 {
        n647 = event-data() -> ()  [unwired: 7 out]
        n648 = local read "Syringe Pump Serial Port"() -> (w3534:refnum<visa-resource-name>)
        n649 = local read "Pump write delay (ms)"() -> (w3535:dbl)
        n650 = case shown="True" "Inject Pump 1 (DNA)" {
          tunnel: w3535 -> [w3540 w3548]
          tunnel: w3534 -> [w3537 w3547]
          frame #0 {
            n651 = flat-sequence {
              tunnel: w3537 -> [w3541]
              tunnel: [w3541] -> w3538
              tunnel: w3540 -> [_]
              tunnel: [w3544] -> w3539
              tunnel: w3538 -> [w3544]
              tunnel: w3539 -> [w3545]
              frame #0 {
                n652 = call "Write to pump.vi"("string"="enter pump1", "VISA resource name"=w3541) -> ()  [unwired: 1 out]
              }
              frame #1 {
                n653 = Wait (ms)(milliseconds to wait="Pump pause delay (ms)") -> ()  [unwired: 1 out]
              }
              frame #2 {
                n654 = call "Write to pump.vi"("string"="stop", "VISA resource name"=w3545) -> ()  [unwired: 1 out]
              }
            }
          }
          frame #1 {
            n655 = flat-sequence {
              tunnel: w3547 -> [w3557]
              tunnel: w3548 -> [w3552]
              tunnel: w3548 -> [w3559]
              tunnel: w3547 -> [w3560]
              frame #0 {
                n656 = local read "All Pump Parameters"() -> (w3551:T5)
                n657 = Unbundle By Name(w3551) -> ("Pump 1"=w3558:T25)
                n658 = call "Set pump parameters.vi"("Pump write delay (ms)"=w3552, "Volume (uL)"="Top Ch Inject Volume (uL)", "Rate (uL/h)"="Top Ch Inject Rate (ul/h)", "Units"=4.0, "Pump #"=1.0, "Pump Parameters In"=w3558, "VISA resource name"=w3557) -> ("Pump Parameters Out"=w3550:T25)  [unwired: 3 in]
                n659 = Bundle By Name(cluster=w3551, "Pump 1"=w3550) -> (w3549:T5)
                n660 = local write "All Pump Parameters"(w3549) -> ()
              }
              frame #1 {
                n661 = Wait (ms)(milliseconds to wait=w3559) -> ()  [unwired: 1 out]
              }
              frame #2 {
                n662 = call "Write to pump.vi"("string"="start", "VISA resource name"=w3560) -> ()  [unwired: 1 out]
              }
            }
          }
        }
      }
      event #44 {
        n663 = event-data() -> ()  [unwired: 7 out]
        n664 = local read "Pump write delay (ms)"() -> (w3563:dbl)
        n665 = case shown="True" "Inject Pump 3 (D)" {
          tunnel: w3563 -> [w3568 w3576]
          tunnel: "Syringe Pump Serial Port" -> [w3565 w3575]
          frame #0 {
            n666 = flat-sequence {
              tunnel: w3565 -> [w3569]
              tunnel: [w3569] -> w3566
              tunnel: w3568 -> [_]
              tunnel: [w3572] -> w3567
              tunnel: w3566 -> [w3572]
              tunnel: w3567 -> [w3573]
              frame #0 {
                n667 = call "Write to pump.vi"("string"="enter pump3", "VISA resource name"=w3569) -> ()  [unwired: 1 out]
              }
              frame #1 {
                n668 = local read "Pump pause delay (ms)"() -> (w3571:u32)
                n669 = Wait (ms)(milliseconds to wait=w3571) -> ()  [unwired: 1 out]
              }
              frame #2 {
                n670 = call "Write to pump.vi"("string"="stop", "VISA resource name"=w3573) -> ()  [unwired: 1 out]
              }
            }
          }
          frame #1 {
            n671 = flat-sequence {
              tunnel: w3575 -> [w3585]
              tunnel: w3576 -> [w3580]
              tunnel: w3576 -> [w3587]
              tunnel: w3575 -> [w3588]
              frame #0 {
                n672 = local read "All Pump Parameters"() -> (w3579:T5)
                n673 = Unbundle By Name(w3579) -> ("Pump 3"=w3586:T25)
                n674 = call "Set pump parameters.vi"("Pump write delay (ms)"=w3580, "Volume (uL)"="Bottom Ch Inject Volume (uL)", "Rate (uL/h)"="Bottom Ch Inject Rate (ul/h)", "Units"=4.0, "Pump #"=3.0, "Pump Parameters In"=w3586, "VISA resource name"=w3585) -> ("Pump Parameters Out"=w3578:T25)  [unwired: 3 in]
                n675 = Bundle By Name(cluster=w3579, "Pump 3"=w3578) -> (w3577:T5)
                n676 = local write "All Pump Parameters"(w3577) -> ()
              }
              frame #1 {
                n677 = Wait (ms)(milliseconds to wait=w3587) -> ()  [unwired: 1 out]
              }
              frame #2 {
                n678 = call "Write to pump.vi"("string"="start", "VISA resource name"=w3588) -> ()  [unwired: 1 out]
              }
            }
          }
        }
      }
      event #45 {
        n679 = event-data() -> ()  [unwired: 7 out]
        n680 = local read "Pump write delay (ms)"() -> (w3592:dbl)
        n681 = flat-sequence {
          tunnel: w3590 -> [w3605]
          tunnel: w3592 -> [w3601]
          tunnel: "Flush Center Channel" -> [_]
          tunnel: w3592 -> [w3607]
          tunnel: w3590 -> [w3608]
          frame #0 {
            n682 = local read "All Pump Parameters"() -> (w3600:T5)
            n683 = Multiply(x=60.0, y="Flush Center Ch Rate (ul/m)") -> (x*y=w3597:dbl)
            n684 = Unbundle By Name(w3600) -> ("Pump 2"=w3606:T25)
            n685 = call "Set pump parameters.vi"("Pump write delay (ms)"=w3601, "Volume (uL)"="Flush Center Ch Volume (uL)", "Rate (uL/h)"=w3597, "Units"=3.0, "Pump #"=2.0, "Pump Parameters In"=w3606, "VISA resource name"=w3605) -> ("Pump Parameters Out"=w3599:T25)  [unwired: 3 in]
            n686 = Bundle By Name(cluster=w3600, "Pump 2"=w3599) -> (w3598:T5)
            n687 = local write "All Pump Parameters"(w3598) -> ()
            n688 = Add(x="Flush Center Ch Volume (uL)", y="Total Volume\nFlushed (uL)") -> (x+y=w3594:dbl)
            n689 = local write "Total Volume\nFlushed (uL)"(w3594) -> ()
          }
          frame #1 {
            n690 = Wait (ms)(milliseconds to wait=w3607) -> ()  [unwired: 1 out]
          }
          frame #2 {
            n691 = call "Write to pump.vi"("string"="start", "VISA resource name"=w3608) -> ()  [unwired: 1 out]
          }
        }
        n692 = local read "Syringe Pump Serial Port"() -> (w3590:refnum<visa-resource-name>)
      }
      event #46 {
        n693 = event-data() -> ()  [unwired: 7 out]
        n694 = flat-sequence {
          tunnel: w3616 -> [w3622]
          tunnel: w3615 -> [w3621]
          tunnel: [w3619] -> w3613
          tunnel: [w3618] -> w3612
          tunnel: [w3661] -> w3611
          tunnel: w3613 -> [w3661]
          tunnel: [w3660] -> w3610
          tunnel: w3612 -> [w3660]
          tunnel: w3611 -> [w3665]
          tunnel: w3610 -> [w3664]
          tunnel: [w3663] -> w3614
          frame #0 {
            n695 = xnode "Read/Write Control"("FPGA VI Reference In"=w3622, "error in"=w3621, "Green Filter Flipper"=TRUE) -> ("FPGA VI Reference Out"=w3619:T15, "error out"=w3618:errorcluster)
          }
          frame #1 {
            n696 = Wait (ms)(milliseconds to wait=u32 500) -> ()  [unwired: 1 out]
          }
          frame #2 {
            n697 = xnode "Read/Write Control"("FPGA VI Reference In"=w3665, "error in"=w3664, "Green Filter Flipper"=FALSE) -> ("error out"=w3663:errorcluster)  [unwired: 1 out]
          }
        }
      }
    }
    "error out 2" <- w875
    n698 = node-c288() -> ()  [unwired: 2 out]
  }
  n699 = timed-loop "Mouse control: trap position (AOM deflection), set confocal spot from image" {
    tunnel: [w3705] -> w135
    tunnel: w78 -> [w3704]
    timing: w17 -> [_]
    timing-out: [_] -> w16
    stop <- w3705 stop-if-true
    n700 = node-c288() -> ()  [unwired: 2 out]
    n701 = event shown="[0] \"Pane\": Mouse Down" {
      selector: _ -> [_ _]
      dyn-events: _ -> [_ _]
      timeout: _ -> [_ _]
      tunnel: w3704 -> [w3708 _]
      event #0 {
        n702 = event-data() -> ("Time"=w3710:u32, "Coords"=w3709:T7, "Button"=w3711:u16)  [unwired: 6 out]
        n703 = case shown="1" w3711 {
          tunnel: w3710 -> [_ _ w3807]
          tunnel: w3709 -> [_ w3741 w3805]
          tunnel: w3708 -> [_ _ w3803]
          frame #0 {
          }
          frame #1 {
            n704 = property on="APD 1" class="ImageControl"() -> ("Displayed Image Position"=w3740:cluster{"Left":i32, "Top":i32})  [unwired: 2 in, 2 out]
            n705 = property on="Detection Laser X" class="ImageControl"() -> ("Displayed Image Position"=w3737:cluster{"Left":i32, "Top":i32})  [unwired: 2 in, 2 out]
            n706 = property on="Detection Laser Y" class="ImageControl"() -> ("Displayed Image Position"=w3736:cluster{"Left":i32, "Top":i32})  [unwired: 2 in, 2 out]
            n707 = property on="APD 1" class="ImageControl"() -> ("Displayed Image Size"=w3738:cluster{"Width":u32, "Height":u32})  [unwired: 2 in, 2 out]
            n708 = property on="Detection Laser X" class="ImageControl"() -> ("Displayed Image Size"=w3739:cluster{"Width":u32, "Height":u32})  [unwired: 2 in, 2 out]
            n709 = property on="Detection Laser Y" class="ImageControl"() -> ("Displayed Image Size"=w3735:cluster{"Width":u32, "Height":u32})  [unwired: 2 in, 2 out]
            n710 = Unbundle By Name(w3738) -> ("Width"=w3732:u32, "Height"=w3731:u32)
            n711 = Unbundle By Name(w3739) -> ("Width"=w3728:u32, "Height"=w3727:u32)
            n712 = Unbundle By Name(w3735) -> ("Width"=w3724:u32, "Height"=w3723:u32)
            n713 = Unbundle By Name(w3740) -> ("Left"=w3734:i32, "Top"=w3733:i32)
            n714 = Unbundle By Name(w3737) -> ("Left"=w3730:i32, "Top"=w3729:i32)
            n715 = Unbundle By Name(w3736) -> ("Left"=w3726:i32, "Top"=w3725:i32)
            n716 = Bundle("Left"=w3734, "Top"=w3733, "Width"=w3732, "Height"=w3731) -> (w3722:T26)  [unwired: 1 in]
            n717 = Bundle("Left"=w3730, "Top"=w3729, "Width"=w3728, "Height"=w3727) -> (w3721:T26)  [unwired: 1 in]
            n718 = Bundle("Left"=w3726, "Top"=w3725, "Width"=w3724, "Height"=w3723) -> (w3720:T26)  [unwired: 1 in]
            n719 = Build Cluster Array(w3722, w3721, w3720) -> (w3719:T27)
            n720 = for {
              tunnel: w3741 -> [w3752]
              tunnel: w3719 -> [w3753] mode=indexing
              shift-right: [w3750] -> w3717
              shift-left: TRUE -> [w3751]
              shift-right: [w3749] -> w3715
              shift-left: _ -> [w3745]
              shift-right: [w3748] -> w3714
              shift-left: _ -> [w3744]
              shift-right: [w3747] -> w3713
              shift-left: _ -> [w3743]
              shift-right: [w3746] -> w3712
              shift-left: _ -> [w3742]
              n721 = case shown="True" w3751 {
                selector: w3751 -> [w3758 _]
                tunnel: w3753 -> [_ w3767]
                tunnel: w3752 -> [_ w3765]
                tunnel: [w3758 w3763] -> w3750
                tunnel: [w3757 w3762] -> w3749
                tunnel: [w3756 w3761] -> w3748
                tunnel: [w3755 w3760] -> w3747
                tunnel: [w3754 w3759] -> w3746
                tunnel: w3745 -> [w3757 _]
                tunnel: w3744 -> [w3756 _]
                tunnel: w3743 -> [w3755 _]
                tunnel: w3742 -> [w3754 _]
                frame #0 {
                }
                frame #1 {
                  n722 = Unbundle(w3767) -> (w3766:T26)
                  n723 = call "isclickinwindow.vi"("Image Param"=w3766, "Point32"=w3765) -> ("4 Y"=w3759:i32, "3 Height"=w3760:i32, "2 X"=w3761:i32, "1 Width"=w3762:i32, "In image?"=w3764:bool)  [unwired: 1 in]
                  n724 = Not(x=w3764) -> (.not. x?=w3763:bool)
                }
              }
            }
            n725 = Not(x=w3717) -> (.not. x?=w3716:bool)
            n726 = case shown="True" w3716 {
              tunnel: w3714 -> [_ w3780]
              tunnel: w3712 -> [_ w3779]
              tunnel: w3715 -> [_ w3778]
              tunnel: w3713 -> [_ w3777]
              frame #0 {
              }
              frame #1 {
                w3773 = FALSE ("Get Point")
                n727 = local read "Scan lines (y)"() -> (w3782:u64)
                n728 = local read "Actual MCL Inc (V)"() -> (w3774:dbl)
                n729 = local read "Scan steps (MCL)"() -> (w3781:u64)
                n730 = Divide "Y Pix/step"(x=w3777, y=w3782) -> (x/y=w3789:dbl)
                n731 = Divide "Y V/pix"(x=w3774, y=w3789) -> (x/y=w3788:dbl)
                n732 = Divide "Y half step offset"(x=w3774, y=2.0) -> (x/y=w3790:dbl)
                n733 = Divide "X pix/step"(x=w3778, y=w3781) -> (x/y=w3787:dbl)
                n734 = Negate(x=w3790) -> (-x=w3791:dbl)
                n735 = local read "Initial Y"() -> (w3797:dbl)
                n736 = Multiply(x=w3779, y=w3788) -> (x*y=w3798:dbl)
                n737 = Divide "X half step offset"(x=w3774, y=2.0) -> (x/y=w3784:dbl)
                n738 = Divide "X V/pix"(x=w3774, y=w3787) -> (x/y=w3786:dbl)
                n739 = Multiply(x=w3774, y=w3781) -> (x*y=w3793:dbl)
                n740 = Compound Arithmetic op=ADD(w3791, w3798, w3797) -> (w3775:dbl)
                "Pointer Y (V)" <- w3775
                n741 = Multiply(x=w3786, y=w3780) -> (x*y=w3795:dbl)
                n742 = Negate(x=w3784) -> (-x=w3783:dbl)
                n743 = local read "Initial X"() -> (w3796:dbl)
                n744 = Negate(x=w3795) -> (-x=w3794:dbl)
                n745 = Compound Arithmetic op=ADD(w3783, w3793, w3796, w3794) -> (w3776:dbl)
                "Pointer X (V)" <- w3776
                n746 = Or(x="Set X Only", y="Set Confocal Spot (X-Y)") -> (x .or. y?=w3769:bool)
                n747 = Or(x="Set Confocal Spot (X-Y)", y="Set Y Only") -> (x .or. y?=w3768:bool)
                n748 = case shown="True" w3769 {
                  tunnel: w3776 -> [_ w3799]
                  frame #0 {
                  }
                  frame #1 {
                    n749 = property on="AO2" class="Slide (strict)"("Val(Sgnl)"=w3799) -> ()  [unwired: 2 in, 2 out]
                  }
                }
                n750 = case shown="True" w3768 {
                  tunnel: w3775 -> [_ w3800]
                  frame #0 {
                  }
                  frame #1 {
                    n751 = property on="AO1" class="Slide (strict)"("Val(Sgnl)"=w3800) -> ()  [unwired: 2 in, 2 out]
                  }
                }
                n752 = local write "Set Confocal Spot (X-Y)"(w3773) -> ()
                n753 = local write "Set X Only"(w3773) -> ()
                n754 = local write "Set Y Only"(w3773) -> ()
              }
            }
          }
          frame #2 {
            n755 = local read "BD 2 Frequency 1 (MHz)"() -> (w3801:dbl)
            n756 = local read "BD 1 Frequency 1 (MHz)"() -> (w3802:dbl)
            n757 = local write "Manipulating Trap"(TRUE ("Manipulating Trap")) -> ()
            n758 = local write "Coords"(T7 {"Horizontal"=0, "Vertical"=0} ("Coords")) -> ()
            n759 = while {
              tunnel: w3807 -> [w3812]
              tunnel: w3805 -> [w3811]
              tunnel: w3803 -> [w3810]
              tunnel: w3802 -> [w3809]
              tunnel: w3801 -> [w3808]
              stop <- w3813 stop-if-true
              n760 = event shown="[0] \"Pane\": Mouse Move" {
                selector: _ -> [_ _]
                dyn-events: _ -> [_ _]
                timeout: _ -> [_ _]
                tunnel: ["Force Manip Abort" w3877] -> w3813
                tunnel: w3812 -> [w3820 _]
                tunnel: w3811 -> [w3818 _]
                tunnel: w3810 -> [w3817 _]
                tunnel: w3809 -> [w3816 _]
                tunnel: w3808 -> [w3815 _]
                event #0 {
                  n761 = event-data() -> ("Time"=w3821:u32, "Coords"=w3822:T7)  [unwired: 3 out]
                  n762 = Less?(x=w3821, y=w3820) -> (x < y?=w3819:bool)
                  n763 = case "Makes sure old motion events prior to mouse click aren't used" shown="False" w3819 {
                    tunnel: w3822 -> [w3864 _]
                    tunnel: w3818 -> [w3865 _]
                    tunnel: w3817 -> [w3842 _]
                    tunnel: w3816 -> [w3838 _]
                    tunnel: w3815 -> [w3837 _]
                    frame #0 {
                      n764 = Subtract(x=w3864, y=w3865) -> (x-y=w3863:T7)
                      "Coords" <- w3863
                      n765 = local read "Y RF Frequency Limits (MHz)"() -> (w3823:T12)
                      n766 = To Double Precision Float(number=w3863) -> (double precision float=w3862:cluster{"Horizontal":dbl, "Vertical":dbl})
                      n767 = Multiply(x=cluster{"Horizontal":dbl, "Vertical":dbl} {"Horizontal"=-1.0, "Vertical"=1.0}, y="Manipulation Scaling") -> (x*y=w3858:cluster{"Horizontal":dbl, "Vertical":dbl})
                      n768 = local read "X RF Frequency Limits (MHz)"() -> (w3824:T12)
                      n769 = Multiply(x=w3862, y=w3858) -> (x*y=w3860:cluster{"Horizontal":dbl, "Vertical":dbl})
                      n770 = Unbundle By Name(w3860) -> ("Horizontal"=w3855:dbl, "Vertical"=w3859:dbl)
                      n771 = Unbundle By Name(w3823) -> ("Maximum"=w3826:dbl, "Minimum"=w3825:dbl)
                      n772 = Boolean To (0,1)(Boolean="Manip. X?") -> (0, 1=w3853:i16)
                      n773 = Boolean To (0,1)(Boolean="Manip. Y?") -> (0, 1=w3850:i16)
                      n774 = Multiply(x=w3859, y=w3850) -> (x*y=w3852:dbl)
                      n775 = Multiply(x=w3853, y=w3855) -> (x*y=w3856:dbl)
                      n776 = local read "BD 1 Frequency 2 (MHz)"() -> (w3840:dbl)
                      n777 = Unbundle By Name(w3824) -> ("Maximum"=w3828:dbl, "Minimum"=w3827:dbl)
                      n778 = local read "BD 2 Frequency 2 (MHz)"() -> (w3839:dbl)
                      n779 = Add(x=w3837, y=w3852) -> (x+y=w3830:dbl)
                      n780 = Add(x=w3838, y=w3856) -> (x+y=w3832:dbl)
                      n781 = In Range and Coerce(upper limit=w3828, x=w3832, lower limit=w3827) -> (coerced(x)=w3831:dbl)  [unwired: 1 out]
                      n782 = In Range and Coerce(upper limit=w3826, x=w3830, lower limit=w3825) -> (coerced(x)=w3829:dbl)  [unwired: 1 out]
                      n783 = Subtract(x=w3831, y=w3840) -> (x-y=w3849:dbl)
                      n784 = Subtract(x=w3829, y=w3839) -> (x-y=w3848:dbl)
                      n785 = Square(x=w3849) -> (x^2=w3847:dbl)
                      n786 = Square(x=w3848) -> (x^2=w3846:dbl)
                      n787 = Add(x=w3847, y=w3846) -> (x+y=w3845:dbl)
                      n788 = Square Root(x=w3845) -> (sqrt(x)=w3841:dbl)
                      n789 = In Range and Coerce(upper limit="Limit Max (MHz)", x=w3841, lower limit="Limit Min (MHz)") -> (In Range?=w3834:bool)  [unwired: 1 out]
                      n790 = Not(x="Limits Enable") -> (.not. x?=w3833:bool)
                      n791 = Or(x=w3834, y=w3833) -> (x .or. y?=w3835:bool)
                      n792 = case shown="True" w3835 {
                        tunnel: w3842 -> [_ w3875]
                        tunnel: w3841 -> [_ w3866]
                        tunnel: w3831 -> [_ w3873]
                        tunnel: w3840 -> [_ w3872]
                        tunnel: w3829 -> [_ w3871]
                        tunnel: w3839 -> [_ w3870]
                        tunnel: w3824 -> [_ w3868]
                        tunnel: w3823 -> [_ w3867]
                        frame #0 {
                        }
                        frame #1 {
                          n793 = local read "BD 1 Frequency 3 (MHz)"() -> (w3874:dbl)
                          n794 = local read "BD 2 Frequency 3 (MHz)"() -> (w3869:dbl)
                          n795 = local write "Trap Delta (MHz)"(w3866) -> ()
                          n796 = property on="Initial delta (MHz)" class="DigNum (strict)"("Val(Sgnl)"=w3866) -> ()  [unwired: 2 in, 2 out]
                          n797 = call "set RF board frequency - interlace.vi"("Board 2 Frequency Limits"=w3867, "Board 1 Frequency Limits"=w3868, "FPGA VI Reference In"=w3875, "Board 2 Frequency 3 (MHz)"=w3869, "Board 1 Frequency 3 (MHz)"=w3874, "Board 2 Frequency 2 (MHz)"=w3870, "Board 2 Frequency 1 (MHz)"=w3871, "Board 1 Frequency 2 (MHz)"=w3872, "Board 1 Frequency 1  (MHz)"=w3873) -> ()  [unwired: 1 in, 2 out]
                          n798 = local write "BD 2 Frequency 1 (MHz)"(w3871) -> ()
                          n799 = local write "BD 1 Frequency 1 (MHz)"(w3873) -> ()
                        }
                      }
                    }
                    frame #1 {
                    }
                  }
                }
                event #1 {
                  n800 = event-data() -> ("Button"=w3876:u16)  [unwired: 8 out]
                  n801 = case shown="3" w3876 {
                    tunnel: [FALSE TRUE] -> w3877
                    frame #0 {
                    }
                    frame #1 {
                      n802 = local write "Manipulating Trap"(FALSE ("Manipulating Trap")) -> ()
                    }
                  }
                }
              }
            }
          }
        }
      }
      event #1 {
        n803 = event-data() -> ()  [unwired: 6 out]
      }
    }
    n804 = local read "Stop All"() -> (w3705:bool)
    n805 = node-c288() -> ()  [unwired: 2 out]
  }
  n806 = timed-loop "Oscillate AOD (debugging)" {
    tunnel: w78 -> [w3882]
    tunnel: [w3881] -> w18
    timing: w11 -> [_]
    timing-out: [_] -> w10
    stop <- w3881 stop-if-true
    n807 = node-c288() -> ()  [unwired: 2 out]
    n808 = event shown="[1] \"Fl. Triggered...\": Value Change" {
      selector: _ -> [_ _ _]
      dyn-events: _ -> [_ _ _]
      timeout: _ -> [_ _ _]
      tunnel: w3882 -> [w3889 _ _]
      tunnel: [FALSE ("Stop All") _ w4122] -> w3881
      event #0 {
        n809 = event-data() -> ()  [unwired: 6 out]
        n810 = local read "Oscillate Set 1"() -> (w3888:bool)
        n811 = Or(x=w3888, y="Fish for Tether") -> (x .or. y?=w3886:bool)
        n812 = case shown="True" w3886 {
          tunnel: w3889 -> [_ w3891]
          tunnel: "Fish for Tether" -> [_ w3890]
          frame #0 {
          }
          frame #1 {
            n813 = case shown="True" w3890 {
              frame #0 {
              }
              frame #1 {
                n814 = local write "Scan axis 2"(TRUE) -> ()
                n815 = local write "Tether"(FALSE ("Tether")) -> ()
              }
            }
            n816 = node-c288() -> (w3893:T18)  [unwired: 4 out]
            n817 = timed-loop "Oscillate AOD" {
              timing: w3893 -> [_]
              timing-out: [_] -> w3892
              tunnel: w3891 -> [w3903]
              tunnel: w3890 -> [w3902]
              i -> [w3905]
              stop <- w3901 stop-if-true
              n818 = node-c288() -> (w3904:i64)  [unwired: 1 out]
              n819 = flat-sequence {
                tunnel: w3905 -> [w3932]
                tunnel: w3904 -> [w3931]
                tunnel: w3903 -> [w3910]
                tunnel: w3902 -> [w3913]
                tunnel: [w3913] -> w3900
                tunnel: [w3912] -> w3899
                tunnel: [w3909] -> w3898
                tunnel: [w3906] -> w3896
                tunnel: w3900 -> [w3968]
                tunnel: w3899 -> [w3966]
                tunnel: w3898 -> [w3965]
                tunnel: [w3964] -> w3897
                tunnel: w3896 -> [w3963]
                tunnel: [w4002] -> w3901
                tunnel: w3897 -> [w4001]
                frame #0 {
                  n820 = Divide(x=w3931, y=i64 1000) -> (x/y=w3926:dbl)
                  n821 = Multiply(x=w3926, y=w3932) -> (x*y=w3928:dbl)
                  n822 = local read "BD 1 Frequency 2 (MHz)"() -> (w3911:dbl)
                  n823 = Multiply(x="Osc. freq. (Hz)", y=6.283185307179586) -> (x*y=w3929:dbl)
                  n824 = Multiply(x=w3929, y=w3928) -> (x*y=w3908:dbl)
                  n825 = local read "BD 1 Frequency 1 (MHz)"() -> (w3916:dbl)
                  n826 = case shown="True" w3913 {
                    tunnel: w3908 -> [w3938 w3943]
                    tunnel: w3916 -> [_ w3954]
                    tunnel: w3911 -> [_ w3955]
                    tunnel: [w3935 w3949] -> w3914
                    tunnel: [FALSE w3946] -> w3909
                    tunnel: [0.0 w3939] -> w3906
                    frame #0 {
                      n827 = Sine(x=w3938) -> (sin(x)=w3936:dbl)
                      n828 = Multiply(x=w3936, y="Osc. amp. (MHz)") -> (x*y=w3935:dbl)
                    }
                    frame #1 {
                      n829 = Cosine(x=w3943) -> (cos(x)=w3958:dbl)
                      n830 = Subtract(x=w3955, y=w3954) -> (x-y=w3953:dbl)
                      n831 = Decrement(x=w3958) -> (x-1=w3957:dbl)
                      n832 = Subtract(x=w3953, y="Closest Delta (MHz)") -> (x-y=w3950:dbl)
                      n833 = Divide(x=w3957, y=-2.0) -> (x/y=w3951:dbl)
                      n834 = Multiply(x=w3951, y=w3950) -> (x*y=w3949:dbl)
                      n835 = local read "Vec Mean of T1 T2"() -> (w3945:dbl[])
                      n836 = Greater?(x=w3945, y="Stop F (pN)") -> (0:w3947:bool[])
                      n837 = Or Array Elements(Boolean array=w3947) -> (logical OR=w3946:bool)
                      n838 = Divide(x=w3943, y=6.283185307179586) -> (x/y=w3942:dbl)
                      n839 = Round Toward +Infinity(x=w3942) -> (ceil(x): smallest int >= x=w3939:dbl)
                      "Attempts" <- w3939
                      n840 = Greater?(x=w3939, y="Attempt Limit") -> (0:w3941:bool)
                      n841 = case shown="True" w3941 {
                        frame #0 {
                        }
                        frame #1 {
                          n842 = call <vilib>:"Beep.vi"() -> ()  [unwired: 3 in, 9 out]
                          n843 = local write "Fish for Tether"(FALSE ("Fish for Tether")) -> ()
                          n844 = local read "Messages"() -> (w3960:string)
                          n845 = call "Update messages.vi"("Message to add"="Tether fishing timeout." ("Messages"), "Old message string"=w3960) -> ("New message string"=→"Messages":string)
                        }
                      }
                    }
                  }
                  n846 = local read "BD 2 Frequency 1 (MHz)"() -> (w3915:dbl)
                  n847 = Select(t=w3916, s="Scan axis 2", f=w3915) -> (s? t:f=w3919:dbl)
                  n848 = Add(x=w3914, y=w3919) -> (x+y=w3912:dbl)
                  n849 = Select(t=w3912, s="Scan axis 2", f=w3916) -> (s? t:f=w3922:dbl)
                  n850 = Select(t=w3915, s="Scan axis 2", f=w3912) -> (s? t:f=w3921:dbl)
                  n851 = local read "Y RF Frequency Limits (MHz)"() -> (w3917:T12)
                  n852 = local read "X RF Frequency Limits (MHz)"() -> (w3918:T12)
                  n853 = local read "BD 1 Frequency 3 (MHz)"() -> (w3925:dbl)
                  n854 = local read "BD 2 Frequency 2 (MHz)"() -> (w3924:dbl)
                  n855 = local read "BD 2 Frequency 3 (MHz)"() -> (w3923:dbl)
                  n856 = call "set RF board frequency - interlace.vi"("Board 2 Frequency Limits"=w3917, "Board 1 Frequency Limits"=w3918, "FPGA VI Reference In"=w3910, "Board 2 Frequency 3 (MHz)"=w3923, "Board 1 Frequency 3 (MHz)"=w3925, "Board 2 Frequency 2 (MHz)"=w3924, "Board 2 Frequency 1 (MHz)"=w3921, "Board 1 Frequency 2 (MHz)"=w3911, "Board 1 Frequency 1  (MHz)"=w3922) -> ()  [unwired: 1 in, 2 out]
                }
                frame #1 {
                  n857 = And(x=w3968, y=w3965) -> (x .and. y?=w3967:bool)
                  n858 = case "Only if were fishing and now formed tether" shown="True" w3967 {
                    tunnel: w3966 -> [w3970 w3983]
                    tunnel: [w3969 w3982] -> w3964
                    tunnel: w3963 -> [_ w3978]
                    frame #0 {
                      n859 = local read "Fish for Tether"() -> (w3969:bool)
                      n860 = case shown="False" w3969 {
                        tunnel: w3970 -> [w3971 _]
                        frame #0 {
                          n861 = property on="BD 1 Frequency 1 (MHz)" class="DigNum (strict)"("Val(Sgnl)"=w3971) -> ()  [unwired: 2 in, 2 out]
                        }
                        frame #1 {
                        }
                      }
                    }
                    frame #1 {
                      w3982 = FALSE ("Fish for Tether")
                      n862 = call <vilib>:"Beep.vi"() -> ()  [unwired: 3 in, 9 out]
                      n863 = Number To Decimal String(number=w3978, width (-)=i16 1) -> (decimal integer string=w3976:string)
                      n864 = case shown="\"2\", \"3\", \"4\"" "Then..." {
                        selector: "Then..." -> [_ w3986]
                        tunnel: w3983 -> [w3985 _]
                        frame #0 {
                          n865 = property on="BD 1 Frequency 1 (MHz)" class="DigNum (strict)"("Val(Sgnl)"=w3985) -> ()  [unwired: 2 in, 2 out]
                        }
                        frame #1 {
                          n866 = flat-sequence {
                            tunnel: w3986 -> [w3988]
                            frame #0 {
                              n867 = property on="Trap Delta (MHz)" class="DigNum (strict)"("Val(Sgnl)"="Move to Delta (MHz)") -> ()  [unwired: 2 in, 2 out]
                            }
                            frame #1 {
                              n868 = case shown="\"3\", \"4\"" w3988 {
                                selector: w3988 -> [w3991 _]
                                frame #0 {
                                n869 = flat-sequence {
                                tunnel: w3991 -> [w3992]
                                tunnel: [w3992] -> w3989
                                tunnel: [w3994] -> w3990
                                tunnel: w3989 -> [w3994]
                                tunnel: w3990 -> [w3998]
                                frame #0 {
                                n870 = property on="Green Laser ON/Interlacing" class="Bool (strict)"("Val(Sgnl)"=TRUE ("Value (Signaling)")) -> ()  [unwired: 2 in, 2 out]
                                }
                                frame #1 {
                                n871 = Multiply(x="Wait Before Save (s)", y=u32 1000 ("x")) -> (x*y=w3996:u32)
                                n872 = Wait (ms)(milliseconds to wait=w3996) -> ()  [unwired: 1 out]
                                }
                                frame #2 {
                                n873 = case shown="\"4\"" w3998 {
                                frame #0 {
                                }
                                frame #1 {
                                n874 = property on="Fl. Triggered..." class="Bool (strict)"("Val(Sgnl)"=TRUE ("Value (Signaling)")) -> ()  [unwired: 2 in, 2 out]
                                }
                                }
                                n875 = property on="Start Saving" class="Bool (strict)"("Value"=TRUE ("Start Saving")) -> ()  [unwired: 2 in, 2 out]
                                }
                                }
                                }
                                frame #1 {
                                }
                              }
                            }
                          }
                        }
                      }
                      n876 = Concatenate Strings("Formed tether in ", w3976, " attempt(s)." ("string")) -> (w3973:string)
                      n877 = local read "Messages"() -> (w3980:string)
                      n878 = local write "Fish for Tether"(w3982) -> ()
                      n879 = call "Update messages.vi"("Message to add"=w3973, "Old message string"=w3980) -> ("New message string"=w3979:string)
                      n880 = local write "Messages"(w3979) -> ()
                      n881 = Get Date/Time In Seconds() -> (seconds since 1Jan1904=→"Time tether formed":timestamp)
                      "Tether" <- "Tether Alarm?"
                    }
                  }
                }
                frame #2 {
                  n882 = local read "Oscillate Set 1"() -> (w4006:bool)
                  n883 = Or(x=w4006, y=w4001) -> (x .or. y?=w4003:bool)
                  n884 = local read "Stop All"() -> (w4004:bool)
                  n885 = Not(x=w4003) -> (.not. x?=w4005:bool)
                  n886 = Compound Arithmetic op=OR(w4004, w4005) -> (w4002:bool)
                }
              }
              n887 = node-c288() -> ()  [unwired: 2 out]
            }
            n888 = node-c288(w3892) -> ()  [unwired: 1 out]
          }
        }
      }
      event #1 {
        n889 = event-data() -> ()  [unwired: 7 out]
        n890 = case shown="True" "Fl. Triggered..." {
          frame #0 {
          }
          frame #1 {
            n891 = node-c288() -> (w4016:T18)  [unwired: 4 out]
            n892 = timed-loop {
              timing: w4016 -> [_]
              timing-out: [_] -> w4015
              tunnel: "Action" -> [w4020]
              shift-right: [w4017] -> _
              shift-left: u8 255 -> [w4019]
              stop <- w4021 stop-if-true
              n893 = node-c288() -> ()  [unwired: 2 out]
              n894 = flat-sequence {
                tunnel: w4020 -> [w4029]
                tunnel: w4019 -> [w4025]
                tunnel: [w4024] -> w4018
                tunnel: [w4113] -> w4021
                tunnel: w4018 -> [w4112]
                tunnel: [w4112] -> w4017
                frame #0 {
                  n895 = local read "Delta Fl. (Hz)"() -> (w4026:dbl)
                  n896 = Multiply(x="Fl. Delta Thresh. (kHz)", y=1000.0) -> (x*y=w4028:dbl)
                  n897 = Greater?(x=w4026, y=w4028) -> (0:w4030:bool)
                  n898 = Or(x=w4030, y="Force Yank") -> (x .or. y?=w4023:bool)
                  n899 = case shown="True" w4023 {
                    tunnel: w4029 -> [_ w4040]
                    tunnel: w4025 -> [w4032 w4036]
                    tunnel: [w4032 w4033] -> w4024
                    frame #0 {
                    }
                    frame #1 {
                      n900 = flat-sequence {
                        tunnel: w4037 -> [w4046]
                        tunnel: [w4046] -> w4041
                        tunnel: w4040 -> [w4045]
                        tunnel: [w4045] -> w4039
                        tunnel: [w4044] -> w4038
                        tunnel: w4036 -> [w4043]
                        tunnel: [w4042] -> w4035
                        tunnel: w4041 -> [w4071]
                        tunnel: w4039 -> [w4070]
                        tunnel: w4038 -> [w4069]
                        tunnel: w4035 -> [w4068]
                        tunnel: [w4068] -> w4034
                        tunnel: w4034 -> [w4110]
                        tunnel: [w4110] -> w4033
                        frame #0 {
                          n901 = call <vilib>:"Beep.vi"() -> ()  [unwired: 3 in, 9 out]
                          n902 = local write "Waiting"(FALSE ("Waiting")) -> ()
                          n903 = Increment(x=w4043) -> (x+1=w4042:u8)
                          n904 = case shown="\"Yank\"" w4045 {
                            tunnel: w4042 -> [_ _ w4052]
                            frame #0 {
                              n905 = property on="Confocal Image" class="Bool (strict)"("Val(Sgnl)"=TRUE ("Value (Signaling)")) -> ()  [unwired: 2 in, 2 out]
                            }
                            frame #1 {
                            }
                            frame #2 {
                              n906 = flat-sequence {
                                tunnel: w4052 -> [w4055]
                                tunnel: [w4054] -> w4051
                                tunnel: ["N Array El"] -> w4050
                                tunnel: w4051 -> [w4065]
                                tunnel: w4050 -> [w4061]
                                frame #0 {
                                n907 = Multiply(x="Yank Delay (s)", y=1000.0) -> (x*y=w4058:dbl)
                                n908 = Quotient & Remainder(x=w4055, y="N Array El") -> (x-y*floor(x/y)=w4054:u8)  [unwired: 1 out]
                                n909 = Wait (ms)(milliseconds to wait=w4058) -> ()  [unwired: 1 out]
                                }
                                frame #1 {
                                n910 = Random Number (0-1)() -> (number: 0 to 1=w4062:dbl)
                                n911 = Multiply(x=w4061, y=w4062) -> (x*y=w4060:dbl)
                                n912 = Round Toward -Infinity(1:w4060) -> (0:w4059:dbl)
                                n913 = Select(t=w4059, s="Random Choice", f=w4065) -> (s? t:f=w4063:dbl)
                                n914 = Index Array(array="Yank to Delta Array (MHz)", index=w4063) -> (element=w4066:dbl)
                                n915 = property on="Trap Delta (MHz)" class="DigNum (strict)"("Val(Sgnl)"=w4066) -> ()  [unwired: 2 in, 2 out]
                                }
                              }
                            }
                          }
                          n916 = local read "Time (s)"() -> (w4044:dbl)
                          "Fl. High" <- TRUE ("Yanking")
                        }
                        frame #1 {
                          n917 = node-c288() -> (w4073:T18)  [unwired: 4 out]
                          n918 = timed-loop {
                            timing: w4073 -> [_]
                            timing-out: [_] -> w4072
                            tunnel: w4071 -> [w4086]
                            tunnel: w4070 -> [w4084]
                            tunnel: w4069 -> [w4083]
                            stop <- w4085 stop-if-true
                            n919 = node-c288() -> ()  [unwired: 2 out]
                            n920 = local read "Fl. Delta Thresh. (kHz)"() -> (w4078:dbl)
                            n921 = local read "Fl. Triggered..."() -> (w4087:bool)
                            n922 = local read "Delta Fl. (Hz)"() -> (w4077:dbl)
                            n923 = local read "Stop All"() -> (w4081:bool)
                            n924 = Not(x=w4087) -> (.not. x?=w4082:bool)
                            n925 = Multiply(x=w4078, y=1000.0) -> (x*y=w4076:dbl)
                            n926 = Negate(x=w4076) -> (-x=w4075:dbl)
                            n927 = Less?(x=w4077, y=w4075) -> (x < y?=w4080:bool)
                            n928 = Compound Arithmetic op=OR(w4080, w4081, w4082, "Force Reset") -> (w4085:bool)
                            n929 = case shown="True" w4085 {
                              tunnel: w4086 -> [_ w4098]
                              tunnel: w4084 -> [_ w4097]
                              tunnel: w4083 -> [_ w4095]
                              frame #0 {
                              }
                              frame #1 {
                                n930 = case shown="\"Yank\"" w4097 {
                                tunnel: w4098 -> [_ w4099]
                                frame #0 {
                                }
                                frame #1 {
                                n931 = flat-sequence {
                                tunnel: [w4104] -> w4100
                                tunnel: w4099 -> [w4104]
                                tunnel: w4100 -> [w4105]
                                frame #0 {
                                n932 = local read "Yank Delay (s)"() -> (w4103:dbl)
                                n933 = Multiply(x=w4103, y=1000.0) -> (x*y=w4101:dbl)
                                n934 = Wait (ms)(milliseconds to wait=w4101) -> ()  [unwired: 1 out]
                                }
                                frame #1 {
                                n935 = property on="Trap Delta (MHz)" class="DigNum (strict)"("Val(Sgnl)"=w4105) -> ()  [unwired: 2 in, 2 out]
                                }
                                }
                                }
                                }
                                n936 = local read "Time (s)"() -> (w4096:dbl)
                                n937 = Subtract(x=w4096, y=w4095) -> (x-y=w4092:dbl)
                                "Duration (s)" <- w4092
                                n938 = Number To Decimal String(number=w4092, width (-)=i16 0) -> (decimal integer string=w4090:string)
                                n939 = Concatenate Strings(w4090, " s fluorescence event." ("string")) -> (w4088:string)
                                n940 = local read "Messages"() -> (w4094:string)
                                n941 = call "Update messages.vi"("Message to add"=w4088, "Old message string"=w4094) -> ("New message string"=w4093:string)
                                n942 = call <vilib>:"Beep.vi"() -> ()  [unwired: 3 in, 9 out]
                                n943 = local write "Messages"(w4093) -> ()
                              }
                            }
                            n944 = node-c288() -> ()  [unwired: 2 out]
                          }
                          n945 = node-c288(w4072) -> ()  [unwired: 1 out]
                        }
                        frame #2 {
                          n946 = local write "Fl. High"(FALSE ("Yanking")) -> ()
                        }
                      }
                      n947 = local read "Trap Delta (MHz)"() -> (w4037:dbl)
                    }
                  }
                }
                frame #1 {
                  n948 = local read "Stop All"() -> (w4116:bool)
                  n949 = local read "Fl. Triggered..."() -> (w4114:bool)
                  n950 = Not(x=w4114) -> (.not. x?=w4115:bool)
                  n951 = Or(x=w4115, y=w4116) -> (x .or. y?=w4113:bool)
                  n952 = Not(x=w4113) -> (.not. x?=→"Waiting":bool)
                }
              }
              n953 = node-c288() -> ()  [unwired: 2 out]
            }
            n954 = node-c288(w4015) -> ()  [unwired: 1 out]
          }
        }
      }
      event #2 {
        n955 = event-data() -> ()  [unwired: 7 out]
        n956 = local read "Stop All"() -> (w4122:bool)
      }
    }
    n957 = node-c288() -> ()  [unwired: 2 out]
  }
  n958 = timed-loop "Stage Control and Stage + Action Control" {
    shift-right: [w4137] -> w59
    shift-left: w61 -> [w4154]
    shift-right: [w4136] -> w58
    shift-left: w60 -> [w4153]
    tunnel: w57 -> [w4138]
    timing: w15 -> [_]
    timing-out: [_] -> w14
    shift-right: ["Dump Beads"] -> _
    shift-left: FALSE ("Dump Beads") -> [w4130]
    stop <- w4155 stop-if-true
    (unwired) T12 {"Minimum"=0.0, "Maximum"=0.0, "Increment"=0.0}  # Y Limits
    (unwired) T12 {"Minimum"=0.0, "Maximum"=0.0, "Increment"=0.0}  # X Limits
    n959 = node-c288() -> ()  [unwired: 2 out]
    n960 = local read "Stop All"() -> (w4155:bool)
    n961 = call "Read Stage Position.vi"("error in"=w4153, "VISA resource name in"=w4154) -> ("Current Position"=w4139:cluster{dbl, dbl, dbl}, "error out"=w4146:errorcluster, "VISA resource name out"=w4147:refnum<visa-resource-name>)  [unwired: 1 out]
    "Current Stage  Position" <- w4139
    n962 = Or(x="Move to Position 3", y="Data Acq. Spot") -> (x .or. y?=w4132:bool)
    n963 = Or(x="Lower Cap.", y=w4130) -> (x .or. y?=w4129:bool)
    n964 = Or(x="Move to Position 1", y="Upper Cap.") -> (x .or. y?=w4135:bool)
    n965 = Compound Arithmetic op=OR(w4129, "Move to Position 2") -> (w4134:bool)
    n966 = Or(x="Lower Ch. Cap.", y="Move to Position 5") -> (x .or. y?=w4124:bool)
    n967 = Or(x="Dump Beads", y="Move to Position 4") -> (x .or. y?=w4131:bool)
    n968 = Build Array(w4135, w4134, w4132, w4131, w4124) -> (w4145:bool[])
    n969 = Or Array Elements(Boolean array=w4145) -> (logical OR=w4148:bool)
    n970 = case shown="True" w4148 {
      tunnel: w4147 -> [w4200 w4209]
      tunnel: w4146 -> [w4199 w4208]
      tunnel: [w4200 w4212] -> w4144
      tunnel: [w4199 w4211] -> w4143
      tunnel: w4145 -> [_ w4210]
      tunnel: "Dump Beads" -> [_ w4205]
      tunnel: w4129 -> [_ w4204]
      tunnel: "Upper Cap." -> [_ w4203]
      tunnel: "Data Acq. Spot" -> [_ w4202]
      tunnel: "Dump Beads" -> [_ w4201]
      frame #0 {
      }
      frame #1 {
        n971 = flat-sequence {
          tunnel: w4210 -> [w4221]
          tunnel: w4209 -> [w4216]
          tunnel: w4208 -> [w4215]
          tunnel: [w4224] -> w4207
          tunnel: [w4223] -> w4206
          tunnel: w4201 -> [w4213]
          tunnel: [w4232] -> w4211
          tunnel: [w4233] -> w4212
          tunnel: w4207 -> [w4233]
          tunnel: w4206 -> [w4232]
          tunnel: w4205 -> [w4230]
          tunnel: w4204 -> [w4229]
          tunnel: w4203 -> [w4228]
          tunnel: w4202 -> [w4227]
          frame #0 {
            n972 = local read "Saved Stage Positions"() -> (w4220:T4)
            n973 = Boolean Array To Number(Boolean array=w4221) -> (number=w4222:u32)
            n974 = case shown="True" w4213 {
              frame #0 {
              }
              frame #1 {
                w4226 = FALSE ("Fl. Triggered...")
                n975 = local read "Saving..."() -> (w4225:bool)
                n976 = property on="Green Laser ON/Interlacing" class="Bool (strict)"("Val(Sgnl)"=w4226) -> ()  [unwired: 2 in, 2 out]
                n977 = local write "Fl. Triggered..."(w4226) -> ()
                n978 = local write "Stop Saving"(w4225) -> ()
              }
            }
            n979 = Logarithm Base 2(1:w4222) -> (0:w4218:dbl)
            n980 = Cluster To Array(cluster=w4220) -> (array=w4219:cluster{dbl, dbl, dbl}[])
            n981 = Index Array(array=w4219, index=w4218) -> (element=w4217:cluster{dbl, dbl, dbl})
            n982 = call "Set Stage Position.vi"("Position"=w4217, "error in"=w4215, "VISA resource name in"=w4216) -> ("error out"=w4223:errorcluster, "VISA resource name out"=w4224:refnum<visa-resource-name>)  [unwired: 1 out]
            "Stage Moving" <- TRUE ("Stage Moving")
          }
          frame #1 {
            n983 = local write "Stage Moving"(FALSE ("Stage Moving")) -> ()
            n984 = case shown="True" w4230 {
              frame #0 {
              }
              frame #1 {
                w4253 = FALSE ("Value (Signaling)")
                n985 = property on="Trap 1 (ON/OFF)" class="Bool (strict)"("Val(Sgnl)"=w4253) -> ()  [unwired: 2 in, 2 out]
                n986 = property on="Trap 2 (ON/OFF)" class="Bool (strict)"("Val(Sgnl)"=w4253) -> ()  [unwired: 2 in, 2 out]
              }
            }
            n987 = call <vilib>:"Beep.vi"() -> ()  [unwired: 3 in, 9 out]
            n988 = case shown="True" w4228 {
              selector: w4228 -> [_ w4251]
              frame #0 {
              }
              frame #1 {
                n989 = property on="Trap 2 (ON/OFF)" class="Bool (strict)"("Val(Sgnl)"=w4251) -> ()  [unwired: 2 in, 2 out]
              }
            }
            n990 = case shown="True" w4227 {
              frame #0 {
              }
              frame #1 {
                n991 = flat-sequence {
                  frame #0 {
                    n992 = property on="Save Calibration" class="Bool (strict)"("Val(Sgnl)"=TRUE ("Value (Signaling)")) -> ()  [unwired: 2 in, 2 out]
                  }
                  frame #1 {
                    n993 = Wait (ms)(milliseconds to wait=u32 4000) -> ()  [unwired: 1 out]
                  }
                  frame #2 {
                    n994 = while {
                      stop <- w4236 stop-if-true
                      n995 = local read "Saving..."() -> (w4237:bool)
                      n996 = Wait (ms)(milliseconds to wait=u32 500) -> ()  [unwired: 1 out]
                      n997 = Not(x=w4237) -> (.not. x?=w4236:bool)
                    }
                  }
                  frame #3 {
                    n998 = case shown="True" "With\nOffset" {
                      frame #0 {
                        n999 = Multiply(x="Cal read wait (s)", y=u32 1000 ("milliseconds to wait")) -> (x*y=w4241:u32)
                        n1000 = Wait (ms)(milliseconds to wait=w4241) -> ()  [unwired: 1 out]
                      }
                      frame #1 {
                        n1001 = flat-sequence {
                          frame #0 {
                            n1002 = property on="Trap Raster Scan" class="Bool (strict)"("Val(Sgnl)"=TRUE ("Value (Signaling)")) -> ()  [unwired: 2 in, 2 out]
                          }
                          frame #1 {
                            n1003 = Wait (ms)(milliseconds to wait=u32 2000) -> ()  [unwired: 1 out]
                          }
                          frame #2 {
                            n1004 = while {
                              stop <- w4246 stop-if-true
                              n1005 = local read "Raster Scanning..."() -> (w4247:bool)
                              n1006 = Wait (ms)(milliseconds to wait=u32 500) -> ()  [unwired: 1 out]
                              n1007 = Not(x=w4247) -> (.not. x?=w4246:bool)
                            }
                          }
                        }
                      }
                    }
                  }
                  frame #4 {
                    n1008 = property on="Read Cal" class="Bool (strict)"("Val(Sgnl)"=TRUE ("Value (Signaling)")) -> ()  [unwired: 2 in, 2 out]
                  }
                  frame #5 {
                    n1009 = Wait (ms)(milliseconds to wait=u32 500) -> ()  [unwired: 1 out]
                  }
                  frame #6 {
                    n1010 = property on="Fish for Tether" class="Bool (strict)"("Val(Sgnl)"=TRUE ("Value (Signaling)")) -> ()  [unwired: 2 in, 2 out]
                  }
                }
              }
            }
            n1011 = case shown="True" w4229 {
              selector: w4229 -> [_ w4252]
              frame #0 {
              }
              frame #1 {
                n1012 = property on="Trap 1 (ON/OFF)" class="Bool (strict)"("Val(Sgnl)"=w4252) -> ()  [unwired: 2 in, 2 out]
              }
            }
          }
        }
      }
    }
    n1013 = Or(x="+z", y="-z") -> (x .or. y?=w4142:bool)
    n1014 = case shown="True" w4142 {
      tunnel: w4144 -> [w4159 w4163]
      tunnel: w4143 -> [w4158 w4162]
      tunnel: [w4159 w4166] -> w4137
      tunnel: [w4158 w4165] -> w4136
      tunnel: "+z" -> [_ w4169]
      tunnel: "-z" -> [_ w4168]
      tunnel: w4139 -> [_ w4167]
      tunnel: w4138 -> [_ w4164]
      frame #0 {
      }
      frame #1 {
        n1015 = flat-sequence {
          tunnel: w4169 -> [w4195]
          tunnel: w4168 -> [w4194]
          tunnel: w4167 -> [w4190]
          tunnel: w4164 -> [w4175]
          tunnel: w4163 -> [w4172]
          tunnel: w4162 -> [w4171]
          tunnel: [w4182] -> w4161
          tunnel: [w4181] -> w4160
          tunnel: [w4197] -> w4165
          tunnel: [w4198] -> w4166
          tunnel: w4161 -> [w4198]
          tunnel: w4160 -> [w4197]
          frame #0 {
            n1016 = Boolean To (0,1)(Boolean=w4195) -> (0, 1=w4193:i16)
            n1017 = Boolean To (0,1)(Boolean=w4194) -> (0, 1=w4192:i16)
            n1018 = Unbundle(w4190) -> (w4189:dbl, w4188:dbl, w4184:dbl)
            n1019 = Divide(x="z nudge increment (um)", y=1000.0) -> (x/y=w4178:dbl)
            n1020 = Multiply(x=w4193, y=w4178) -> (x*y=w4186:dbl)
            n1021 = Multiply(x=w4192, y=w4178) -> (x*y=w4191:dbl)
            n1022 = Negate(x=w4191) -> (-x=w4187:dbl)
            n1023 = Add(x=w4186, y=w4187) -> (x+y=w4185:dbl)
            n1024 = local write "Stage Moving"(TRUE ("Stage Moving")) -> ()
            n1025 = Add(x=w4185, y=w4184) -> (x+y=w4177:dbl)
            n1026 = Unbundle(w4175) -> ("Minimum"=w4174:dbl, "Maximum"=w4173:dbl)  [unwired: 1 out]
            n1027 = In Range and Coerce(upper limit=w4173, x=w4177, lower limit=w4174) -> (coerced(x)=w4176:dbl)  [unwired: 1 out]
            n1028 = Bundle(cluster=w4190, w4189, w4188, w4176) -> (w4183:cluster{dbl, dbl, dbl})
            n1029 = call "Set Stage Position.vi"("Position"=w4183, "error in"=w4171, "VISA resource name in"=w4172) -> ("error out"=w4181:errorcluster, "VISA resource name out"=w4182:refnum<visa-resource-name>)  [unwired: 1 out]
          }
          frame #1 {
            n1030 = local write "Stage Moving"(FALSE ("Stage Moving")) -> ()
          }
        }
      }
    }
    n1031 = node-c288() -> ()  [unwired: 2 out]
  }
  n1032 = flat-sequence "Video" {
    tunnel: [w4262] -> w190
    tunnel: w190 -> [w4298]
    tunnel: w188 -> [w4296]
    frame #0 {
      n1033 = while {
        stop <- w4255 continue-if-true
        n1034 = call "Close Video Capture.vi"() -> ("error code OUT"=w4257:i32)
        n1035 = Equal?(x=w4257, y=0) -> (x = y?=w4255:bool)
      }
      n1036 = local write "Stop All"(FALSE ("Stop All")) -> ()
    }
    frame #1 {
      n1037 = call "DMR_Init.vi"() -> ()  [unwired: 3 out]
    }
    frame #2 {
      # "Setting the destination format to Mono8 makes sure that the image can be displayed in the intensity plot."
      n1038 = call "DMR_GetDevice.vi"("search string IN"="DE019116701") -> ("device handle OUT"=w4280:i32)  [unwired: 4 in, 2 out]
      n1039 = call "DMR_OpenDevice.vi"("device handle IN"=w4280) -> ("driver handle OUT"=w4263:i32)  [unwired: 4 out]
      n1040 = call "DMR_FindList.vi"("flags IN"=u32 0 ("flags"), "list name IN"="" ("String"), "list type IN"=T28."camera descriptions", "driver handle IN"=w4263) -> ("list handle OUT"=w4266:i32)  [unwired: 2 out]
      n1041 = call "DMR_FindList.vi"("flags IN"=u32 0 ("flags"), "list name IN"="Base", "list type IN"=T28."setting", "driver handle IN"=w4263) -> ("list handle OUT"=w4264:i32)  [unwired: 2 out]
      n1042 = call "OBJ_GetHandle.vi"("object name IN"="VideoStandard", "list handle IN"=w4266) -> ("object handle OUT"=w4260:i32)  [unwired: 3 out]
      n1043 = call "OBJ_GetHandle.vi"("object name IN"="PixelFormat", "list handle IN"=w4264) -> ("object handle OUT"=w4274:i32)  [unwired: 3 out]
      n1044 = call "OBJ_SetS.vi"("value index IN"=0, "value IN"="NTSC M", "object handle IN"=w4260) -> ()  [unwired: 2 out]
      n1045 = call "OBJ_SetS.vi"("value index IN"=0, "value IN"="Mono8" ("value"), "object handle IN"=w4274) -> ()  [unwired: 2 out]
      n1046 = call "OBJ_GetHandle.vi"("object name IN"="VideoChannel", "list handle IN"=w4264) -> ("object handle OUT"=w4270:i32)  [unwired: 3 out]
      n1047 = while {
        tunnel: [w4285] -> w4262
        tunnel: w4263 -> [w4282]
        stop <- w4283 continue-if-true
        n1048 = call "DMR_ImageRequestSingle.vi"("request control IN"=0, "driver handle IN"=w4282) -> ("error code OUT"=w4284:i32, "driver handle OUT"=w4285:i32)  [unwired: 2 out]
        n1049 = Equal To 0?(x=w4284) -> (x = 0?=w4283:bool)
      }
      n1050 = call "OBJ_SetI.vi"("value index IN"=0, "value IN"=3 ("Video channel"), "object handle IN"=w4270) -> ()  [unwired: 2 out]
    }
    frame #3 {
      w4293 = T13 0 items=["Grayscale (U8)", "Grayscale (I16)", "Grayscale (SGL)", "Complex (CSG)", "RGB (U32)", "HSL (U32)", "RGB (U64)"] ("Image Type")
      n1051 = call "IMAQ Create"("Image Name"="untitled", "Image Type"=w4293) -> ("New Image"=w4294:T2)  [unwired: 2 in, 2 out]
      n1052 = node-c288() -> (w4292:T18)  [unwired: 4 out]
      n1053 = Initialize Array(u32 0 ("Window Number (0...15)"), 480 ("dimension size"), 640 ("dimension size")) -> (w4287:u32[][])
      n1054 = timed-loop {
        tunnel: w4298 -> [w4316]
        tunnel: [w4315] -> w4297
        tunnel: w4296 -> [w4314]
        tunnel: w4294 -> [w4313]
        timing: w4292 -> [_]
        timing-out: [_] -> w4291
        tunnel: w4287 -> [w4299]
        stop <- w4302 stop-if-true
        # "This block performs the \nactual image capture."
        n1055 = node-c288() -> ()  [unwired: 2 out]
        n1056 = local read "Stop All"() -> (w4303:bool)
        n1057 = Reciprocal(x="Video Capture Rate (Hz)") -> (1/x=w4305:dbl)
        n1058 = Or(x=FALSE, y=w4303) -> (x .or. y?=w4302:bool)
        n1059 = Multiply(x=w4305, y=1000.0) -> (x*y=w4300:dbl)
        n1060 = call "DMR_ImageRequestWaitFor.vi"("queue number IN"=0, "timeout(ms) IN"=500, "driver handle IN"=w4316) -> ("error code OUT"=w4320:i32, "request number OUT"=w4317:i32, "driver handle OUT"=w4318:i32)
        n1061 = feedback #1(T29 refnum ("Avi Refnum")) -> (w4307:T29)
        n1062 = case shown="True" "New Video File" {
          tunnel: [T29 refnum ("Avi Refnum") w4337] -> w4309
          tunnel: [FALSE TRUE] -> w4310
          tunnel: w4307 -> [_ w4333]
          frame #0 {
          }
          frame #1 {
            n1063 = call "Create new save file.vi"("Ext"=".avi" ("string"), "Index In"="Video Index") -> ("Path Out"=w4329:path, "Index Out"=w4330:dbl)  [unwired: 1 in]
            "Path Out" <- w4329
            n1064 = Not Equal?(x=w4333, y=T29 refnum ("Avi Refnum")) -> (x != y?=w4334:bool)
            n1065 = Increment(x=w4330) -> (x+1=w4339:dbl)
            n1066 = case shown="True" w4334 {
              tunnel: w4333 -> [_ w4340]
              frame #0 {
              }
              frame #1 {
                n1067 = call "IMAQ AVI Close"("Avi Refnum"=w4340) -> ()  [unwired: 1 in, 10 out]
              }
            }
            n1068 = call "IMAQ AVI Create"("Frames Per Second"=u32 30, "AVI Path"=w4329) -> ("Avi Refnum"=w4337:T29)  [unwired: 5 in, 4 out]
            n1069 = local write "Video Index"(w4339) -> ()
          }
        }
        n1070 = Equal To 0?(x=w4320) -> (x = 0?=w4319:bool)
        n1071 = Select(t=w4309, s=w4310, f=w4307) -> (s? t:f=w4308:T29)
        n1072 = case shown="True" w4319 {
          tunnel: w4318 -> [w4341 w4379]
          tunnel: w4317 -> [_ w4378]
          tunnel: [w4341 w4375] -> w4315
          tunnel: w4314 -> [_ w4365]
          tunnel: w4313 -> [_ w4358]
          tunnel: w4299 -> [_ w4362]
          tunnel: w4308 -> [_ w4360]
          frame #0 {
          }
          frame #1 {
            w4369 = u32 0 ("X-offset IN")
            n1073 = call "DMR_GetImageRequestBufferData.vi"("driver handle IN"=w4379, "request number IN"=w4378) -> ("width OUT"=w4368:i32, "height OUT"=w4367:i32, "driver handle OUT"=w4374:i32, "request number OUT"=w4373:i32, "bytes per pixel OUT"=w4370:i32)  [unwired: 13 out]
            n1074 = call "DMR_GetImageRequestBufferImageData.vi"("driver handle IN"=w4374, "request number IN"=w4373, "bytes per pixel IN"=w4370, "X-offset IN"=w4369, "Y-offset IN"=w4369, "height IN"=w4367, "width IN"=w4368) -> ("driver handle OUT"=w4372:u32, "request number OUT"=w4371:u32, "image OUT"=w4363:u32[][])  [unwired: 10 out]
            n1075 = call "DMR_ImageRequestUnlock.vi"("request number IN"=w4371, "driver handle IN"=w4372) -> ("driver handle OUT"=w4377:i32)  [unwired: 1 in, 2 out]
            n1076 = case shown="True" "Averaging" {
              tunnel: w4363 -> [w4408 w4413]
              tunnel: [w4408 w4412] -> w4359
              tunnel: w4362 -> [_ w4410]
              frame #0 {
              }
              frame #1 {
                (unwired) 1
                w4418 = 1
                n1077 = feedback #2(w4410) -> (w4409:u32[][])
                n1078 = Add(x=w4413, y=w4409) -> (x+y=w4414:u32[][])
                n1079 = Select(t=w4410, s="Reset Averaging", f=w4414) -> (s? t:f=w4416:u32[][])
                n1080 = feedback #3(w4418) -> (w4411:i32)
                n1081 = Divide(x=w4414, y=w4411) -> (x/y=w4415:dbl[][])
                n1082 = Increment(x=w4411) -> (x+1=w4419:i32)
                n1083 = To Unsigned Long Integer(number=w4415) -> (unsigned 32bit integer=w4412:u32[][])
                n1084 = Select(t=w4418, s="Reset Averaging", f=w4419) -> (s? t:f=w4417:i32)
              }
            }
            "Image" <- w4359
            n1085 = case shown="True" "Capture and Save Image" {
              tunnel: w4359 -> [_ w4430]
              tunnel: w4365 -> [_ w4429]
              frame #0 {
              }
              frame #1 {
                n1086 = To Unsigned Byte Integer(number=w4430) -> (unsigned 8bit integer=w4426:u8[][])
                n1087 = call <vilib>:"Flatten Pixmap.vi"("colors"=w4429, "8-bit pixmap"=w4426) -> ("image data"=w4427:T30)  [unwired: 4 in, 5 out]
                n1088 = call "Create new save file.vi"("Insert"="video_frame_" ("string"), "Ext"=".bmp" ("string"), "Index In"="Image Index") -> ("Path Out"=w4422:path, "Index Out"=w4428:dbl)
                n1089 = call <vilib>:"Write BMP File.vi"("image data"=w4427, "path to BMP file"=w4422) -> ()  [unwired: 1 in, 9 out]
                n1090 = Increment(x=w4428) -> (x+1=w4421:dbl)
                n1091 = local write "Image Index"(w4421) -> ()
              }
            }
            n1092 = case shown="True" "Capture Video" {
              tunnel: w4360 -> [_ w4407]
              tunnel: w4359 -> [_ w4405]
              tunnel: w4358 -> [_ w4404]
              frame #0 {
              }
              frame #1 {
                n1093 = To Unsigned Byte Integer(number=w4405) -> (unsigned 8bit integer=w4406:u8[][])
                n1094 = call "IMAQ ArrayToImage"("Image Pixels (U8)"=w4406, "Image"=w4404) -> ("Image Out"=w4403:T2)  [unwired: 4 in, 5 out]
                n1095 = call "IMAQ AVI Write Frame"("Image"=w4403, "Avi Refnum"=w4407) -> ()  [unwired: 2 in, 8 out]
              }
            }
            n1096 = call "DMR_ImageRequestSingle.vi"("request control IN"=0, "driver handle IN"=w4377) -> ("driver handle OUT"=w4375:i32)  [unwired: 3 out]
            n1097 = To Double Precision Float(number=w4359) -> (double precision float=w4354:dbl[][])
            n1098 = Initialize Array(u8 1, 480 ("dimension size"), 640 ("dimension size")) -> (w4353:u8[][])
            n1099 = Multiply(x=w4353, y="Intensity Upper") -> (x*y=w4352:u8[][])
            n1100 = Multiply(x=w4353, y="Intensity Lower") -> (x*y=w4351:u8[][])
            n1101 = In Range and Coerce(upper limit=w4352, x=w4354, lower limit=w4351) -> (coerced(x)=w4350:dbl[][])  [unwired: 1 out]
            n1102 = Subtract(x=w4350, y="Intensity Lower") -> (x-y=w4346:dbl[][])
            n1103 = Subtract(x="Intensity Upper", y="Intensity Lower") -> (x-y=w4345:u8)
            n1104 = Divide(x=w4346, y=w4345) -> (x/y=w4347:dbl[][])
            n1105 = Multiply(x=u8 255, y=w4347) -> (x*y=w4343:dbl[][])
            n1106 = To Unsigned Byte Integer(number=w4343) -> (unsigned 8bit integer=w4342:u8[][])
            n1107 = disable-structure shown="Disabled" {
              disable-tunnel: w4358 -> [w4383 _]
              disable-tunnel: w4342 -> [w4380 _]
              frame #0 {
                n1108 = call "IMAQ ArrayToImage"("Image Pixels (U8)"=w4380, "Image"=w4383) -> ("Image Out"=w4381:T2)  [unwired: 4 in, 5 out]
                n1109 = First Call?() -> (First Call?: T/F=w4382:bool)
                n1110 = case shown="True" w4382 {
                  tunnel: w4381 -> [w4384 w4395]
                  frame #0 {
                    n1111 = flat-sequence {
                      tunnel: w4384 -> [w4390]
                      frame #0 {
                        w4387 = FALSE ("Get/Set Status? (Set)")
                        w4386 = 0 ("Window Number (0...15)")
                        n1112 = call "IMAQ WindSize"("Get/Set Status? (Set)"=w4387, "Window Number"=w4386) -> ("Width & Height out"=→"Window Size":cluster{"Width":i32, "Height":i32})  [unwired: 4 in, 2 out]
                        n1113 = call "IMAQ WindMove"("Window Number (0...15)"=w4386, "Get/Set Status? (Set)"=w4387) -> ("Coordinates (screen)"=→"Window Position":cluster{"X Position":i32, "Y Position":i32})  [unwired: 3 in, 1 out]
                        n1114 = call "IMAQ WindDraw"("Resize to Image Size? (Y)"=FALSE, "Window Number (0...15)"=w4386, "Image"=w4390) -> ()  [unwired: 7 in, 2 out]
                      }
                      frame #1 {
                        n1115 = call "IMAQ WindZoom 2"("Center Point"="Center Point", "Zoom to Fit? (False)"=FALSE, "Zoom Factor"="Zoom Factor") -> ()  [unwired: 5 in, 4 out]
                      }
                    }
                  }
                  frame #1 {
                    n1116 = flat-sequence {
                      tunnel: w4395 -> [w4398]
                      tunnel: [w4396] -> w4394
                      tunnel: w4394 -> [w4400]
                      frame #0 {
                        w4397 = TRUE ("Resize to Image Size? (Y)")
                        w4396 = 0 ("Window Number (0...15)")
                        n1117 = call "IMAQ WindNonTearing"("Window Number"=w4396, "NonTearing? (True)"=w4397) -> ()  [unwired: 8 in, 2 out]
                        n1118 = call "IMAQ WindDraw"("Resize to Image Size? (Y)"=w4397, "Window Number (0...15)"=w4396, "Image"=w4398) -> ()  [unwired: 7 in, 2 out]
                      }
                      frame #1 {
                        n1119 = call "IMAQ WindSize"("Scrollbars? (N)"=FALSE, "Width & Height"="Initial Window Size", "Window Number"=w4400) -> ()  [unwired: 3 in, 3 out]
                        n1120 = call "IMAQ WindMove"("Window Number (0...15)"=w4400, "Coordinates (screen)"="Initial Window Position") -> ()  [unwired: 3 in, 2 out]
                      }
                    }
                  }
                }
              }
              frame #1 {
              }
            }
          }
        }
        n1121 = node-c288(w4300) -> ()  [unwired: 1 out]
      }
      n1122 = node-c288(w4291) -> ()  [unwired: 1 out]
      n1123 = call "DMR_CloseDevice.vi"("driver handle IN"=w4297) -> ()  [unwired: 1 in, 4 out]
    }
    frame #4 {
      n1124 = call "DMR_Close.vi"() -> ()  [unwired: 1 out]
    }
  }
  n1125 = node-c288(i64 1 ("Period")) -> (w128:T18)  [unwired: 3 out]
  n1126 = timed-loop "Acquire Data" {
    tunnel: w75 -> [w4610]
    tunnel: w74 -> [w4609]
    tunnel: [w4647] -> w231
    tunnel: [w4641] -> w229
    timing: w128 -> [_]
    timing-out: [_] -> w127
    tunnel: w6 -> [w4442]
    tunnel: w2 -> [w4440]
    tunnel: w1 -> [w4439]
    stop <- "Stop All" stop-if-true
    w4492 = "NI_ChannelName" ("name")
    n1127 = node-c288() -> ()  [unwired: 2 out]
    n1128 = case "Reset data stream" shown="True" "Reset" {
      tunnel: w4610 -> [w6834 w6841]
      tunnel: w4609 -> [w6833 w6840]
      tunnel: [w6834 w6836] -> w4605
      tunnel: [w6833 w6835] -> w4604
      frame #0 {
      }
      frame #1 {
        w6839 = TRUE ("AI to FIFO")
        w6846 = FALSE ("AI to FIFO")
        n1129 = local write "Overflow (data lost)"(FALSE ("Overflow (data lost)")) -> ()
        n1130 = xnode "Read/Write Control"("FPGA VI Reference In"=w6841, "error in"=w6840, "AI to FIFO"=w6846, "APD to FIFO"=w6846) -> ("FPGA VI Reference Out"=w6844:T15, "error out"=w6845:errorcluster)
        n1131 = xnode "Invoke Method"("FPGA VI Reference In"=w6844, "error in"=w6845) -> ("FPGA VI Reference Out"=w6842:T15, "error out"=w6843:errorcluster)
        n1132 = xnode "Invoke Method"("FPGA VI Reference In"=w6842, "error in"=w6843) -> ("FPGA VI Reference Out"=w6838:T15, "error out"=w6837:errorcluster)
        n1133 = xnode "Read/Write Control"("FPGA VI Reference In"=w6838, "error in"=w6837, "AI to FIFO"=w6839, "APD to FIFO"=w6839) -> ("FPGA VI Reference Out"=w6836:T15, "error out"=w6835:errorcluster)
      }
    }
    n1134 = Or(x="Start AOD Scan", y="Trap Raster Scan") -> (x .or. y?=w4552:bool)
    n1135 = And(x="Save scans", y=w4552) -> (x .and. y?=w4601:bool)
    n1136 = case "Start AOM raster scan" shown="True" w4552 {
      tunnel: w4605 -> [w6072 w6082]
      tunnel: w4604 -> [w6071 w6081]
      tunnel: [w6072 w6075] -> w4603
      tunnel: [w6071 w6074] -> w4602
      frame #0 {
      }
      frame #1 {
        n1137 = case shown="True" "Restart DMA? (AOD)" {
          tunnel: [w6448 w6449] -> w6076
          tunnel: [w6447 w6450] -> w6077
          tunnel: w6082 -> [w6448 w6456]
          tunnel: w6081 -> [w6447 w6455]
          frame #0 {
          }
          frame #1 {
            w6452 = FALSE ("AI to FIFO")
            n1138 = xnode "Read/Write Control"("FPGA VI Reference In"=w6456, "error in"=w6455, "AI to FIFO"=w6452, "APD to FIFO"=w6452) -> ("FPGA VI Reference Out"=w6454:T15, "error out"=w6453:errorcluster)
            n1139 = xnode "Invoke Method"("FPGA VI Reference In"=w6454, "error in"=w6453) -> ("FPGA VI Reference Out"=w6458:T15, "error out"=w6457:errorcluster)
            n1140 = xnode "Invoke Method"("FPGA VI Reference In"=w6458, "error in"=w6457) -> ("FPGA VI Reference Out"=w6449:T15, "error out"=w6450:errorcluster)
            n1141 = local write "Overflow (data lost)"(FALSE ("Overflow (data lost)")) -> ()
          }
        }
        n1142 = case shown="True" "Move MCL Also?" {
          tunnel: w6077 -> [w6085 w6191]
          tunnel: w6076 -> [w6086 w6192]
          tunnel: [w6084 w6195] -> w6075
          tunnel: [w6083 w6194] -> w6074
          frame #0 {
            w6087 = TRUE ("AI to FIFO")
            n1143 = xnode "Read/Write Control"("FPGA VI Reference In"=w6086, "error in"=w6085, "AI to FIFO"=w6087, "APD to FIFO"=w6087, "Start scan"=w6087) -> ("FPGA VI Reference Out"=w6084:T15, "error out"=w6083:errorcluster)
          }
          frame #1 {
            w6188 = FALSE ("1D or 2D Scan?")
            w6193 = TRUE ("AI to FIFO")
            # "Count for MCL loop"
            # "N total cycles"
            # "N steps"
            # "V_int"
            n1144 = local read "Scan Range (nm)"() -> (w6170:dbl)
            n1145 = local read "Number of F/B Scans (AOD)"() -> (w6187:u16)
            n1146 = Sign(1:w6170) -> (0:w6169:dbl)
            n1147 = Compound Arithmetic op=MULTIPLY(w6170, "MCL Step Position Ratio", "MCL/AOM Scale Tweak") -> (w6174:dbl)
            n1148 = Negate(x=w6169) -> (-x=w6166:dbl)
            n1149 = Multiply(x=w6166, y="MCL Step Increment (V_int)") -> (x*y=w6168:dbl)
            n1150 = Divide(x=w6174, y="MCL X Cal (nm/V)") -> (x/y=w6180:dbl)
            n1151 = Multiply(x=32767.0 ("y"), y=w6180) -> (x*y=w6186:dbl)
            n1152 = local read "Total Counts (ticks)"() -> (w6171:u32)
            n1153 = local read "Cycles/step (AOD)"() -> (w6182:u64)
            n1154 = local read "Scan steps (AOD)"() -> (w6183:u64)
            n1155 = Divide(x=w6186, y=10.0) -> (x/y=w6179:dbl)
            n1156 = Divide(x=w6179, y="MCL Step Increment (V_int)") -> (x/y=w6177:dbl)
            n1157 = Absolute Value(x=w6177) -> (abs(x)=w6165:dbl)
            n1158 = Compound Arithmetic op=MULTIPLY(w6183, w6182, w6171) -> (w6178:u64)
            n1159 = local write "wait to reset values"(w6193) -> ()
            n1160 = local write "MCL Scanning"(w6193) -> ()
            n1161 = Divide(x=w6178, y=w6165) -> (x/y=w6175:dbl)
            "MCL Count" <- w6175
            n1162 = xnode "Read/Write Control"("FPGA VI Reference In"=w6192, "error in"=w6191, "Scan steps (MCL)"=w6165, "Number of scans (MCL)"=w6187, "Cycles per step (MCL)"=u64 1, "Scan freq.  increment (MCL)"=w6168, "1D or 2D Scan?"=w6188, "MCL Scan Axis"=w6188, "Cont. Scan (MCL)"=w6188, "MCL count"=w6175) -> ("FPGA VI Reference Out"=w6190:T15, "error out"=w6189:errorcluster)
            n1163 = xnode "Read/Write Control"("FPGA VI Reference In"=w6190, "error in"=w6189, "AI to FIFO"=w6193, "APD to FIFO"=w6193, "Start scan"=w6193, "Start scan (MCL)"=w6193) -> ("FPGA VI Reference Out"=w6195:T15, "error out"=w6194:errorcluster)
          }
        }
        n1164 = local write "Trap Raster Scan"(FALSE ("Trap Raster Scan")) -> ()
        "Raster Scanning..." <- TRUE ("Scanning...")
      }
    }
    n1165 = Compound Arithmetic op=OR("Start MCL Scan", "Confocal Image", "Confocal Linescan") -> (w4550:bool)
    n1166 = And(x="Save Data (MCL)", y=w4550) -> (x .and. y?=w4600:bool)
    n1167 = case "Start MCL raster scan" shown="True" w4550 {
      tunnel: w4603 -> [w5256 w5271]
      tunnel: w4602 -> [w5255 w5270]
      tunnel: [w5256 w5266] -> w4487
      tunnel: [w5255 w5265] -> w4486
      tunnel: [FALSE w5264] -> w4586
      tunnel: "Start MCL Scan" -> [_ w5259]
      tunnel: "Confocal Image" -> [_ w5258]
      tunnel: "Confocal Linescan" -> [_ _]
      frame #0 {
      }
      frame #1 {
        w5264 = TRUE
        n1168 = case shown="True" "Restart DMA? (MCL)" {
          tunnel: [w5508 w5511] -> w5269
          tunnel: [w5507 w5510] -> w5268
          tunnel: w5271 -> [w5508 w5516]
          tunnel: w5270 -> [w5507 w5515]
          frame #0 {
          }
          frame #1 {
            w5512 = FALSE ("AI to FIFO")
            n1169 = xnode "Read/Write Control"("FPGA VI Reference In"=w5516, "error in"=w5515, "AI to FIFO"=w5512, "APD to FIFO"=w5512) -> ("FPGA VI Reference Out"=w5514:T15, "error out"=w5513:errorcluster)
            n1170 = xnode "Invoke Method"("FPGA VI Reference In"=w5514, "error in"=w5513) -> ("FPGA VI Reference Out"=w5518:T15, "error out"=w5517:errorcluster)
            n1171 = xnode "Invoke Method"("FPGA VI Reference In"=w5518, "error in"=w5517) -> ("FPGA VI Reference Out"=w5511:T15, "error out"=w5510:errorcluster)
            n1172 = local write "Overflow (data lost)"(FALSE ("Overflow (data lost)")) -> ()
          }
        }
        n1173 = case shown="False" w5259 {
          selector: w5259 -> [_ w5275]
          tunnel: w5258 -> [w5274 _]
          tunnel: [w5274 w5275] -> w5257
          frame #0 {
            n1174 = property on="2D or 1D Scan" class="Bool (strict)"("Val(Sgnl)"=w5274) -> ()  [unwired: 2 in, 2 out]
            n1175 = property on="Confocal Image" class="Bool (strict)"("Value"=FALSE ("Start Confocal Map")) -> ()  [unwired: 2 in, 2 out]
          }
          frame #1 {
          }
        }
        n1176 = local write "MCL Scanning"(w5264) -> ()
        n1177 = local read "AO1"() -> (w5261:dbl)
        n1178 = local read "AO2"() -> (w5260:dbl)
        n1179 = case shown="True" "Center Scan" {
          tunnel: w5269 -> [w5282 w5391]
          tunnel: w5268 -> [w5281 w5390]
          tunnel: [w5280 w5389] -> w5266
          tunnel: [w5279 w5388] -> w5265
          tunnel: [w5277 w5375] -> w5263
          tunnel: [w5276 w5374] -> w5262
          tunnel: w5261 -> [w5277 w5380]
          tunnel: w5260 -> [w5276 w5383]
          tunnel: w5257 -> [_ _]
          frame #0 {
            w5278 = TRUE ("AI to FIFO")
            n1180 = xnode "Read/Write Control"("FPGA VI Reference In"=w5282, "error in"=w5281, "AI to FIFO"=w5278, "APD to FIFO"=w5278, "Start scan (MCL)"=w5278) -> ("FPGA VI Reference Out"=w5280:T15, "error out"=w5279:errorcluster)
          }
          frame #1 {
            w5387 = TRUE ("AI to FIFO")
            n1181 = local read "Scan steps (MCL)"() -> (w5366:u64)
            n1182 = local read "Scan lines (y)"() -> (w5362:u64)
            n1183 = local read "Fast Scan Dir"() -> (w5373:bool)
            n1184 = local read "Actual MCL Inc (V)"() -> (w5363:dbl)
            n1185 = Decrement(x=w5362) -> (x-1=w5361:u64)
            n1186 = Decrement(x=w5366) -> (x-1=w5365:u64)
            n1187 = Multiply(x=w5363, y=w5361) -> (x*y=w5360:dbl)
            n1188 = Divide(x=w5360, y=2.0) -> (x/y=w5370:dbl)
            n1189 = Multiply(x=w5363, y=w5365) -> (x*y=w5364:dbl)
            n1190 = Divide(x=w5364, y=2.0) -> (x/y=w5369:dbl)
            n1191 = Select(t=w5369, s=w5373, f=w5370) -> (s? t:f=w5368:dbl)
            n1192 = Select(t=w5370, s=w5373, f=w5369) -> (s? t:f=w5372:dbl)
            n1193 = Subtract(x=w5380, y=w5372) -> (x-y=w5371:dbl)
            n1194 = Subtract(x=w5383, y=w5368) -> (x-y=w5367:dbl)
            n1195 = local read "2D or 1D Scan"() -> (w5385:bool)
            n1196 = Not(x=w5373) -> (.not. x?=w5379:bool)
            n1197 = Not(x=w5385) -> (.not. x?=w5381:bool)
            n1198 = And(x=w5373, y=w5381) -> (x .and. y?=w5382:bool)
            n1199 = And(x=w5381, y=w5379) -> (x .and. y?=w5384:bool)
            n1200 = Select(t=w5383, s=w5384, f=w5367) -> (s? t:f=w5374:dbl)
            n1201 = Select(t=w5380, s=w5382, f=w5371) -> (s? t:f=w5375:dbl)
            n1202 = call "Volt to I16.vi"("Voltage In"=w5375) -> ("I16 Voltage Out"=w5378:i16)
            n1203 = call "Volt to I16.vi"("Voltage In"=w5374) -> ("I16 Voltage Out"=w5377:i16)
            n1204 = xnode "Read/Write Control"("FPGA VI Reference In"=w5391, "error in"=w5390, "AI to FIFO"=w5387, "APD to FIFO"=w5387, "Start scan (MCL)"=w5387, "AO1"=w5378, "AO2"=w5377) -> ("FPGA VI Reference Out"=w5389:T15, "error out"=w5388:errorcluster)
          }
        }
        "Initial Y" <- w5263
        "Initial X" <- w5262
        "wait to reset values" <- w5264
      }
    }
    n1205 = local read "APD Elements/DMA read"() -> (w4455:u32)
    n1206 = local read "Elements/DMA read"() -> (w4510:u32)
    n1207 = xnode "Get APD Data"("FPGA VI Reference In"=w4487, "error in"=w4486, "Number of Elements"=w4455, "Timeout (ms)"=-1) -> ("Data"=w4454:u32[], "Elements Remaining"=→"APD FIFO Elements Remaining":u32)  [unwired: 2 out]
    n1208 = xnode "Get Trap Data"("FPGA VI Reference In"=w4487, "error in"=w4486, "Number of Elements"=w4510, "Timeout (ms)"=-1 ("Timeout")) -> ("FPGA VI Reference Out"=w4489:T15, "error out"=w4488:errorcluster, "Data"=w4626:u32[], "Elements Remaining"=w4656:u32)
    "FIFO El. Rem." <- w4656
    n1209 = local read "FIFO Depth"() -> (w4658:u32)
    n1210 = Subtract(x=w4658, y=w4510) -> (x-y=w4657:u32)
    n1211 = Divide(x=w4656, y=w4657) -> (x/y=w4655:dbl)
    "Buffer Status" <- w4655
    n1212 = Equal?(x=w4655, y=1.0) -> (x = y?=w4653:bool)
    n1213 = case "Alert buffer overflow" shown="True" w4653 {
      frame #0 {
      }
      frame #1 {
        n1214 = call <vilib>:"Beep.vi"() -> ()  [unwired: 3 in, 9 out]
        "Overflow (data lost)" <- TRUE ("Overflow (data lost)")
      }
    }
    n1215 = local read "FPGA Averaging"() -> (w4509:bool)
    n1216 = case "Special unpacking case if no averaging done by FPGA" shown="False" w4509 {
      tunnel: w4626 -> [w5668 w5694]
      tunnel: [w5639 w5669] -> w4625
      frame #0 {
        n1217 = Decimate 1D Array(w5668) -> (w5667:u32[], w5666:u32[], w5665:u32[], w5664:u32[])
        n1218 = Split Number(x=w5667) -> (hi(x)=w5663:u16[], lo(x)=w5662:u16[])
        n1219 = Split Number(x=w5666) -> (hi(x)=w5661:u16[], lo(x)=w5660:u16[])
        n1220 = Split Number(x=w5665) -> (hi(x)=w5659:u16[], lo(x)=w5658:u16[])
        n1221 = Split Number(x=w5664) -> (hi(x)=w5657:u16[], lo(x)=w5656:u16[])
        n1222 = To Word Integer(number=w5663) -> (16bit integer=w5655:i16[])
        n1223 = To Word Integer(number=w5662) -> (16bit integer=w5654:i16[])
        n1224 = To Word Integer(number=w5661) -> (16bit integer=w5653:i16[])
        n1225 = To Word Integer(number=w5660) -> (16bit integer=w5652:i16[])
        n1226 = To Word Integer(number=w5659) -> (16bit integer=w5651:i16[])
        n1227 = To Word Integer(number=w5658) -> (16bit integer=w5650:i16[])
        n1228 = To Word Integer(number=w5657) -> (16bit integer=w5649:i16[])
        n1229 = To Word Integer(number=w5656) -> (16bit integer=w5648:i16[])
        n1230 = To Double Precision Float(number=w5655) -> (double precision float=w5647:dbl[])
        n1231 = To Double Precision Float(number=w5654) -> (double precision float=w5646:dbl[])
        n1232 = To Double Precision Float(number=w5653) -> (double precision float=w5645:dbl[])
        n1233 = To Double Precision Float(number=w5652) -> (double precision float=w5644:dbl[])
        n1234 = To Double Precision Float(number=w5651) -> (double precision float=w5643:dbl[])
        n1235 = To Double Precision Float(number=w5650) -> (double precision float=w5642:dbl[])
        n1236 = To Double Precision Float(number=w5649) -> (double precision float=w5641:dbl[])
        n1237 = To Double Precision Float(number=w5648) -> (double precision float=w5640:dbl[])
        n1238 = Interleave 1D Arrays(w5647, w5646, w5645, w5644, w5643, w5642, w5641, w5640) -> (w5639:dbl[])
      }
      frame #1 {
        n1239 = Decimate 1D Array(w5694) -> (w5685:u32[], w5683:u32[], w5681:u32[], w5679:u32[], w5677:u32[], w5675:u32[], w5673:u32[], w5671:u32[])
        n1240 = To Long Integer(number=w5685) -> (32bit integer=w5693:i32[])
        n1241 = To Long Integer(number=w5683) -> (32bit integer=w5692:i32[])
        n1242 = To Long Integer(number=w5681) -> (32bit integer=w5691:i32[])
        n1243 = To Long Integer(number=w5679) -> (32bit integer=w5690:i32[])
        n1244 = To Long Integer(number=w5677) -> (32bit integer=w5689:i32[])
        n1245 = To Long Integer(number=w5675) -> (32bit integer=w5688:i32[])
        n1246 = To Long Integer(number=w5673) -> (32bit integer=w5687:i32[])
        n1247 = To Long Integer(number=w5671) -> (32bit integer=w5686:i32[])
        n1248 = To Double Precision Float(number=w5693) -> (double precision float=w5684:dbl[])
        n1249 = To Double Precision Float(number=w5692) -> (double precision float=w5682:dbl[])
        n1250 = To Double Precision Float(number=w5691) -> (double precision float=w5680:dbl[])
        n1251 = To Double Precision Float(number=w5690) -> (double precision float=w5678:dbl[])
        n1252 = To Double Precision Float(number=w5689) -> (double precision float=w5676:dbl[])
        n1253 = To Double Precision Float(number=w5688) -> (double precision float=w5674:dbl[])
        n1254 = To Double Precision Float(number=w5687) -> (double precision float=w5672:dbl[])
        n1255 = To Double Precision Float(number=w5686) -> (double precision float=w5670:dbl[])
        n1256 = Interleave 1D Arrays(w5684, w5682, w5680, w5678, w5676, w5674, w5672, w5670) -> (w5669:dbl[])
      }
    }
    n1257 = local read "FPGA Ave."() -> (w4508:dbl)
    n1258 = feedback #4(i16 -1 ("Trap Sets")) -> (w4506:i16)
    n1259 = feedback #5("" ("Detector Type")) -> (w4503:string)
    n1260 = Not Equal?(x=w4503, y="Detector Type") -> (x != y?=w4501:bool)
    n1261 = local read "Trap Sets"() -> (w4505:i16)
    n1262 = Not Equal?(x=w4506, y=w4505) -> (x != y?=w4500:bool)
    n1263 = Or(x=w4501, y=w4500) -> (x .or. y?=w4499:bool)
    n1264 = Divide(x=w4625, y=w4508) -> (x/y=w4633:dbl[])
    n1265 = case "Deinterlace trap data, average down PSD" shown="2" w4505 {
      tunnel: w4633 -> [w5713 w5778]
      tunnel: [w5710 w5775] -> w4493
      tunnel: [w5713 w5777] -> w4632
      tunnel: "Detector Type" -> [w5712 w5773]
      tunnel: [w5711 w5776] -> w4491
      tunnel: [w5709 w5774] -> w4624
      frame #0 {
        n1266 = Divide(x=w5713, y=3276.7) -> (x/y=w5714:dbl[])
        n1267 = Decimate 1D Array(w5714) -> (w5723:dbl[], w5722:dbl[], w5721:dbl[], w5720:dbl[], w5719:dbl[], w5718:dbl[], w5717:dbl[], w5716:dbl[])
        n1268 = case shown="\"IR-QPD + PSD + FB-QPD position\"" w5712 {
          tunnel: w5723 -> [w5747 w5772]
          tunnel: w5722 -> [w5746 w5771]
          tunnel: w5721 -> [w5731 w5749]
          tunnel: w5720 -> [w5732 w5759]
          tunnel: w5719 -> [w5745 w5770]
          tunnel: w5718 -> [w5744 w5769]
          tunnel: w5717 -> [w5728 w5750]
          tunnel: w5716 -> [w5727 w5748]
          tunnel: [w5726 w5756] -> w5711
          tunnel: [w5725 w5755] -> w5710
          tunnel: [w5724 w5754] -> w5709
          frame #0 {
            w5724 = 0  # Channel pattern
            n1269 = Divide(x=w5747, y=w5732) -> (x/y=w5734:dbl[])
            n1270 = Divide(x=w5746, y=w5732) -> (x/y=w5733:dbl[])
            n1271 = Divide(x=w5745, y=w5728) -> (x/y=w5730:dbl[])
            n1272 = Divide(x=w5744, y=w5727) -> (x/y=w5729:dbl[])
            n1273 = Build Array(w5734, w5733, w5732, w5731, w5730, w5729, w5728, w5727) -> (w5725:dbl[][])
            n1274 = Bundle("T1 Y", "T1 X", "T1 Sum", "FB Sum", "PSD Y", "PSD X", "PSD Y Sum", "PSD X Sum") -> (w5743:T38)  [unwired: 1 out]
            n1275 = Cluster To Array(cluster=w5743) -> (array=w5726:string[])
          }
          frame #1 {
            w5754 = 3  # Channel pattern
            n1276 = Negate(x=w5750) -> (-x=w5751:dbl[])
            n1277 = Divide(x=w5772, y=w5759) -> (x/y=w5761:dbl[])
            n1278 = Divide(x=w5771, y=w5759) -> (x/y=w5760:dbl[])
            n1279 = Divide(x=w5770, y=w5750) -> (x/y=w5758:dbl[])
            n1280 = Divide(x=w5769, y=w5751) -> (x/y=w5757:dbl[])
            n1281 = Build Array(w5761, w5760, w5759, w5748, w5749, w5758, w5757, w5750) -> (w5755:dbl[][])
            n1282 = Bundle("T1 Y", "T1 X", "T1 Sum", "FB X", "FB Sum", "PSD Y", "PSD X", "PSD Y Sum") -> (w5768:T38)  [unwired: 1 out]
            n1283 = Cluster To Array(cluster=w5768) -> (array=w5756:string[])
          }
        }
      }
      frame #1 {
        n1284 = case shown="\"IR-QPD + PSD + FB-QPD X position\"" w5773 {
          tunnel: w5778 -> [w5839 w5906 w5976]
          tunnel: [w5819 w5891 w5963] -> w5777
          tunnel: [w5805 w5882 w5954] -> w5776
          tunnel: [w5804 w5842 w5921] -> w5775
          tunnel: [w5798 w5880 w5952] -> w5774
          frame #0 {
            w5798 = 1  # Channel pattern
            # "time average x2 the 4th signal and the 4 psd signals (detection laser)"
            # "deinterlace 3 signals from qpd"
            n1285 = Decimate 1D Array(w5839) -> (w5838:dbl[], w5837:dbl[], w5803:dbl[], w5836:dbl[], w5826:dbl[], w5824:dbl[], w5823:dbl[], w5821:dbl[])
            n1286 = Decimate 1D Array(w5803) -> (w5802:dbl[], w5801:dbl[])
            n1287 = Decimate 1D Array(w5838) -> (w5835:dbl[], w5807:dbl[])
            n1288 = Decimate 1D Array(w5837) -> (w5834:dbl[], w5832:dbl[])
            n1289 = Decimate 1D Array(w5836) -> (w5833:dbl[], w5831:dbl[])
            n1290 = call "downsample 1D array - double.vi"("Ave N"=2.0, "Array In"=w5826) -> ("Array Out"=w5825:dbl[])  [unwired: 1 out]
            n1291 = call "downsample 1D array - double.vi"("Ave N"=2.0, "Array In"=w5824) -> ("Array Out"=w5806:dbl[])  [unwired: 1 out]
            n1292 = call "downsample 1D array - double.vi"("Ave N"=2.0, "Array In"=w5823) -> ("Array Out"=w5822:dbl[])  [unwired: 1 out]
            n1293 = call "downsample 1D array - double.vi"("Ave N"=2.0, "Array In"=w5821) -> ("Array Out"=w5820:dbl[])  [unwired: 1 out]
            n1294 = Interleave 1D Arrays(w5835, w5834, w5833, w5807, w5832, w5831, w5802, w5801, w5825, w5806, w5822, w5820) -> (w5819:dbl[])
            n1295 = Divide(x=w5819, y=3276.7) -> (x/y=w5818:dbl[])
            n1296 = Decimate 1D Array(w5818) -> (w5817:dbl[], w5816:dbl[], w5815:dbl[], w5814:dbl[], w5813:dbl[], w5812:dbl[], w5800:dbl[], w5799:dbl[], w5811:dbl[], w5810:dbl[], w5809:dbl[], w5808:dbl[])
            n1297 = Divide(x=w5817, y=w5815) -> (x/y=w5785:dbl[])
            n1298 = Divide(x=w5816, y=w5815) -> (x/y=w5784:dbl[])
            n1299 = Divide(x=w5814, y=w5812) -> (x/y=w5783:dbl[])
            n1300 = Divide(x=w5813, y=w5812) -> (x/y=w5782:dbl[])
            n1301 = Divide(x=w5811, y=w5809) -> (x/y=w5781:dbl[])
            n1302 = Divide(x=w5810, y=w5808) -> (x/y=w5780:dbl[])
            n1303 = Build Array(w5785, w5784, w5815, w5783, w5782, w5812, w5800, w5799, w5781, w5780, w5809, w5808) -> (w5804:dbl[][])
            n1304 = Bundle("T1 Y", "T1 X", "T1 Sum", "T2 Y", "T2 X", "T2 Sum", "T1 FB Sum", "T2 FB Sum", "PSD Y", "PSD X", "PSD Y Sum", "PSD X Sum") -> (w5786:T39)  [unwired: 1 out]
            n1305 = Cluster To Array(cluster=w5786) -> (array=w5805:string[])
          }
          frame #1 {
            w5880 = 2  # Channel pattern
            # "time average x2 the 3 psd signals (detection laser)"
            # "deinterlace 3 signals from qpds"
            n1306 = Decimate 1D Array(w5906) -> (w5905:dbl[], w5904:dbl[], w5881:dbl[], w5903:dbl[], w5894:dbl[], w5893:dbl[], w5892:dbl[], w5868:dbl[])
            n1307 = Decimate 1D Array(w5881) -> (w5863:dbl[], w5861:dbl[])
            n1308 = Decimate 1D Array(w5905) -> (w5902:dbl[], w5883:dbl[])
            n1309 = Decimate 1D Array(w5904) -> (w5901:dbl[], w5899:dbl[])
            n1310 = Decimate 1D Array(w5903) -> (w5900:dbl[], w5898:dbl[])
            n1311 = Decimate 1D Array(w5868) -> (w5864:dbl[], w5862:dbl[])
            n1312 = call "downsample 1D array - double.vi"("Ave N"=2.0, "Array In"=w5894) -> ("Array Out"=w5867:dbl[])  [unwired: 1 out]
            n1313 = call "downsample 1D array - double.vi"("Ave N"=2.0, "Array In"=w5893) -> ("Array Out"=w5866:dbl[])  [unwired: 1 out]
            n1314 = call "downsample 1D array - double.vi"("Ave N"=2.0, "Array In"=w5892) -> ("Array Out"=w5865:dbl[])  [unwired: 1 out]
            n1315 = Interleave 1D Arrays(w5902, w5901, w5900, w5883, w5899, w5898, w5864, w5863, w5862, w5861, w5867, w5866, w5865) -> (w5891:dbl[])
            n1316 = Divide(x=w5891, y=3276.7) -> (x/y=w5890:dbl[])
            n1317 = Decimate 1D Array(w5890) -> (w5889:dbl[], w5888:dbl[], w5887:dbl[], w5886:dbl[], w5885:dbl[], w5884:dbl[], w5853:dbl[], w5851:dbl[], w5850:dbl[], w5848:dbl[], w5847:dbl[], w5846:dbl[], w5843:dbl[])
            n1318 = Negate(x=w5843) -> (-x=w5841:dbl[])
            n1319 = Divide(x=w5847, y=w5843) -> (x/y=w5845:dbl[])
            n1320 = Divide(x=w5846, y=w5841) -> (x/y=w5844:dbl[])
            n1321 = Divide(x=w5889, y=w5887) -> (x/y=w5872:dbl[])
            n1322 = Divide(x=w5888, y=w5887) -> (x/y=w5871:dbl[])
            n1323 = Divide(x=w5886, y=w5884) -> (x/y=w5870:dbl[])
            n1324 = Divide(x=w5885, y=w5884) -> (x/y=w5869:dbl[])
            n1325 = Divide(x=w5853, y=w5851) -> (x/y=w5852:dbl[])
            n1326 = Divide(x=w5850, y=w5848) -> (x/y=w5849:dbl[])
            n1327 = Build Array(w5872, w5871, w5887, w5870, w5869, w5884, w5852, w5851, w5849, w5848, w5845, w5844, w5843) -> (w5842:dbl[][])
            n1328 = Bundle("T1 Y", "T1 X", "T1 Sum", "T2 Y", "T2 X", "T2 Sum", "T1 FB X", "T1 FB Sum", "T2 FB X", "T2 FB Sum", "PSD Y", "PSD X", "PSD Y Sum") -> (w5873:T40)  [unwired: 1 out]
            n1329 = Cluster To Array(cluster=w5873) -> (array=w5882:string[])
          }
          frame #2 {
            w5952 = 4  # Channel pattern
            # "time average x2 the 3 psd signals (detection laser)"
            # "deinterlace 3 signals from qpds"
            n1330 = Decimate 1D Array(w5976) -> (w5975:dbl[], w5974:dbl[], w5953:dbl[], w5973:dbl[], w5919:dbl[], w5965:dbl[], w5964:dbl[], w5941:dbl[])
            n1331 = Decimate 1D Array "Feedback Sum"(w5953) -> (w5937:dbl[], w5935:dbl[])
            n1332 = Decimate 1D Array "QPD Y"(w5975) -> (w5972:dbl[], w5955:dbl[])
            n1333 = Decimate 1D Array "QPD X"(w5974) -> (w5971:dbl[], w5969:dbl[])
            n1334 = Decimate 1D Array "Feedback Y"(w5919) -> (w5918:dbl[], w5917:dbl[])
            n1335 = Decimate 1D Array "QPD Sum"(w5973) -> (w5970:dbl[], w5968:dbl[])
            n1336 = Decimate 1D Array "Feedback X"(w5941) -> (w5938:dbl[], w5936:dbl[])
            n1337 = call "downsample 1D array - double.vi"("Ave N"=2.0, "Array In"=w5965) -> ("Array Out"=w5940:dbl[])  [unwired: 1 out]
            n1338 = call "downsample 1D array - double.vi"("Ave N"=2.0, "Array In"=w5964) -> ("Array Out"=w5939:dbl[])  [unwired: 1 out]
            n1339 = Interleave 1D Arrays(w5972, w5971, w5970, w5955, w5969, w5968, w5918, w5938, w5937, w5917, w5936, w5935, w5940, w5939) -> (w5963:dbl[])
            n1340 = Divide(x=w5963, y=3276.7) -> (x/y=w5962:dbl[])
            n1341 = Decimate 1D Array(w5962) -> (w5961:dbl[], w5960:dbl[], w5959:dbl[], w5958:dbl[], w5957:dbl[], w5956:dbl[], w5914:dbl[], w5928:dbl[], w5912:dbl[], w5913:dbl[], w5926:dbl[], w5910:dbl[], w5924:dbl[], w5922:dbl[])
            n1342 = Negate(x=w5922) -> (-x=w5920:dbl[])
            n1343 = Divide(x=w5924, y=w5920) -> (x/y=w5923:dbl[])
            n1344 = Divide(x=w5913, y=w5910) -> (x/y=w5909:dbl[])
            n1345 = Divide(x=w5914, y=w5912) -> (x/y=w5911:dbl[])
            n1346 = Divide(x=w5961, y=w5959) -> (x/y=w5945:dbl[])
            n1347 = Divide(x=w5960, y=w5959) -> (x/y=w5944:dbl[])
            n1348 = Divide(x=w5958, y=w5956) -> (x/y=w5943:dbl[])
            n1349 = Divide(x=w5957, y=w5956) -> (x/y=w5942:dbl[])
            n1350 = Divide(x=w5928, y=w5912) -> (x/y=w5927:dbl[])
            n1351 = Divide(x=w5926, y=w5910) -> (x/y=w5925:dbl[])
            n1352 = Build Array(w5945, w5944, w5959, w5943, w5942, w5956, w5911, w5927, w5912, w5909, w5925, w5910, w5923, w5922) -> (w5921:dbl[][])
            n1353 = Bundle("T1 Y", "T1 X", "T1 Sum", "T2 Y", "T2 X", "T2 Sum", "T1 FB Y", "T1 FB X", "T1 FB Sum", "T2 FB Y", "T2 FB X", "T2 FB Sum", "PSD X", "PSD Y Sum") -> (w5908:T41)  [unwired: 1 out]
            n1354 = Cluster To Array(cluster=w5908) -> (array=w5954:string[])
          }
        }
      }
    }
    n1355 = case "Update these things only if detector type or number of traps changes" shown="True" w4499 {
      tunnel: w4491 -> [_ w4781]
      frame #0 {
      }
      frame #1 {
        n1356 = property on="High Res. Display" class="Ring (strict)"("Strings []"=w4781) -> ()  [unwired: 2 in, 2 out]
        n1357 = Build Array (concatenate)(w4781, "none") -> (w4774:string[])
        n1358 = property on="FFT 1 Choice 1" class="Ring (strict)"("Strings []"=w4774) -> ()  [unwired: 2 in, 2 out]
        n1359 = property on="FFT 1 Choice 2" class="Ring (strict)"("Strings []"=w4774) -> ()  [unwired: 2 in, 2 out]
        n1360 = property on="FFT 2 Choice 1" class="Ring (strict)"("Strings []"=w4774) -> ()  [unwired: 2 in, 2 out]
        n1361 = property on="FFT 2 Choice 2" class="Ring (strict)"("Strings []"=w4774) -> ()  [unwired: 2 in, 2 out]
        n1362 = Bundle("APD 1", "APD 2") -> (w4777:cluster{string, string})  [unwired: 1 out]
        n1363 = Cluster To Array(cluster=w4777) -> (array=w4775:string[])
        n1364 = Build Array (concatenate)(w4775, w4774) -> (w4779:string[])
        n1365 = Array Size(array=w4779) -> (size(s)=w4780:i32)
        n1366 = property on="Signals to Plot" class="LstBox (strict)"("Item Names"=w4779) -> ()  [unwired: 2 in, 2 out]
        n1367 = property on="Signals to Plot" class="LstBox (strict)"("Number of Rows"=w4780) -> ()  [unwired: 2 in, 2 out]
        n1368 = property on="All Signals" class="WFChart (strict)"("LegNumRows"=w4780) -> ()  [unwired: 2 in, 2 out]
      }
    }
    n1369 = local read "Data points/scans (MCL)"() -> (w4595:dbl)
    n1370 = Increment(x=w4595) -> (x+1=w4596:dbl)
    n1371 = feedback #6(w4596) -> (w4599:dbl)
    n1372 = Select(t=0, s=w4586, f=w4599) -> (s? t:f=w4592:dbl)
    n1373 = To Word Integer(number=w4632) -> (16bit integer=w4659:i16[])
    n1374 = Decimate 1D Array(w4454) -> (w4485:u32[], w4622:u32[])
    n1375 = To Double Precision Float(number=w4485) -> (double precision float=w4484:dbl[])
    n1376 = Array Size(array=w4484) -> (size(s)=w4598:i32)
    n1377 = Add(x=w4598, y=w4592) -> (x+y=w4593:dbl)
    n1378 = Greater?(x=w4593, y=w4595) -> (0:w4594:bool)
    n1379 = local read "DMA Update Period (s)"() -> (w4512:dbl)
    n1380 = Select(t=w4592, s=w4594, f=w4593) -> (s? t:f=w4591:dbl)
    n1381 = Build Array(w4485, w4622) -> (w4583:u32[][])
    n1382 = local read "MCL Scanning"() -> (w4589:bool)
    n1383 = local read "Data Period (s)"() -> (w4470:dbl)
    n1384 = To Double Precision Float(number=w4583) -> (double precision float=w4584:dbl[][])
    n1385 = Not(x=w4594) -> (.not. x?=w4588:bool)
    n1386 = local read "APD Integration Time (s)"() -> (w4511:dbl)
    n1387 = And(x=w4588, y=w4589) -> (x .and. y?=w4590:bool)
    n1388 = feedback #7(0.0) -> (w4619:dbl)
    n1389 = Add(x=w4512, y=w4619) -> (x+y=w4628:dbl)
    n1390 = Or(x=w4590, y=w4586) -> (x .or. y?=w4587:bool)
    n1391 = Multiply(x=w4470, y="Trap Disp. Downsample") -> (x*y=w4468:dbl)
    "Display Period (s)" <- w4468
    n1392 = Equal?(x="Tab Control 6", y=T31."High Res Display") -> (x = y?=w4496:bool)
    n1393 = for {
      tunnel: [w5708] -> w4618 mode=indexing
      tunnel: w4619 -> [w5707]
      tunnel: "Trap Disp. Downsample" -> [w5704]
      tunnel: w4493 -> [w5702] mode=indexing
      tunnel: w4470 -> [w5701]
      tunnel: w4491 -> [w5700] mode=indexing
      tunnel: w4492 -> [w5699]
      tunnel: [w5698] -> w4441 mode=indexing
      tunnel: w4468 -> [w5697]
      workers-P: 4 -> [_]
      n1394 = Bundle By Name("Y"=w5702, "dt"=w5701) -> (w5703:waveform(dbl))  [unwired: 1 out]
      n1395 = Set Waveform Attribute(5:w5700, 6:w5699, 7:w5703) -> (3:w5698:waveform(dbl))  [unwired: 1 in, 2 out]
      n1396 = call "downsample 1D array - double.vi"("Ave N"=w5704, "Array In"=w5702) -> ("Array Out"=w5705:dbl[])  [unwired: 1 out]
      n1397 = To Time Stamp(1:w5707) -> (0:w5706:timestamp)
      n1398 = Bundle By Name(cluster=w5698, "t0"=w5706, "Y"=w5705, "dt"=w5697) -> (w5708:waveform(dbl))
    }
    n1399 = case "For plotting results of scanning MCL" shown="True" w4587 {
      tunnel: w4586 -> [_ w5231]
      tunnel: w4484 -> [_ w5244]
      tunnel: w4595 -> [_ _]
      tunnel: w4441 -> [_ w5215]
      tunnel: w4442 -> [_ w5147]
      tunnel: w4440 -> [_ w5145]
      tunnel: w4439 -> [_ w5144]
      frame #0 {
      }
      frame #1 {
        w5152 = u32 0 items=["Horizontal", "Vertical", "Central", "1st Diagonal", "2nd Diagonal"] ("Type of Symmetry")
        w5155 = u32 0 items=["Horizontal", "Vertical", "Central", "1st Diagonal", "2nd Diagonal"] ("Type of Symmetry")
        w5185 = u32 0 items=["Horizontal", "Vertical", "Central", "1st Diagonal", "2nd Diagonal"] ("Type of Symmetry")
        n1400 = Index Array(array=w5215, index=10) -> (element=w5221:waveform(dbl))
        n1401 = Index Array(array=w5215, index=11) -> (element=w5218:waveform(dbl))
        n1402 = Index Array(array=w5215, index="Channel") -> (element=w5217:waveform(dbl))
        n1403 = local read "Cycles/step (MCL)"() -> (w5169:u64)
        n1404 = Unbundle By Name(w5221) -> ("Y"=w5171:dbl[])
        n1405 = Unbundle By Name(w5218) -> ("Y"=w5173:dbl[])
        n1406 = Unbundle By Name(w5217) -> ("Y"=w5178:dbl[])
        n1407 = call "downsample 1D array - double.vi"("Ave N"=w5169, "Array In"=w5171) -> ("Array Out"=w5170:dbl[])  [unwired: 1 out]
        n1408 = call "downsample 1D array - double.vi"("Ave N"=w5169, "Array In"=w5173) -> ("Array Out"=w5172:dbl[])  [unwired: 1 out]
        n1409 = call "downsample 1D array - double.vi"("Ave N"=w5169, "Array In"=w5178) -> ("Array Out"=w5177:dbl[])  [unwired: 1 out]
        n1410 = feedback #8(w5244) -> (w5245:dbl[])
        n1411 = Build Array (concatenate)(w5245, w5244) -> (w5223:dbl[])
        n1412 = Select(t=w5244, s=w5231, f=w5223) -> (s? t:f=w5228:dbl[])
        n1413 = feedback #9(w5170) -> (w5232:dbl[])
        n1414 = Build Array (concatenate)(w5232, w5170) -> (w5220:dbl[])
        n1415 = feedback #10(w5177) -> (w5242:dbl[])
        n1416 = Build Array (concatenate)(w5242, w5177) -> (w5241:dbl[])
        n1417 = feedback #11(w5172) -> (w5234:dbl[])
        n1418 = Build Array (concatenate)(w5234, w5172) -> (w5235:dbl[])
        n1419 = Select(t=w5170, s=w5231, f=w5220) -> (s? t:f=w5174:dbl[])
        n1420 = Select(t=w5177, s=w5231, f=w5241) -> (s? t:f=w5176:dbl[])
        n1421 = Select(t=w5172, s=w5231, f=w5235) -> (s? t:f=w5175:dbl[])
        n1422 = local read "N APD Samp/step"() -> (w5227:dbl)
        n1423 = local read "Scan steps (MCL)"() -> (w5182:u64)
        n1424 = local read "Scan lines (y)"() -> (w5214:u64)
        n1425 = call "integrate 1D array interval - double.vi"("Ave N"=w5227, "Array In"=w5228) -> ("Array Out"=w5226:dbl[])  [unwired: 1 out]
        n1426 = Array Size(array=w5226) -> (size(s)=w5230:i32)
        n1427 = Multiply(x=w5182, y=u64 2) -> (x*y=w5229:u64)
        n1428 = Multiply(x=w5214, y=w5229) -> (x*y=w5239:u64)
        n1429 = Subtract(x=w5239, y=w5230) -> (x-y=w5168:u64)
        n1430 = call <vilib>:"Mean.vi"("X"=w5226) -> ("mean"=w5165:dbl)  [unwired: 1 out]
        n1431 = call <vilib>:"Mean.vi"("X"=w5174) -> ("mean"=w5158:dbl)  [unwired: 1 out]
        n1432 = call <vilib>:"Mean.vi"("X"=w5176) -> ("mean"=w5163:dbl)  [unwired: 1 out]
        n1433 = call <vilib>:"Mean.vi"("X"=w5175) -> ("mean"=w5161:dbl)  [unwired: 1 out]
        n1434 = Initialize Array(1.0 ("element"), w5168) -> (w5159:dbl[])
        n1435 = Multiply(x=w5159, y=w5165) -> (x*y=w5166:dbl[])
        n1436 = Multiply(x=w5159, y=w5161) -> (x*y=w5162:dbl[])
        n1437 = Multiply(x=w5159, y=w5163) -> (x*y=w5164:dbl[])
        n1438 = Multiply(x=w5159, y=w5158) -> (x*y=w5160:dbl[])
        n1439 = Build Array (concatenate)(w5226, w5166) -> (w5238:dbl[])
        n1440 = Build Array (concatenate)(w5174, w5160) -> (w5233:dbl[])
        n1441 = Build Array (concatenate)(w5176, w5164) -> (w5237:dbl[])
        n1442 = Build Array (concatenate)(w5175, w5162) -> (w5236:dbl[])
        n1443 = Reshape Array(w5238, w5214, w5229) -> (w5212:dbl[][])
        n1444 = Reshape Array(w5233, w5214, w5229) -> (w5195:dbl[][])
        n1445 = Reshape Array(w5237, w5214, w5229) -> (w5187:dbl[][])
        n1446 = Reshape Array(w5236, w5214, w5229) -> (w5202:dbl[][])
        n1447 = Index Array(array=w5212, index (row)=0) -> (element=→"Waveform Graph":dbl[])  [unwired: 1 in]
        n1448 = Array Subset(array=w5202, index (col)=0 ("index"), length (col)=w5182) -> (w5207:dbl[][])  [unwired: 2 in]
        n1449 = Array Subset(array=w5212, index (col)=0 ("index"), length (col)=w5182) -> (w5211:dbl[][])  [unwired: 2 in]
        n1450 = Array Subset(array=w5202, index (col)=w5182) -> (w5205:dbl[][])  [unwired: 3 in]
        n1451 = Array Subset(array=w5212, index (col)=w5182) -> (w5209:dbl[][])  [unwired: 3 in]
        n1452 = Array Subset(array=w5187, index (col)=0 ("index"), length (col)=w5182) -> (w5193:dbl[][])  [unwired: 2 in]
        n1453 = Array Subset(array=w5187, index (col)=w5182) -> (w5191:dbl[][])  [unwired: 3 in]
        n1454 = Array Subset(array=w5195, index (col)=0 ("index"), length (col)=w5182) -> (w5200:dbl[][])  [unwired: 2 in]
        n1455 = Array Subset(array=w5195, index (col)=w5182) -> (w5198:dbl[][])  [unwired: 3 in]
        n1456 = for {
          tunnel: w5207 -> [w5251] mode=indexing
          tunnel: [w5250] -> w5206 mode=indexing
          n1457 = Reverse 1D Array(array=w5251) -> (reversed array=w5250:dbl[])
        }
        n1458 = for {
          tunnel: w5211 -> [w5253] mode=indexing
          tunnel: [w5252] -> w5210 mode=indexing
          n1459 = Reverse 1D Array(array=w5253) -> (reversed array=w5252:dbl[])
        }
        n1460 = for {
          tunnel: w5193 -> [w5247] mode=indexing
          tunnel: [w5246] -> w5192 mode=indexing
          n1461 = Reverse 1D Array(array=w5247) -> (reversed array=w5246:dbl[])
        }
        n1462 = for {
          tunnel: w5200 -> [w5249] mode=indexing
          tunnel: [w5248] -> w5199 mode=indexing
          n1463 = Reverse 1D Array(array=w5249) -> (reversed array=w5248:dbl[])
        }
        n1464 = Add(x=w5206, y=w5205) -> (x+y=w5204:dbl[][])
        n1465 = Add(x=w5210, y=w5209) -> (x+y=w5184:dbl[][])
        n1466 = Add(x=w5192, y=w5191) -> (x+y=w5190:dbl[][])
        n1467 = Add(x=w5199, y=w5198) -> (x+y=w5197:dbl[][])
        n1468 = Divide(x=w5190, y=2) -> (x/y=w5188:dbl[][])
        n1469 = Divide(x=w5204, y=2) -> (x/y=w5148:dbl[][])
        n1470 = To Single Precision Float(number=w5184) -> (single precision float=w5183:sgl[][])
        n1471 = Divide(x=w5197, y=2) -> (x/y=w5150:dbl[][])
        n1472 = Transpose 2D Array(2D array=w5188) -> (transposed array=→"Data map":dbl[][])
        n1473 = To Single Precision Float(number=w5148) -> (single precision float=w5154:sgl[][])
        n1474 = To Single Precision Float(number=w5150) -> (single precision float=w5151:sgl[][])
        n1475 = call "IMAQ ArrayToImage"("Image Pixels (Float)"=w5183, "Image"=w5147) -> ("Image Out"=w5186:T2)  [unwired: 8 in, 1 out]
        n1476 = call "IMAQ ArrayToImage"("Image Pixels (Float)"=w5154, "Image"=w5145) -> ("Image Out"=w5156:T2)  [unwired: 8 in, 1 out]
        n1477 = call "IMAQ Symmetry"("Type of Symmetry"=w5185, "Image Src"=w5186) -> ("Image Dst Out"=w5180:T2)  [unwired: 3 in, 1 out]
        n1478 = call "IMAQ ArrayToImage"("Image Pixels (Float)"=w5151, "Image"=w5144) -> ("Image Out"=w5153:T2)  [unwired: 8 in, 1 out]
        n1479 = call "IMAQ Symmetry"("Type of Symmetry"=w5155, "Image Src"=w5156) -> ("Image Dst Out"=→"Detection Laser X":T2)  [unwired: 3 in, 1 out]
        n1480 = call "IMAQ Symmetry"("Type of Symmetry"=w5152, "Image Src"=w5153) -> ("Image Dst Out"=→"Detection Laser Y":T2)  [unwired: 3 in, 1 out]
        n1481 = call "IMAQ Set Simple Calibration"("Calibration Axis Info"=T32 {"Origin Pixel"={"X"=0.0, "Y"=0.0}, "Angle Relative to Horizontal (deg)"=0.0, "Axis Reference"=0}, "Grid Descriptor"=T33 {"X Step"=0.3, "Y Step"=0.3, "Unit"=enum."Undefined"}, "Image"=w5180) -> ("Calibrated Image"=→"APD 1":T2)  [unwired: 7 in, 1 out]
      }
    }
    n1482 = Reciprocal(x=w4468) -> (1/x=→"Trap Disp. Freq. (Hz)":dbl)
    n1483 = case shown="True" w4496 {
      tunnel: w4441 -> [_ w4750]
      frame #0 {
      }
      frame #1 {
        n1484 = Index Array(array=w4750, index="High Res. Display") -> (element=w4751:waveform(dbl))
        n1485 = call <vilib>:"Std Deviation and Variance.vi"("X"=w4751) -> ("mean"=w4758:dbl, "standard deviation"=w4763:dbl)  [unwired: 1 in, 1 out]
        "Mean Intensity" <- w4758
        "Sigma" <- w4763
        n1486 = Subtract(x=w4751, y=w4758) -> (x-y=w4757:waveform(dbl))
        n1487 = Select(t=w4757, s="Subtract mean", f=w4751) -> (s? t:f=→"1 Channel":waveform(dbl))
        n1488 = Divide(x=w4763, y=w4758) -> (x/y=→"Sigma/Mean":dbl)
        n1489 = feedback #12(1) -> (w4752:i32)
        n1490 = Greater Or Equal?(x=w4752, y="Slow mean N ave.") -> (x >= y?=w4765:bool)
        n1491 = Increment(x=w4752) -> (x+1=w4767:i32)
        n1492 = Select(t=1, s=w4765, f=w4767) -> (s? t:f=w4754:i32)
        n1493 = feedback #13() -> (w4755:waveform(dbl))  [unwired: 1 out]
        n1494 = case shown="Default" w4752 {
          tunnel: [w4770 w4773] -> w4756
          tunnel: w4755 -> [w4772 _]
          tunnel: w4751 -> [w4771 w4773]
          frame #0 {
            n1495 = call-poly <vilib>:"Append Waveforms.vi"("waveform B"=w4771, "waveform A"=w4772) -> ("waveform out"=w4770:waveform(dbl))  [unwired: 1 in, 8 out]
          }
          frame #1 {
          }
        }
        n1496 = case shown="True" w4765 {
          tunnel: w4756 -> [_ w4769]
          frame #0 {
          }
          frame #1 {
            n1497 = call <vilib>:"Mean.vi"("X"=w4769) -> ("mean"=→"Slow mean":dbl)  [unwired: 1 out]
          }
        }
      }
    }
    n1498 = case "For computing FFTs for display" shown="True" "Compute FFT" {
      tunnel: w4441 -> [_ w6593]
      frame #0 {
      }
      frame #1 {
        n1499 = Build Array("FFT 1 Choice 1", "FFT 1 Choice 2", "FFT 2 Choice 1", "FFT 2 Choice 2") -> (w6586:u16[])
        n1500 = Array Size(array=w6593) -> (size(s)=w6592:i32)
        n1501 = feedback #14(u16[] [100, 100, 100, 100]) -> (w6587:u16[])
        n1502 = feedback #15("# Spectra to Ave.") -> (w6584:dbl)
        n1503 = Not Equal?(x="# Spectra to Ave.", y=w6584) -> (x != y?=w6583:bool)
        n1504 = Not Equal?(x=w6586, y=w6587) -> (x != y?=w6585:bool)
        n1505 = feedback #16(1.0) -> (w6570:dbl)
        n1506 = Compound Arithmetic op=OR("Reset FFT", w6585, w6583) -> (w6568:bool)
        n1507 = Select(t=1.0, s=w6568, f=w6570) -> (s? t:f=w6572:dbl)
        n1508 = Greater?(x=w6572, y="# Spectra to Ave.") -> (0:w6591:bool)
        n1509 = Increment(x=w6572) -> (x+1=w6571:dbl)
        n1510 = local read "DMA Update Period (s)"() -> (w6566:dbl)
        n1511 = Multiply(x="# Spectra to Ave.", y=w6566) -> (x*y=→"Ave. Time (s)":dbl)
        n1512 = Build Array(cluster{"f0":dbl, "df":dbl, "magnitude":dbl[]} {"f0"=0.0, "df"=0.0, "magnitude"=[]} ("PSD")) -> (w6575:cluster{"f0":dbl, "df":dbl, "magnitude":dbl[]}[])
        n1513 = Build Array(w6575, w6575, w6575, w6575) -> (w6577:T42)
        n1514 = feedback #17(w6577) -> (w6582:T42)
        n1515 = for {
          N: 4 -> [_]
          tunnel: w6586 -> [w6615] mode=indexing
          tunnel: w6593 -> [w6616]
          tunnel: w6592 -> [w6618]
          tunnel: w6568 -> [w6611]
          tunnel: w6591 -> [w6610]
          tunnel: "# Spectra to Ave." -> [w6609]
          tunnel: [w6608] -> w6581 mode=indexing
          tunnel: w6582 -> [w6613] mode=indexing
          tunnel: [w6612] -> w6569 mode=indexing
          tunnel: w6572 -> [w6607]
          n1516 = Less?(x=w6615, y=w6618) -> (x < y?=w6617:bool)
          n1517 = Index Array(array=w6616, index=w6615) -> (element=w6614:waveform(dbl))
          n1518 = case shown="True" w6617 {
            tunnel: w6614 -> [_ w6635]
            tunnel: w6613 -> [w6620 w6633]
            tunnel: [w6620 w6621] -> w6612
            tunnel: w6611 -> [_ w6632]
            tunnel: w6610 -> [_ w6625]
            tunnel: w6609 -> [_ w6624]
            tunnel: [cluster{"f0":dbl, "df":dbl, "magnitude":dbl[]} {"f0"=0.0, "df"=0.0, "magnitude"=[]} ("PSD") w6626] -> w6608
            tunnel: w6607 -> [_ w6623]
            frame #0 {
            }
            frame #1 {
              n1519 = call <vilib>:"Std Deviation and Variance.vi"("X"=w6635) -> ("mean"=w6636:dbl)  [unwired: 1 in, 2 out]
              n1520 = Subtract(x=w6635, y=w6636) -> (x-y=w6634:waveform(dbl))
              n1521 = xnode "Spectral Measurements"("Signals"=w6634) -> ("PSD"=w6628:cluster{"f0":dbl, "df":dbl, "magnitude":dbl[]})  [unwired: 1 in, 1 out]
              n1522 = case shown="False" w6632 {
                tunnel: w6633 -> [w6645 _]
                tunnel: [w6641 w6650] -> w6621
                tunnel: w6628 -> [w6644 w6651]
                tunnel: w6625 -> [w6643 _]
                frame #0 {
                  n1523 = Build Array (concatenate)(w6645, w6644) -> (w6642:cluster{"f0":dbl, "df":dbl, "magnitude":dbl[]}[])
                  n1524 = case shown="True" w6643 {
                    tunnel: w6642 -> [w6646 w6649]
                    tunnel: [w6646 w6647] -> w6641
                    frame #0 {
                    }
                    frame #1 {
                      n1525 = Delete From Array(array=w6649, index=0) -> (array with subset deleted=w6647:cluster{"f0":dbl, "df":dbl, "magnitude":dbl[]}[])  [unwired: 1 in, 1 out]
                    }
                  }
                }
                frame #1 {
                  n1526 = Build Array(w6651) -> (w6650:cluster{"f0":dbl, "df":dbl, "magnitude":dbl[]}[])
                }
              }
              n1527 = for {
                tunnel: w6621 -> [w6640] mode=indexing
                tunnel: [w6639] -> w6631 mode=indexing
                n1528 = Unbundle By Name(w6640) -> ("magnitude"=w6639:dbl[])
              }
              n1529 = Transpose 2D Array(2D array=w6631) -> (transposed array=w6630:dbl[][])
              n1530 = for {
                tunnel: w6630 -> [w6638] mode=indexing
                tunnel: [w6637] -> w6629 mode=indexing
                n1531 = Add Array Elements(numeric array=w6638) -> (sum=w6637:dbl)
              }
              n1532 = Select(t=w6624, s=w6625, f=w6623) -> (s? t:f=w6622:dbl)
              n1533 = Divide(x=w6629, y=w6622) -> (x/y=w6627:dbl[])
              n1534 = Bundle By Name(cluster=w6628, "magnitude"=w6627) -> (w6626:cluster{"f0":dbl, "df":dbl, "magnitude":dbl[]})
            }
          }
        }
        n1535 = case shown="True" w6568 {
          tunnel: w6569 -> [w6600 w6606]
          tunnel: [w6600 w6601] -> w6567
          frame #0 {
          }
          frame #1 {
            n1536 = Array Subset(array=w6606, index (row)=0 ("index"), length (row)=4 ("length"), index (col)=0 ("index"), length (col)=1 ("length")) -> (w6601:T42)
          }
        }
        n1537 = Split 1D Array(array=w6581, index=2) -> (first subarray=→"FFT 1":cluster{"f0":dbl, "df":dbl, "magnitude":dbl[]}[], second subarray=→"FFT 2":cluster{"f0":dbl, "df":dbl, "magnitude":dbl[]}[])
      }
    }
    n1538 = Bundle("APD 1", "APD 2") -> (w4616:cluster{string, string})  [unwired: 1 out]
    n1539 = Cluster To Array(cluster=w4616) -> (array=w4613:string[])
    n1540 = for {
      tunnel: w4584 -> [w5628] mode=indexing
      tunnel: w4619 -> [w5637]
      tunnel: w4511 -> [w5636]
      tunnel: [w5632] -> w4617 mode=indexing
      tunnel: "APD Disp. Scale" -> [w5633]
      tunnel: w4492 -> [w5631]
      tunnel: w4613 -> [w5630] mode=indexing
      tunnel: "APD Disp. Downsample" -> [w5626]
      tunnel: [w5629] -> w4612
      workers-P: 2 -> [_]
      n1541 = call "integrate 1D array interval - double.vi"("Ave N"=w5626, "Array In"=w5628) -> ("Array Out"=w5627:dbl[])  [unwired: 1 out]
      n1542 = Multiply(x=w5636, y=w5626) -> (x*y=w5629:dbl)
      n1543 = Divide(x=w5627, y=w5633) -> (x/y=w5634:dbl[])
      n1544 = To Time Stamp(1:w5637) -> (0:w5638:timestamp)
      n1545 = Bundle By Name("t0"=w5638, "Y"=w5634, "dt"=w5629) -> (w5635:waveform(dbl))  [unwired: 1 out]
      n1546 = Set Waveform Attribute(5:w5630, 6:w5631, 7:w5635) -> (3:w5632:waveform(dbl))  [unwired: 1 in, 2 out]
    }
    "APD Display Period (s)" <- w4612
    n1547 = Reciprocal(x=w4612) -> (1/x=→"APD Display Freq. (Hz)":dbl)
    n1548 = feedback #18(w4485) -> (w4582:u32[])
    n1549 = Build Array (concatenate)(w4582, w4485) -> (w4579:u32[])
    n1550 = Array Size(array=w4579) -> (size(s)=w4576:i32)
    n1551 = Array Size(array=w4485) -> (size(s)=w4578:i32)
    n1552 = local read "APD Integration Time (s)"() -> (w4445:dbl)
    n1553 = Build Array (concatenate)(w4617, w4618) -> (w4437:waveform(dbl)[])
    "All Signals" <- w4437
    n1554 = Multiply(x=w4578, y="APD Ave N") -> (x*y=w4577:dbl)
    n1555 = Greater?(x=w4576, y=w4577) -> (0:w4580:bool)
    n1556 = Index Array(array=w4437, index=0) -> (element=w4569:waveform(dbl))
    n1557 = case shown="True" w4580 {
      tunnel: w4579 -> [w5138 w5143]
      tunnel: [w5138 w5139] -> w4517
      tunnel: w4577 -> [_ w5141]
      tunnel: w4576 -> [_ w5142]
      frame #0 {
      }
      frame #1 {
        n1558 = Subtract(x=w5142, y=w5141) -> (x-y=w5140:dbl)
        n1559 = Array Subset(array=w5143, index=w5140, length=w5141) -> (w5139:u32[])
      }
    }
    n1560 = Multiply(x="APD Disp. Scale", y=w4569) -> (x*y=w4447:waveform(dbl))
    n1561 = Multiply(x="APD Disp. Downsample", y=w4445) -> (x*y=w4443:dbl)
    n1562 = Divide(x=w4447, y=w4443) -> (x/y=w4436:waveform(dbl))
    "APD 1 Chart" <- w4436
    n1563 = Index Array(array=w4437, index=3) -> (element=w4528:waveform(dbl))
    n1564 = Index Array(array=w4437, index=6) -> (element=w4525:waveform(dbl))
    n1565 = Array Size(array=w4517) -> (size(s)=w4574:i32)
    n1566 = Add Array Elements(numeric array=w4517) -> (sum=w4585:u32)
    n1567 = call <vilib>:"Std Deviation and Variance.vi"("X"=w4517) -> ("standard deviation"=w4516:dbl)  [unwired: 1 in, 2 out]
    n1568 = Divide(x="T1 offset_x (mV)", y=1000.0) -> (x/y=w4529:dbl)
    n1569 = Multiply(x=w4511, y=w4574) -> (x*y=w4575:dbl)
    "Int. Time (s)" <- w4575
    n1570 = Divide(x=w4585, y=w4575) -> (x/y=w4514:dbl)
    "APD 1 Rate (Hz)" <- w4514
    n1571 = Divide(x=w4516, y=w4511) -> (x/y=w4515:dbl)
    "Rate sigma (Hz)" <- w4515
    n1572 = Divide(x=w4515, y=w4514) -> (x/y=→"sigma/mean":dbl)
    n1573 = Divide(x="T2 offset_x (mV)", y=1000.0) -> (x/y=w4527:dbl)
    n1574 = case shown="0, Default" "Calibration" {
      tunnel: "T1 alpha_x (nm/V)" -> [_ w5115 w5136]
      tunnel: "T1 kappa_x (pN/nm)" -> [_ _ w5126]
      tunnel: "T2 alpha_x (nm/V)" -> [_ w5114 w5134]
      tunnel: "T2 kappa_x (pN/nm)" -> [_ _ w5127]
      tunnel: w4528 -> [w5097 w5112 w5132]
      tunnel: w4525 -> [w5096 w5110 w5130]
      tunnel: [w5097 w5109 w5129] -> w4558
      tunnel: [w5096 w5108 w5128] -> w4557
      tunnel: ["T1 X (V)" ("Label.Text") "T1 X (nm)" ("Label.Text") "T1 X (pN)" ("Label.Text")] -> w4546
      tunnel: ["T2 X (V)" ("Label.Text") "T2 X (nm)" ("Label.Text") "T2 X (pN)" ("Label.Text")] -> w4545
      tunnel: ["Position (V)" ("Label.Text") "Position (nm)" ("Label.Text") "Force (pN)" ("Label.Text")] -> w4547
      tunnel: w4527 -> [_ w5100 w5119]
      tunnel: w4529 -> [_ w5103 w5121]
      tunnel: ["Mean (V)" ("Label.Text") "Mean (nm)" ("Label.Text") "Mean (pN)" ("Label.Text")] -> w4542
      tunnel: ["Difference (V)" ("Label.Text") "Difference (nm)" ("Label.Text") "Difference (pN)" ("Label.Text")] -> w4448
      frame #0 {
      }
      frame #1 {
        n1575 = Unbundle By Name(w5112) -> ("Y"=w5116:dbl[])
        n1576 = Unbundle By Name(w5110) -> ("Y"=w5101:dbl[])
        n1577 = Subtract(x=w5116, y=w5103) -> (x-y=w5104:dbl[])
        n1578 = Subtract(x=w5101, y=w5100) -> (x-y=w5102:dbl[])
        n1579 = Multiply(x=w5102, y=w5114) -> (x*y=w5111:dbl[])
        n1580 = Multiply(x=w5115, y=w5104) -> (x*y=w5113:dbl[])
        n1581 = Bundle By Name(cluster=w5110, "Y"=w5111) -> (w5108:waveform(dbl))
        n1582 = Bundle By Name(cluster=w5112, "Y"=w5113) -> (w5109:waveform(dbl))
      }
      frame #2 {
        n1583 = Unbundle By Name(w5132) -> ("Y"=w5137:dbl[])
        n1584 = Unbundle By Name(w5130) -> ("Y"=w5135:dbl[])
        n1585 = Subtract(x=w5135, y=w5119) -> (x-y=w5120:dbl[])
        n1586 = Subtract(x=w5137, y=w5121) -> (x-y=w5122:dbl[])
        n1587 = Compound Arithmetic op=MULTIPLY(w5120, w5134, w5127) -> (w5131:dbl[])
        n1588 = Compound Arithmetic op=MULTIPLY(w5126, w5136, w5122) -> (w5133:dbl[])
        n1589 = Bundle By Name(cluster=w5130, "Y"=w5131) -> (w5128:waveform(dbl))
        n1590 = Bundle By Name(cluster=w5132, "Y"=w5133) -> (w5129:waveform(dbl))
      }
    }
    n1591 = feedback #19(u16 1 ("Calibration")) -> (w4549:u16)
    n1592 = case shown="True" "Read Lateness and Rel Phase" {
      tunnel: w4489 -> [w4783 w4801]
      tunnel: w4488 -> [w4784 w4800]
      tunnel: [w4783 w4799] -> w4520
      tunnel: [w4784 w4798] -> w4519
      frame #0 {
      }
      frame #1 {
        n1593 = xnode "Read/Write Control"("FPGA VI Reference In"=w4801, "error in"=w4800) -> ("FPGA VI Reference Out"=w4799:T15, "error out"=w4798:errorcluster, "GI Relative phase"=→"GI relative phase":i16, "Relative phase"=→"Relative phase (AI1)":i16, "AI Late Counter"=→"Late Counter (AI1)":u32, "GI Late Counter"=→"GI Late Counter":u32, "MCL Late Counter"=→"MCL Late Counter":u32, "MCL Relative Phase"=→"Relative Phase (MCL)":i16, "APD Acq Relative Phase"=→"APD Acq Relative Phase":i16, "APD Gate Relative Phase"=→"APD Gate Relative Phase":i16, "APD Acq Late Counter"=→"APD Acq Late Counter":u32, "APD Gate Late Counter"=→"APD Gate Late Counter":u32, "Green FB Relative Phase"=→"Relative phase (Green FB)":i16, "GI Relative phase 2"=→"GI relative phase 2":i16, "GI Late Counter 2"=→"GI Late Counter 2":u32)
      }
    }
    n1594 = Not Equal?(x=w4549, y="Calibration") -> (x != y?=w4494:bool)
    n1595 = Unbundle By Name(w4528) -> ("Y"=w4531:dbl[])
    n1596 = Unbundle By Name(w4525) -> ("Y"=w4534:dbl[])
    n1597 = Subtract(x=w4531, y=w4529) -> (x-y=w4532:dbl[])
    n1598 = Subtract(x=w4534, y=w4527) -> (x-y=w4533:dbl[])
    n1599 = Multiply(x=w4533, y="T2 alpha_x (nm/V)") -> (x*y=w4524:dbl[])
    n1600 = Multiply(x="T1 alpha_x (nm/V)", y=w4532) -> (x*y=w4523:dbl[])
    n1601 = Multiply(x=w4557, y=-1.0) -> (x*y=w4536:waveform(dbl))
    n1602 = Subtract(x=w4524, y=w4523) -> (x-y=w4522:dbl[])
    n1603 = Unbundle By Name(w4557) -> ("Y"=w4476:dbl[])
    n1604 = Unbundle By Name(w4558) -> ("Y"=w4477:dbl[])
    n1605 = Build Array(w4558, w4536) -> (→"Force":waveform(dbl)[])
    n1606 = Subtract(x=w4522, y="Offset (nm)") -> (x-y=w4474:dbl[])
    n1607 = call <vilib>:"Mean.vi"("X"=w4476) -> ("mean"=w4452:dbl)  [unwired: 1 out]
    "T2 X" <- w4452
    n1608 = Absolute Value(x=w4477) -> (abs(x)=w4478:dbl[])
    n1609 = Absolute Value(x=w4476) -> (abs(x)=w4479:dbl[])
    n1610 = call <vilib>:"Mean.vi"("X"=w4477) -> ("mean"=w4453:dbl)  [unwired: 1 out]
    "T1 X" <- w4453
    n1611 = Add(x=w4478, y=w4479) -> (x+y=w4480:dbl[])
    n1612 = Bundle By Name(cluster=w4528, "Y"=w4474) -> (w4435:waveform(dbl))
    "Bead Separation" <- w4435
    n1613 = Divide(x=w4480, y=2.0) -> (x/y=→"Vec Mean of T1 T2":dbl[])
    n1614 = case shown="True" w4494 {
      tunnel: w4547 -> [_ w5090]
      tunnel: w4546 -> [_ w5089]
      tunnel: w4545 -> [_ w5088]
      tunnel: w4542 -> [_ w5087]
      tunnel: w4448 -> [_ w5086]
      frame #0 {
      }
      frame #1 {
        n1615 = property on="Force" class="WFChart (strict)"("YScale.NameLbl.Text"=w5090) -> ()  [unwired: 2 in, 2 out]
        n1616 = property on="T2 X" class="DigNum (strict)"("Caption.Text"=w5088) -> ()  [unwired: 2 in, 2 out]
        n1617 = property on="T1 X" class="DigNum (strict)"("Caption.Text"=w5089) -> ()  [unwired: 2 in, 2 out]
        n1618 = property on="Mean" class="DigNum (strict)"("Caption.Text"=w5087) -> ()  [unwired: 2 in, 2 out]
        n1619 = property on="Difference" class="DigNum (strict)"("Caption.Text"=w5086) -> ()  [unwired: 2 in, 2 out]
      }
    }
    n1620 = local read "Tether"() -> (w4483:bool)
    n1621 = Absolute Value(x=w4453) -> (abs(x)=w4450:dbl)
    n1622 = Absolute Value(x=w4452) -> (abs(x)=w4449:dbl)
    n1623 = local read "Display Period (s)"() -> (w4467:dbl)
    n1624 = Add(x=w4450, y=w4449) -> (x+y=w4544:dbl)
    n1625 = Subtract(x=w4450, y=w4449) -> (x-y=→"Difference":dbl)
    n1626 = feedback #20(w4474) -> (w4473:dbl[])
    n1627 = Divide(x=w4544, y=2.0) -> (x/y=w4482:dbl)
    "Mean" <- w4482
    n1628 = case shown="True" w4483 {
      tunnel: w4482 -> [_ w4737]
      frame #0 {
      }
      frame #1 {
        n1629 = Greater?(x="Lost Tether Alarm Threshold (pN)", y=w4737) -> (0:w4735:bool)
        n1630 = case shown="True" w4735 {
          frame #0 {
          }
          frame #1 {
            n1631 = local read "Time tether formed"() -> (w4743:timestamp)
            n1632 = flat-sequence {
              frame #0 {
                # "stop only if saving"
                n1633 = local read "Saving..."() -> (w4748:bool)
                n1634 = local write "Stop Saving"(w4748) -> ()
              }
              frame #1 {
                w4749 = FALSE ("Fl. Triggered...")
                n1635 = property on="Green Laser ON/Interlacing" class="Bool (strict)"("Val(Sgnl)"=w4749) -> ()  [unwired: 2 in, 2 out]
                n1636 = local write "Fl. Triggered..."(w4749) -> ()
              }
            }
            n1637 = Get Date/Time In Seconds() -> (seconds since 1Jan1904=w4744:timestamp)
            n1638 = Subtract(x=w4744, y=w4743) -> (x-y=w4742:dbl)
            n1639 = Number To Decimal String(number=w4742) -> (decimal integer string=w4739:string)  [unwired: 1 out]
            n1640 = local read "Messages"() -> (w4746:string)
            n1641 = call <vilib>:"Beep.vi"() -> ()  [unwired: 3 in, 9 out]
            n1642 = Concatenate Strings("Lost tether (" ("Message to add"), w4739, " s)." ("string")) -> (w4741:string)
            n1643 = local write "Tether"(FALSE ("Tether")) -> ()
            n1644 = call "Update messages.vi"("Message to add"=w4741, "Old message string"=w4746) -> ("New message string"=w4745:string)
            n1645 = local write "Messages"(w4745) -> ()
          }
        }
      }
    }
    n1646 = Build Array (concatenate)(w4474, w4473) -> (w4472:dbl[])
    n1647 = Divide(x="Bead Sep. Int. Time (s)", y=w4467) -> (x/y=w4466:dbl)
    n1648 = Split 1D Array(array=w4472, index=w4466) -> (first subarray=w4465:dbl[])  [unwired: 1 out]
    n1649 = xnode "Read/Write Control"("FPGA VI Reference In"=w4520, "error in"=w4519) -> ("FPGA VI Reference Out"=w4648:T15, "error out"=w4642:errorcluster, "AI2 Y Sum Set 1"=w4638:i16, "AI2 Y Sum Set 2"=w4637:i16, "Scanning"=→"AOD Scanning":bool, "Scan I"=→"AOD Scan I":u64, "Scanning MCL"=w4640:bool, "Scan I (MCL)"=→"MCL Scan I":u64, "Green FB Signals"=w4567:T37)  [unwired: 1 out]
    "MCL Scanning" <- w4640
    n1650 = call <vilib>:"Mean.vi"("X"=w4465) -> ("mean"=w4464:dbl)  [unwired: 1 out]
    "Bead Mean (nm)" <- w4464
    n1651 = Subtract(x=w4465, y=w4464) -> (x-y=w4463:dbl[])
    n1652 = Square(x=w4463) -> (x^2=w4462:dbl[])
    n1653 = call <vilib>:"Mean.vi"("X"=w4462) -> ("mean"=w4461:dbl)  [unwired: 1 out]
    n1654 = Square Root(x=w4461) -> (sqrt(x)=w4460:dbl)
    n1655 = Multiply(x=10.0, y=w4460) -> (x*y=→"RMS (Ang)":dbl)
    n1656 = flat-sequence "To save data" {
      tunnel: [w7034] -> w4661
      tunnel: [w7035] -> w4660
      tunnel: w4601 -> [w7028]
      tunnel: w4470 -> [w7032]
      tunnel: ["Save Calibration"] -> w4629
      tunnel: w4624 -> [w7031]
      tunnel: [w7024] -> w4623
      tunnel: [w7021] -> w4621
      tunnel: [w7018] -> w4620
      tunnel: w4600 -> [w7020]
      tunnel: w4491 -> [w7014]
      tunnel: [w7014] -> w4490
      tunnel: ["Start Saving"] -> w4438
      tunnel: w4661 -> [w7224]
      tunnel: w4660 -> [w7223]
      tunnel: w4659 -> [w7222]
      tunnel: w4629 -> [w7221]
      tunnel: w4623 -> [w7219]
      tunnel: w4621 -> [w7218]
      tunnel: w4620 -> [w7217]
      tunnel: w4454 -> [w7216]
      tunnel: w4512 -> [w7215]
      tunnel: w4490 -> [w7214]
      tunnel: w4438 -> [w7213]
      tunnel: w4436 -> [w7212]
      tunnel: w4435 -> [w7211]
      frame #0 {
        n1657 = Or(x="Save N Sets", y="Start Saving") -> (x .or. y?=w7015:bool)
        n1658 = To Double Precision Float(number=w7031) -> (double precision float=w7025:dbl)
        n1659 = Build Array(w7015, "Save Calibration", w7028, w7020) -> (w7030:bool[])
        n1660 = Compound Arithmetic op=OR("Save Calibration", w7028, w7015, w7020) -> (w7033:bool)
        n1661 = Boolean Array To Number(Boolean array=w7030) -> (number=w7027:u32)
        n1662 = feedback #21(refnum<k0> refnum) -> (w7036:refnum<file>)
        n1663 = feedback #22(FALSE ("Save APD Data\nwith Trap Data")) -> (w7019:bool)
        n1664 = feedback #23(refnum<k0> refnum) -> (w7022:refnum<file>)
        n1665 = feedback #24(0) -> (w7038:i32)
        n1666 = feedback #25() -> (w7026:u32)  [unwired: 1 out]
        n1667 = case shown="True" w7033 {
          tunnel: [w7043 1] -> w7034
          tunnel: w7038 -> [w7045 _]
          tunnel: [w7044 w7058] -> w7035
          tunnel: w7036 -> [w7044 _]
          tunnel: w7032 -> [_ w7078]
          tunnel: w7025 -> [_ w7076]
          tunnel: w7027 -> [_ w7079]
          tunnel: [w7042 w7057] -> w7024
          tunnel: w7026 -> [w7042 _]
          tunnel: [w7041 w7054] -> w7021
          tunnel: w7022 -> [w7041 _]
          tunnel: [w7040 w7053] -> w7018
          tunnel: w7019 -> [w7040 _]
          tunnel: "Start Saving" -> [_ w7051]
          tunnel: w7014 -> [_ w7050]
          frame #0 {
            n1668 = Increment(x=w7045) -> (x+1=w7043:i32)
          }
          frame #1 {
            w7046 = FALSE ("Start Saving")
            w7052 = 9.0  # File Version
            w7061 = FALSE ("prepend array or string size? (T)")
            w7059 = T21."big-endian, network order" ("byte order (0:big-endian, network order)")
            n1669 = Array Size(array=w7050) -> (size(s)=w7049:i32)
            n1670 = local read "BD 1 Frequency 1 (MHz)"() -> (w7075:dbl)
            n1671 = local read "BD 2 Frequency 1 (MHz)"() -> (w7074:dbl)
            n1672 = local read "BD 1 Frequency 2 (MHz)"() -> (w7073:dbl)
            n1673 = local read "BD 2 Frequency 2 (MHz)"() -> (w7072:dbl)
            n1674 = local read "BD 1 Frequency 3 (MHz)"() -> (w7071:dbl)
            n1675 = local read "BD 2 Frequency 3 (MHz)"() -> (w7070:dbl)
            n1676 = To Double Precision Float(number=w7049) -> (double precision float=w7048:dbl)
            n1677 = local write "Start Saving"(w7046) -> ()
            n1678 = local write "Save Calibration"(w7046) -> ()
            n1679 = Build Array(w7075, w7074, w7073, w7072, w7071, w7070) -> (w7069:dbl[])
            n1680 = case shown="1, Default" w7079 {
              tunnel: w7078 -> [w7123 w7137 w7152 w7189]
              tunnel: w7048 -> [w7128 w7144 w7172 w7208]
              tunnel: w7076 -> [w7127 w7143 w7171 w7207]
              tunnel: [w7124 w7139 w7163 w7199] -> w7067
              tunnel: [w7113 "Cal sets to save" w7153 w7190] -> w7057
              tunnel: w7069 -> [w7125 w7140 w7165 w7201]
              tunnel: "Save APD Data\nwith Trap Data" -> [w7122 _ w7148 w7186]
              tunnel: [w7122 w7133 w7148 w7186] -> w7053
              tunnel: w7052 -> [w7116 w7131 w7146 w7184]
              tunnel: w7051 -> [w7115 _ _ _]
              frame #0 {
                w7119 = 0.0 ("f")
                # "timeseries"
                n1681 = local read "Save ave N"() -> (w7130:dbl)
                n1682 = Multiply(x=w7130, y=w7123) -> (x*y=w7129:dbl)
                n1683 = Boolean To (0,1)(Boolean=w7122) -> (0, 1=w7121:i16)
                n1684 = To Double Precision Float(number=w7121) -> (double precision float=w7120:dbl)
                n1685 = Build Array(w7116, w7123, w7129, w7128, w7127, 0.0 ("f")) -> (w7126:dbl[])
                n1686 = Build Array(w7120, w7119, w7119, w7119, w7119) -> (w7117:dbl[])
                n1687 = Select(t=u32 4000000000, s=w7115, f="N sets to save") -> (s? t:f=w7113:u32)
                n1688 = Build Array (concatenate)(w7126, w7125, w7117) -> (w7124:dbl[])
              }
              frame #1 {
                w7134 = 0.0 ("f")
                w7133 = FALSE ("Save APD Data\nwith Trap Data")
                # "calibration"
                n1689 = Boolean To (0,1)(Boolean=w7133) -> (0, 1=w7136:i16)
                n1690 = To Double Precision Float(number=w7136) -> (double precision float=w7135:dbl)
                n1691 = Build Array(w7135, w7134, w7134, w7134, w7134) -> (w7132:dbl[])
                n1692 = Build Array(w7131, w7137, w7137, w7144, w7143, 1.0 ("t")) -> (w7141:dbl[])
                n1693 = Build Array (concatenate)(w7141, w7140, w7132) -> (w7139:dbl[])
                "Calibrating Trap..." <- TRUE ("Calibrating...")
              }
              frame #2 {
                w7149 = 0.0 ("f")
                # "scan dir (x/y = 0/1)"
                # "cycles/step"
                # "n scans (f/b)"
                # "steps"
                # "freq. range"
                # "AOD raster scan"
                n1694 = local read "Number of F/B Scans (AOD)"() -> (w7157:u16)
                n1695 = local read "Cycles/step (AOD)"() -> (w7159:u64)
                n1696 = local read "Scan Range (MHz)"() -> (w7162:dbl)
                n1697 = local read "Scan steps (AOD)"() -> (w7161:u64)
                n1698 = local read "Scan BD"() -> (w7169:bool)
                n1699 = local read "Save ave N"() -> (w7174:dbl)
                n1700 = Boolean To (0,1)(Boolean=w7169) -> (0, 1=w7168:i16)
                n1701 = To Double Precision Float(number=w7157) -> (double precision float=w7156:dbl)
                n1702 = To Double Precision Float(number=w7161) -> (double precision float=w7160:dbl)
                n1703 = To Double Precision Float(number=w7159) -> (double precision float=w7158:dbl)
                n1704 = To Double Precision Float(number=w7168) -> (double precision float=w7167:dbl)
                n1705 = Boolean To (0,1)(Boolean=w7148) -> (0, 1=w7151:i16)
                n1706 = Multiply(x=w7174, y=w7152) -> (x*y=w7173:dbl)
                n1707 = To Double Precision Float(number=w7151) -> (double precision float=w7150:dbl)
                n1708 = Build Array(w7150, w7149, w7149, w7149, w7149) -> (w7147:dbl[])
                n1709 = local read "N sets should be saved"() -> (w7154:dbl)
                n1710 = Build Array(w7167, w7162, w7160, w7158, w7156) -> (w7164:dbl[])
                n1711 = Build Array(w7146, w7152, w7173, w7172, w7171, 2.0 ("t")) -> (w7166:dbl[])
                n1712 = Round Toward +Infinity(x=w7154) -> (ceil(x): smallest int >= x=w7155:dbl)
                n1713 = Build Array (concatenate)(w7166, w7165, w7147, w7164) -> (w7163:dbl[])
                n1714 = To Unsigned Long Integer(number=w7155) -> (unsigned 32bit integer=w7153:u32)
              }
              frame #3 {
                w7181 = 0.0 ("f")
                # "MCL raster scan"
                n1715 = local read "Number of scans (MCL)"() -> (w7176:u64)
                n1716 = local read "Scan lines (y)"() -> (w7175:u64)
                n1717 = local read "2D or 1D Scan"() -> (w7178:bool)
                n1718 = local read "Scan Range (V)\n(of steps)"() -> (w7198:dbl)
                n1719 = local read "Fast Scan Dir"() -> (w7205:bool)
                n1720 = local read "Cycles/step (MCL)"() -> (w7195:u64)
                n1721 = Select(t=w7175, s=w7178, f=w7176) -> (s? t:f=w7177:u64)
                n1722 = local read "Scan steps (MCL)"() -> (w7197:u64)
                n1723 = Boolean To (0,1)(Boolean=w7178) -> (0, 1=w7180:i16)
                n1724 = local read "Save ave N"() -> (w7210:dbl)
                n1725 = local read "Initial X"() -> (w7183:dbl)
                n1726 = local read "Initial Y"() -> (w7182:dbl)
                n1727 = To Double Precision Float(number=w7180) -> (double precision float=w7179:dbl)
                n1728 = Boolean To (0,1)(Boolean=w7205) -> (0, 1=w7204:i16)
                n1729 = To Double Precision Float(number=w7177) -> (double precision float=w7193:dbl)
                n1730 = To Double Precision Float(number=w7197) -> (double precision float=w7196:dbl)
                n1731 = To Double Precision Float(number=w7195) -> (double precision float=w7194:dbl)
                n1732 = To Double Precision Float(number=w7204) -> (double precision float=w7203:dbl)
                n1733 = Boolean To (0,1)(Boolean=w7186) -> (0, 1=w7188:i16)
                n1734 = Multiply(x=w7210, y=w7189) -> (x*y=w7209:dbl)
                n1735 = To Double Precision Float(number=w7188) -> (double precision float=w7187:dbl)
                n1736 = local read "N sets should be saved (MCL)"() -> (w7191:dbl)
                n1737 = Build Array(w7187, w7179, w7181, w7181, w7181) -> (w7185:dbl[])
                n1738 = Build Array(w7203, w7198, w7196, w7194, w7193, w7183, w7182) -> (w7200:dbl[])
                n1739 = Build Array(w7184, w7189, w7209, w7208, w7207, 3.0 ("t")) -> (w7202:dbl[])
                n1740 = Round Toward +Infinity(x=w7191) -> (ceil(x): smallest int >= x=w7192:dbl)
                n1741 = Build Array (concatenate)(w7202, w7201, w7185, w7200) -> (w7199:dbl[])
                n1742 = To Unsigned Long Integer(number=w7192) -> (unsigned 32bit integer=w7190:u32)
              }
            }
            n1743 = local read "Index"() -> (w7084:dbl)
            n1744 = call "Create new save file.vi"("Insert"="", "Ext"=".dat", "Index In"=w7084) -> ("Path Out"=w7055:path, "Index Out"=w7056:dbl)
            n1745 = local write "Index"(w7056) -> ()
            n1746 = local write "Save file name"(w7055) -> ()
            n1747 = local write "Save index"(w7056) -> ()
            n1748 = Array Size(array=w7067) -> (size(s)=w7068:i32)
            n1749 = Open/Create/Replace File(file path (use dialog)=w7055, operation (0:open)=T22."create", access (0:read/write)=enum16{"read/write", "read-only", "write-only"}."write-only") -> (refnum out=w7081:refnum<file>)  [unwired: 1 in, 4 out]
            n1750 = local write "Saving..."(TRUE ("Saving...")) -> ()
            n1751 = To Double Precision Float(number=w7068) -> (double precision float=w7066:dbl)
            n1752 = String Length(string="Comment (data description)") -> (length=w7064:i32)
            n1753 = To Double Precision Float(number=w7064) -> (double precision float=w7063:dbl)
            n1754 = Deny Access(7:w7081) -> (3:w7080:refnum<file>)  [unwired: 1 in, 2 out]
            n1755 = Build Array (concatenate)(w7066, w7067, w7063) -> (w7065:dbl[])
            n1756 = case "If fluorescence data to be saved" shown="True" w7053 {
              tunnel: w7055 -> [_ w7111]
              tunnel: [refnum<k0> refnum w7091] -> w7054
              frame #0 {
              }
              frame #1 {
                w7090 = 0.0
                n1757 = local read "APD Integration Time (s)"() -> (w7096:dbl)
                n1758 = local read "N APD Samp/step"() -> (w7089:dbl)
                n1759 = Path To String(path=w7111) -> (string=w7110:string)
                n1760 = String Length(string=w7110) -> (length=w7109:i32)
                n1761 = Subtract(x=w7109, y=4) -> (x-y=w7107:i32)
                n1762 = String Subset(string=w7110, length (rest)=w7107) -> (substring=w7106:string)  [unwired: 1 out]
                n1763 = Build Array(w7096, w7089, w7090, w7090, w7090, w7090, w7090, w7090) -> (w7093:dbl[])
                n1764 = Concatenate Strings(w7106, "_fl.dat" ("string")) -> (w7104:string)
                n1765 = Array Size(array=w7093) -> (size(s)=w7095:i32)
                n1766 = String To Path(string=w7104) -> (path=w7100:path)
                n1767 = Open/Create/Replace File(file path (use dialog)=w7100, operation (0:open)=T22."create", access (0:read/write)=enum16{"read/write", "read-only", "write-only"}."write-only") -> (refnum out=w7101:refnum<file>)  [unwired: 1 in, 4 out]
                n1768 = Deny Access(7:w7101) -> (3:w7097:refnum<file>)  [unwired: 1 in, 2 out]
                n1769 = To Double Precision Float(number=w7095) -> (double precision float=w7094:dbl)
                n1770 = Build Array (concatenate)(w7094, w7093) -> (w7092:dbl[])
                n1771 = Write to Binary File(file (use dialog)=w7097, data=w7092, 5:FALSE ("prepend array or string size? (T)"), 9:T21."big-endian, network order" ("byte order (0:big-endian, network order)")) -> (refnum out=w7091:refnum<file>)  [unwired: 1 in, 3 out]
              }
            }
            n1772 = Write to Binary File(file (use dialog)=w7080, data=w7065, 5:w7061, 9:w7059) -> (refnum out=w7062:refnum<file>)  [unwired: 1 in, 3 out]
            n1773 = Write to Binary File(file (use dialog)=w7062, data="Comment (data description)", 5:w7061, 9:w7059) -> (refnum out=w7058:refnum<file>)  [unwired: 1 in, 3 out]
          }
        }
      }
      frame #1 {
        n1774 = local read "Saving..."() -> (w7220:bool)
        n1775 = case shown="True" w7220 {
          tunnel: w7224 -> [_ w7231]
          tunnel: w7223 -> [_ w7245]
          tunnel: w7222 -> [_ w7241]
          tunnel: w7221 -> [_ w7240]
          tunnel: w7219 -> [_ w7239]
          tunnel: w7218 -> [_ w7234]
          tunnel: w7217 -> [_ w7233]
          tunnel: w7216 -> [_ w7232]
          tunnel: w7215 -> [_ w7230]
          tunnel: w7214 -> [_ w7228]
          tunnel: w7213 -> [_ w7227]
          tunnel: w7212 -> [_ w7226]
          tunnel: w7211 -> [_ w7225]
          frame #0 {
          }
          frame #1 {
            n1776 = Multiply(x=w7231, y=w7230) -> (x*y=→"Time (s)":dbl)
            n1777 = Less Or Equal?(x=w7231, y=w7239) -> (x <= y?=w7243:bool)
            n1778 = Or(x="Stop Saving", y="Abort save 2") -> (x .or. y?=w7235:bool)
            n1779 = Not(x=w7235) -> (.not. x?=w7244:bool)
            n1780 = And(x=w7243, y=w7244) -> (x .and. y?=w7242:bool)
            n1781 = case shown="True" w7242 {
              tunnel: w7245 -> [w7250 w7294]
              tunnel: [0.0 w7297] -> w7238
              tunnel: w7231 -> [_ w7295]
              tunnel: w7239 -> [_ w7296]
              tunnel: w7241 -> [_ w7291]
              tunnel: w7240 -> [_ _]
              tunnel: w7234 -> [w7248 w7282]
              tunnel: w7233 -> [w7247 w7283]
              tunnel: w7232 -> [_ w7281]
              tunnel: w7228 -> [_ w7280]
              tunnel: w7227 -> [_ w7253]
              tunnel: w7226 -> [_ w7273]
              tunnel: w7225 -> [_ w7272]
              frame #0 {
                w7246 = FALSE
                n1782 = Close File(refnum=w7250) -> ()  [unwired: 1 in, 2 out]
                n1783 = case shown="True" w7247 {
                  tunnel: w7248 -> [_ w7251]
                  frame #0 {
                  }
                  frame #1 {
                    n1784 = Close File(refnum=w7251) -> ()  [unwired: 1 in, 2 out]
                  }
                }
                n1785 = local write "Raster Scanning..."(w7246) -> ()
                n1786 = local write "Calibrating Trap..."(w7246) -> ()
                n1787 = call <vilib>:"Beep.vi"() -> ()  [unwired: 3 in, 9 out]
                n1788 = local write "Stop Saving"(w7246) -> ()
                "Saving..." <- w7246
              }
              frame #1 {
                n1789 = local read "Calibrating Trap..."() -> (w7284:bool)
                n1790 = case shown="True" w7283 {
                  tunnel: w7282 -> [_ w7301]
                  tunnel: w7281 -> [_ w7300]
                  frame #0 {
                  }
                  frame #1 {
                    n1791 = Write to Binary File(file (use dialog)=w7301, data=w7300, 5:FALSE ("prepend array or string size? (T)"), 9:T21."big-endian, network order" ("byte order (0:big-endian, network order)")) -> ()  [unwired: 1 in, 4 out]
                  }
                }
                n1792 = Greater?(x="Save ave N", y=1.0) -> (0:w7287:bool)
                n1793 = Not(x=w7284) -> (.not. x?=w7286:bool)
                n1794 = And(x=w7286, y=w7287) -> (x .and. y?=w7288:bool)
                n1795 = case shown="True" w7288 {
                  tunnel: w7291 -> [w7304 w7316]
                  tunnel: [w7304 w7308] -> w7285
                  tunnel: "Save ave N" -> [_ w7309]
                  tunnel: w7280 -> [_ w7307]
                  frame #0 {
                  }
                  frame #1 {
                    n1796 = Array Size(array=w7316) -> (size(s)=w7310:i32)
                    n1797 = Array Size(array=w7307) -> (size(s)=w7306:i32)
                    n1798 = Divide(x=w7310, y=w7306) -> (x/y=w7314:dbl)
                    n1799 = Reshape Array(w7316, w7314, w7306) -> (w7315:i16[][])
                    n1800 = Transpose 2D Array(2D array=w7315) -> (transposed array=w7313:i16[][])
                    n1801 = for {
                      tunnel: w7313 -> [w7319] mode=indexing
                      tunnel: [w7318] -> w7305 mode=indexing
                      tunnel: w7309 -> [w7317]
                      n1802 = call "downsample 1D array - I16.vi"("Ave N"=w7317, "Array In"=w7319) -> ("Array Out"=w7318:i16[])  [unwired: 1 out]
                    }
                    n1803 = Transpose 2D Array(2D array=w7305) -> (transposed array=w7312:i16[][])
                    n1804 = Divide(x=w7310, y=w7309) -> (x/y=w7311:dbl)
                    n1805 = Reshape Array(w7312, w7311) -> (w7308:i16[])
                  }
                }
                n1806 = Unbundle By Name(w7272) -> ("Y"=w7277:dbl[])
                n1807 = Unbundle By Name(w7273) -> ("Y"=w7260:dbl[])
                n1808 = Array Size(array=w7260) -> (size(s)=→"size(s) of 1 acq array":i32)
                n1809 = Write to Binary File(file (use dialog)=w7294, data=w7285, 5:FALSE ("prepend array or string size? (T)"), 9:T21."big-endian, network order" ("byte order (0:big-endian, network order)")) -> ()  [unwired: 1 in, 4 out]
                n1810 = feedback #26(w7277) -> (w7276:dbl[])
                n1811 = Build Array (concatenate)(w7276, w7277) -> (w7275:dbl[])
                n1812 = Select(t=w7277, s=w7253, f=w7275) -> (s? t:f=w7274:dbl[])
                "Trap Delta Graph" <- w7274
                n1813 = feedback #27(w7260) -> (w7279:dbl[])
                n1814 = Build Array (concatenate)(w7279, w7260) -> (w7278:dbl[])
                n1815 = Select(t=w7260, s=w7253, f=w7278) -> (s? t:f=w7268:dbl[])
                "APD 1 Graph" <- w7268
                n1816 = Divide(x=w7295, y=w7296) -> (x/y=w7298:dbl)
                n1817 = Array Size(array=w7268) -> (size(s)=w7270:i32)
                "size(s) APD array" <- w7270
                n1818 = Multiply(x=w7298, y=100.0) -> (x*y=w7297:dbl)
                n1819 = Subtract(x=w7270, y="N pts to average") -> (x-y=w7267:i32)
                n1820 = Multiply(x="N pts to average", y=u16 2) -> (x*y=w7269:u16)
                n1821 = Subtract(x=w7270, y=w7269) -> (x-y=w7266:i32)
                n1822 = Array Subset(array=w7268, index=w7267, length="N pts to average") -> (w7264:dbl[])
                n1823 = Array Subset(array=w7268, index=w7266, length="N pts to average") -> (w7263:dbl[])
                n1824 = call <vilib>:"Mean.vi"("X"=w7264) -> ("mean"=w7262:dbl)  [unwired: 1 out]
                n1825 = call <vilib>:"Mean.vi"("X"=w7263) -> ("mean"=w7261:dbl)  [unwired: 1 out]
                n1826 = Subtract(x=w7262, y=w7261) -> (x-y=w7258:dbl)
                "Delta Fl. (Hz)" <- w7258
                n1827 = Initialize Array(w7258, 1 ("dimension size")) -> (w7255:dbl[])
                n1828 = feedback #28(w7255) -> (w7256:dbl[])
                n1829 = Build Array (concatenate)(w7256, w7255) -> (w7254:dbl[])
                n1830 = Select(t=w7255, s=w7253, f=w7254) -> (s? t:f=w7252:dbl[])
                "APD 1 Graph 2" <- w7252
              }
            }
            "Progress" <- w7238
            "Progress 2" <- w7238
          }
        }
      }
    }
    n1831 = local read "AI2 (V)"() -> (w4639:cluster{"Set 1":dbl, "Set 2":dbl})
    n1832 = Bundle By Name(cluster=w4639, "Set 1"=w4638, "Set 2"=w4637) -> (w4635:cluster{"Set 1":dbl, "Set 2":dbl})
    n1833 = Divide(x=w4635, y=3276.7) -> (x/y=w4634:cluster{"Set 1":dbl, "Set 2":dbl})
    n1834 = local write "AI2 (V)"(w4634) -> ()
    n1835 = Divide(x=w4567, y=3276.7) -> (x/y=w4563:T43)
    n1836 = Unbundle By Name(w4563) -> ("Green FB Ch 0"=w4566:dbl, "Green FB Ch 1"=w4565:dbl, "Green FB Ch 2"=w4564:dbl)
    n1837 = Divide(x=w4566, y=w4564) -> (x/y=w4562:dbl)
    n1838 = Divide(x=w4565, y=w4564) -> (x/y=w4561:dbl)
    n1839 = Bundle By Name(cluster=w4563, "Green FB Ch 0"=w4562, "Green FB Ch 1"=w4561) -> (w4541:T43)
    "Green FB Signals (V)" <- w4541
    n1840 = Unbundle By Name(w4541) -> ("Green FB Ch 2"=→"Green FB Plot":dbl)
    n1841 = local read "wait to reset values"() -> (w4643:bool)
    n1842 = Not(x=w4640) -> (.not. x?=w4644:bool)
    n1843 = And(x=w4644, y=w4643) -> (x .and. y?=w4645:bool)
    n1844 = case "Part of MCL raster scanning: returns to initial positions after scan done" shown="True" w4645 {
      tunnel: w4648 -> [w5979 w5986]
      tunnel: [w5979 w5985] -> w4647
      tunnel: w4642 -> [w5978 w5984]
      tunnel: [w5978 w5983] -> w4641
      frame #0 {
      }
      frame #1 {
        w5994 = 10.0 ("y")
        w5993 = 32767.0 ("y")
        # "to return scan values\nafter a synchronous \nAOM scan"
        n1845 = local read "AO2"() -> (w5987:dbl)
        n1846 = local read "AO1"() -> (w5988:dbl)
        n1847 = Multiply(x=w5988, y=w5993) -> (x*y=w5990:dbl)
        n1848 = local write "wait to reset values"(FALSE ("wait to reset values")) -> ()
        n1849 = Multiply(x=w5987, y=w5993) -> (x*y=w5992:dbl)
        n1850 = Divide(x=w5990, y=w5994) -> (x/y=w5989:dbl)
        n1851 = Divide(x=w5992, y=w5994) -> (x/y=w5991:dbl)
        n1852 = To Word Integer(number=w5989) -> (16bit integer=w5995:i16)
        n1853 = To Word Integer(number=w5991) -> (16bit integer=w5996:i16)
        n1854 = local read "Total Counts (ticks)"() -> (w5980:u32)
        n1855 = xnode "Read/Write Control"("FPGA VI Reference In"=w5986, "error in"=w5984, "AO1"=w5995, "AO2"=w5996, "MCL count"=w5980) -> ("FPGA VI Reference Out"=w5985:T15, "error out"=w5983:errorcluster)
        n1856 = local read "Scan Range (V)\n(of steps)"() -> (w5981:dbl)
        n1857 = property on="Scan Range (V)\n(of steps)" class="DigNum (strict)"("Val(Sgnl)"=w5981) -> ()  [unwired: 2 in, 2 out]
      }
    }
    n1858 = node-c288() -> ()  [unwired: 2 out]
  }
  n1859 = for "Create Greyscale map" {
    N: 256 -> [_]
    tunnel: [w7393] -> w188 mode=indexing
    i -> [w7396]
    n1860 = To Unsigned Byte Integer(number=w7396) -> (unsigned 8bit integer=w7392:u8)
    n1861 = Join Numbers(hi=w7392, lo=w7392) -> ((hi.lo)=w7395:u16)
    n1862 = Join Numbers(hi=w7392, lo=w7392) -> ((hi.lo)=w7394:u16)
    n1863 = Join Numbers(hi=w7395, lo=w7394) -> ((hi.lo)=w7393:u32)
  }
  n1864 = node-c288(w12) -> ()  [unwired: 1 out]
  n1865 = node-c288(w16) -> ()  [unwired: 1 out]
  n1866 = node-c288(w14) -> ()  [unwired: 1 out]
  n1867 = node-c288(w10) -> ()  [unwired: 1 out]
  n1868 = VISA Close(VISA resource name=w59, error in (no error)=w58) -> (error out=w63:errorcluster)
  n1869 = call <vilib>:"Simple Error Handler.vi"("error in (no error)"=w63) -> ()  [unwired: 1 in, 8 out]
  n1870 = node-c288(w127) -> ()  [unwired: 1 out]
  n1871 = flat-sequence {
    tunnel: w229 -> [w7400]
    tunnel: w231 -> [w7401]
    tunnel: [w7399] -> w209
    tunnel: [w7398] -> w208
    tunnel: w184 -> [_]
    tunnel: w182 -> [_]
    tunnel: w135 -> [_]
    tunnel: w18 -> [_]
    tunnel: w209 -> [w7459]
    tunnel: w208 -> [w7460]
    frame #0 {
      w7397 = FALSE ("AI to FIFO")
      n1872 = xnode "Read/Write Control"("FPGA VI Reference In"=w7401, "error in"=w7400, "AI to FIFO"=w7397, "APD to FIFO"=w7397) -> ("FPGA VI Reference Out"=w7399:T15, "error out"=w7398:errorcluster)
    }
    frame #1 {
      n1873 = xnode "Close FPGA VI Reference"("FPGA VI Reference In"=w7459, "error in"=w7460) -> ("error out"=→"error out":errorcluster)
    }
  }
